vi "SubLanc.vi"(0 "Target Voltage, V":dbl=1.0 min=-4.0 max=4.0 step=0.1 format="%.4f", 2 "Sweep rate, V/min":dbl=0.1 min=0.0 max=1.0 step=0.01 format="%.4f", 3 "Custom Folder":string, 5 "optional Bias (V)":dbl=1e-08) -> ()   [LabVIEW 2015]
uses:
  <vilib>/Utility/file.llb/Write To Spreadsheet File (DBL).vi
panel:
  out "Numeric 4":i32
  in  "Commutator":bool
  in  "Commute SorceMeter":enum32{"Radio Selection 1", "Radio Selection 2"}(radio)
  out "Numeric 3":i32
  in  "Channel 2 (Vnano3b)":bool
  in  "Channel 1 (Vnano3)":bool
  out "Numeric":i32
  in  "Capacitance (C) and Loss (L)":bool
  in  "Magnetic Field (B)":bool
  in  "Current (Ik3)":bool
  in  "Voltage (Vk3)":bool
  in  "Current (Ik2)":bool
  in  "Voltage (Vk2)":bool
  in  "Channel 2 (Vnano2b)":bool
  in  "Channel 1 (Vnano2)":bool
  in  "Thermometer 1 (T1)":bool=TRUE
  in  "Channel 2 (Vnano1b)":bool
  in  "Channel 1 (Vnano1)":bool
  in  "Current (Ik1)":bool=TRUE
  in  "Voltage (Vk1)":bool
  out "Numeric Current":dbl
  out "Main Keithly2614B address":string="12"
  out "Delib Time delay":i32
  in  "points at each Vg":i32=1
  out "XY Graph":cluster{dbl[], dbl[]}(graph)={[1.0, 0.8, 0.6000000000000001, 0.4000000000000001, 0.20000000000000007, 5.551115123125783e-17, -0.19999999999999996, -0.39999999999999997, -0.6, -0.8, -1.0], [0.03352775, 0.056811, 0.03911575, 0.04330675, -0.02468015, 0.011641600000000002, 0.10151450000000001, 0.12386675000000001, 0.08288825000000001, -0.00186266, -0.038650000000000004]}
  in  "Time btw \npoints, sec":dbl=1.0 format="%.2f"
  out "Array 2":dbl[][](array[numeric])
  out "array for data":dbl[](array[numeric])
  out "Numeric 2":dbl
  out "Array":string[](array[string])
  in  "Addr 1 lock-in oop":bool
  in  "Ring":u16(ring) caption="Y-axis:" items=["Vg", "I", "R1", "R1oop", "Ik1", "T1"]
  out "String":string
  out "Data file:":path
  in  "Set compliance limit, mkA":dbl=0.05 min=0.0 max=1.0 step=0.01 format="%.3f"
  in  "error in (no error)":errorcluster
  in  "Ring 3":u16(ring)=1 items=["1 kOhm", "10 kOhm", "100 kOhm", "1 Mohm", "10 mOhm"]
  in  "Ring 2":u16(ring)=3 items=["1 kOhm", "10 kOhm", "100 kOhm", "1 Mohm", "10 mOhm"]
  in  "Fixed Current mkA":dbl=1.0
  in  "Current is:":T1(radio)
  in  "Ressitance measurements?":bool=TRUE
  in  "Addr 5 lock-in oop":bool
  in  "Addr 4 lock-in oop":bool
  in  "Addr 3 lock-in oop":bool
  in  "Addr 2 lock-in oop":bool
  in  "Addr 5 lock-in":bool
  in  "Addr 4 lock-in":bool
  in  "Addr 3 lock-in":bool=TRUE
  in  "Addr 2 lock-in":bool=TRUE
  in  "Addr 1 lock-in":bool=TRUE
  # "Keithley 2400: address 12"
  # "0"
  # "SourceMeters"
  # "Nanovoltmeters"
  # "Temperature"
  # "Main"
  # "Magnetic Field"
  # "(not recommended, too slow)"
  # "Capacitance & Loss"
  # "(not recommended, too slow)"
  # "(not recommended, too slow)"
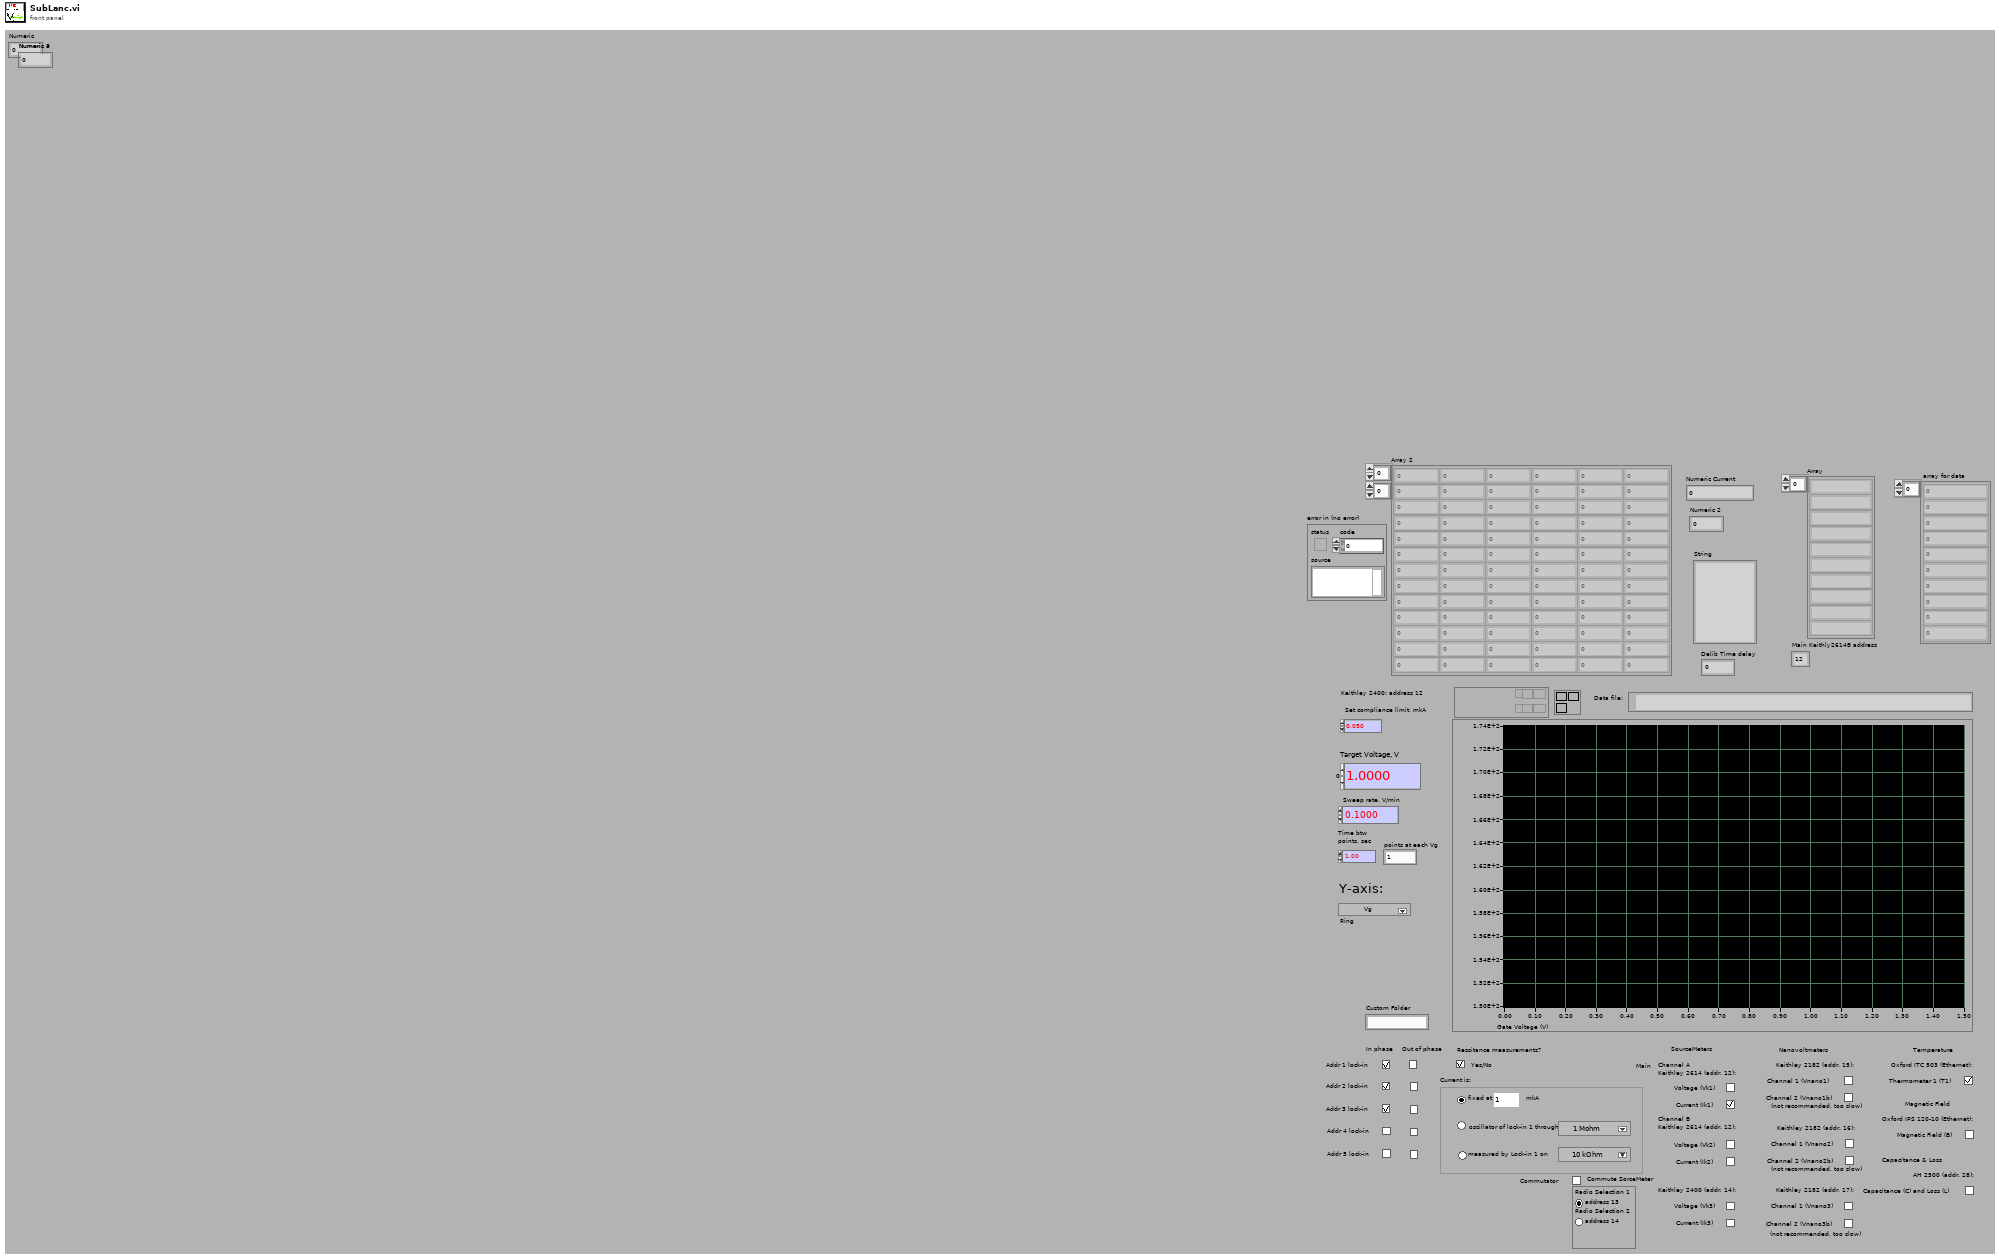
[diagram p1: front panel]
types:
  T1 = enum32{"Radio Selection 1", "Radio Selection 2", "Radio Selection 3"}
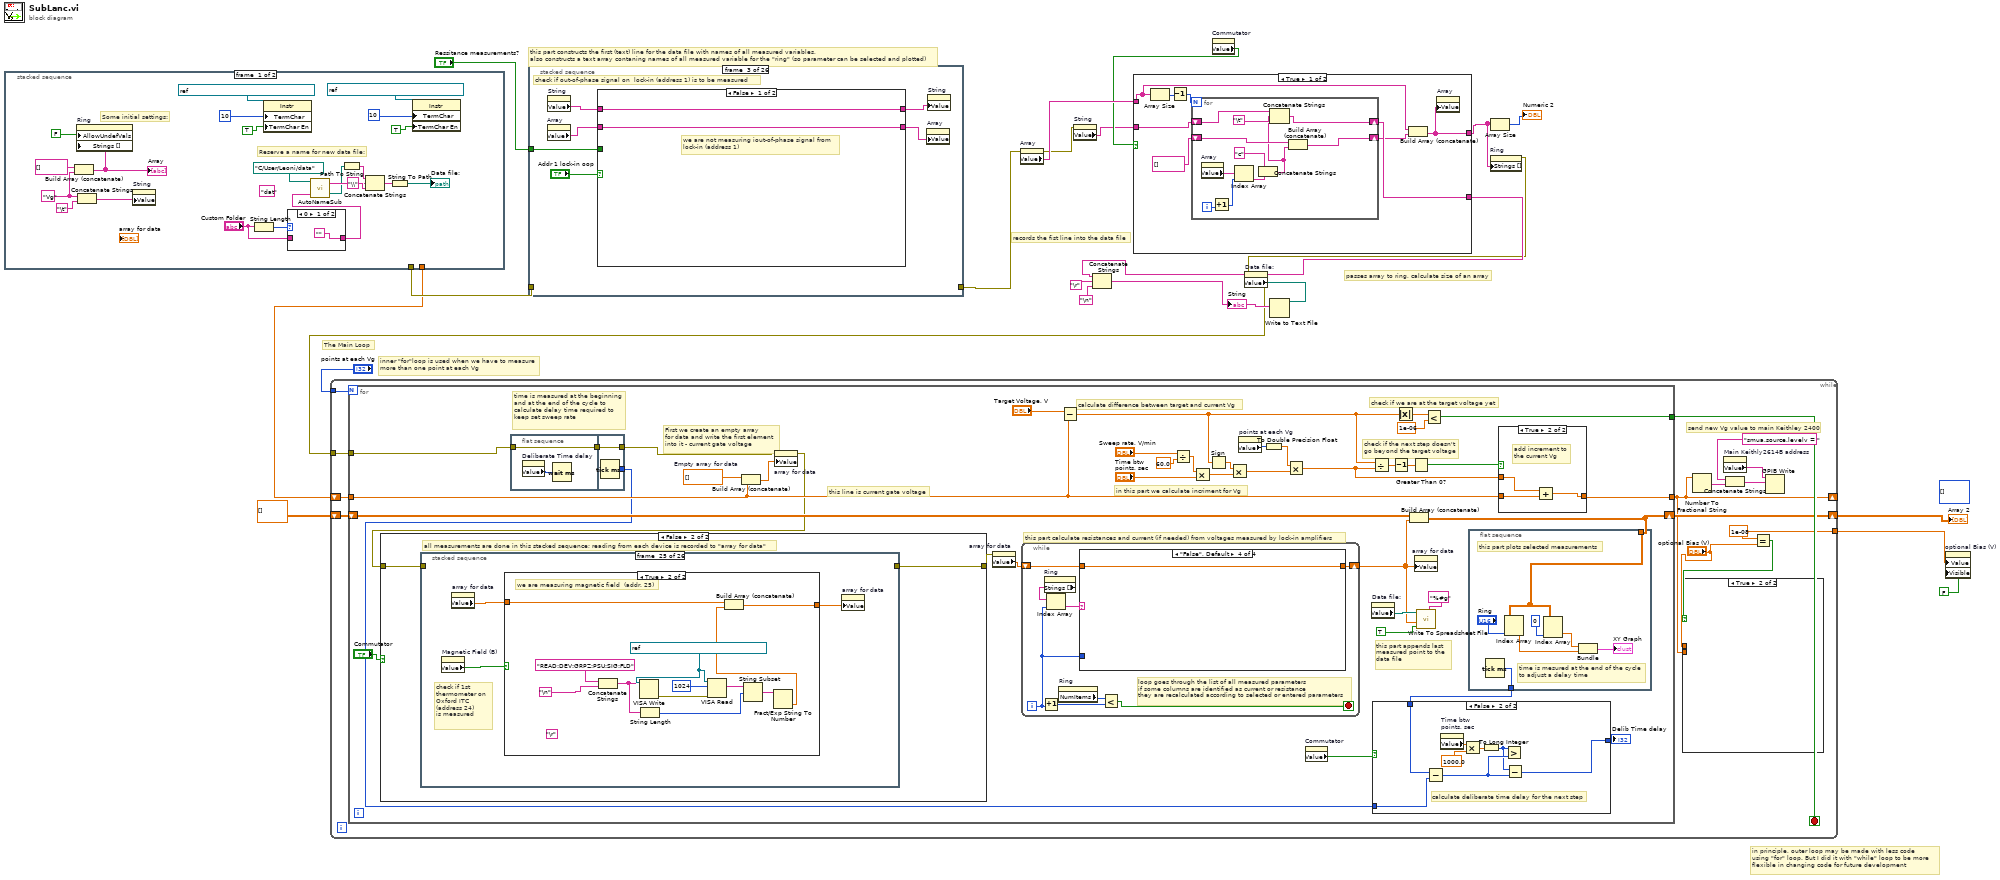
[diagram p0: block diagram]
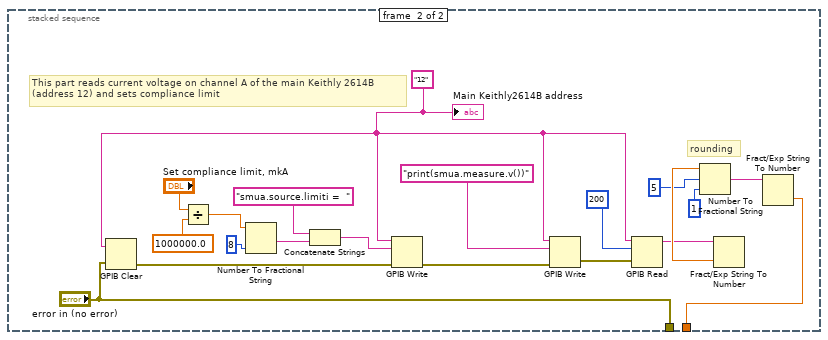
[diagram p4: hidden frame]
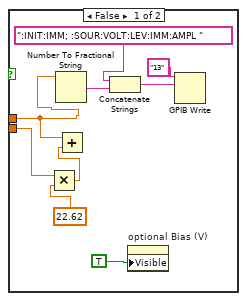
[diagram p5: hidden frame]
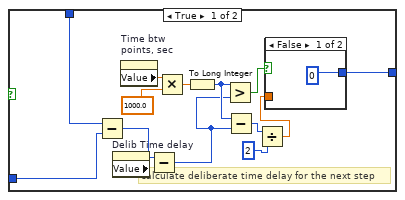
[diagram p6: hidden frame]
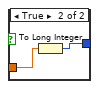
[diagram p7: hidden frame]
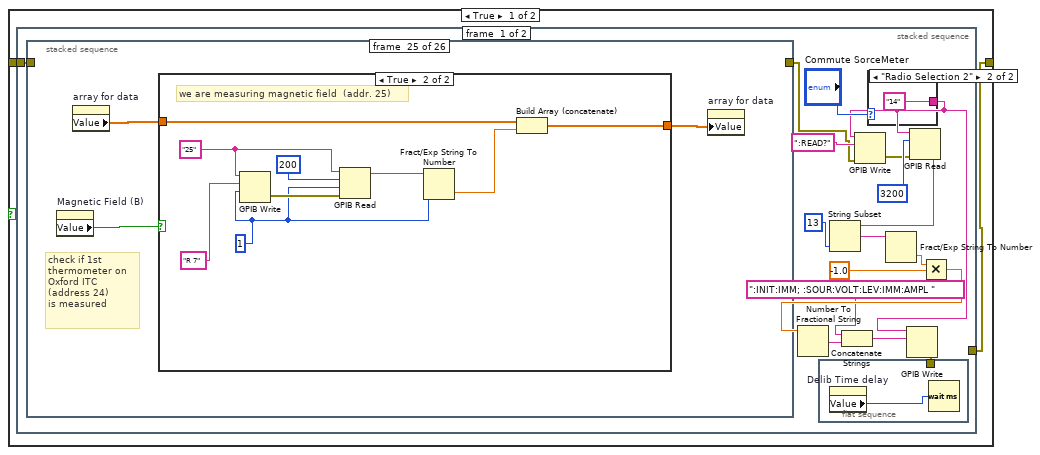
[diagram p8: hidden frame]
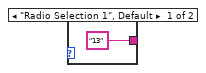
[diagram p9: hidden frame]
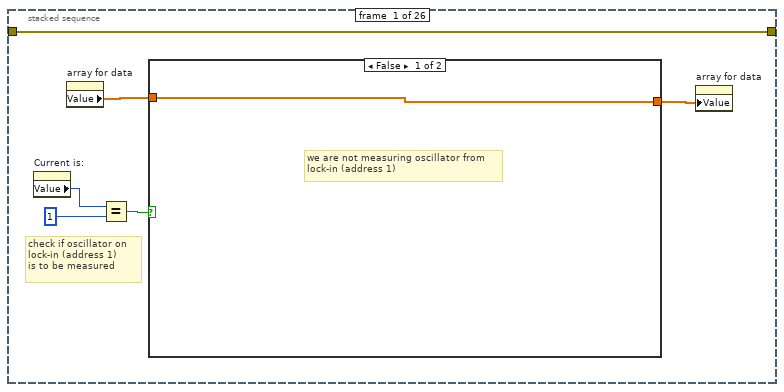
[diagram p10: hidden frame]
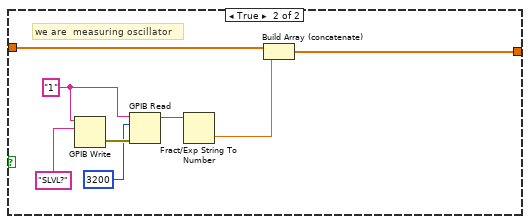
[diagram p11: hidden frame]
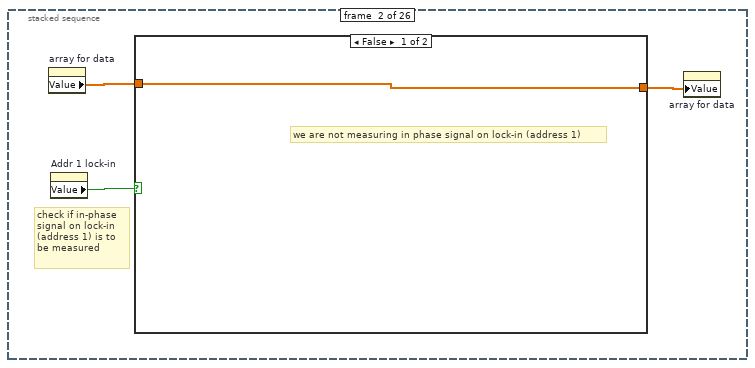
[diagram p12: hidden frame]
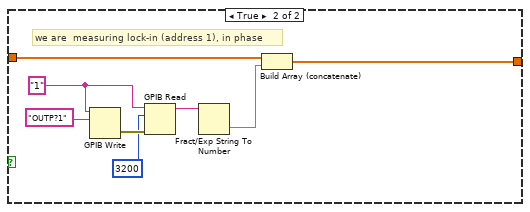
[diagram p13: hidden frame]
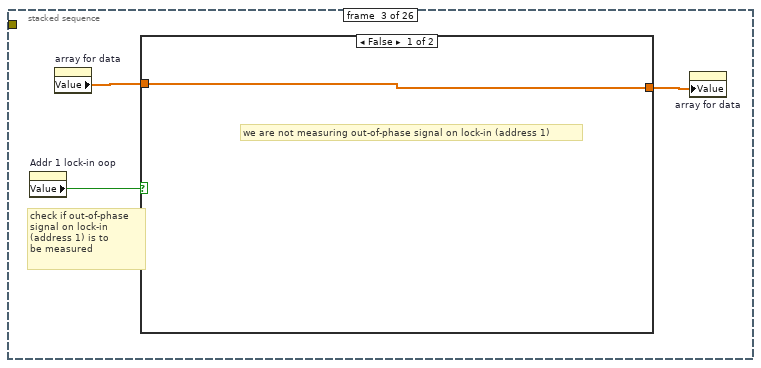
[diagram p14: hidden frame]
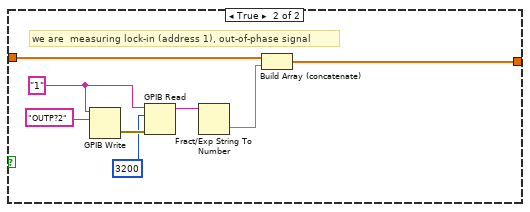
[diagram p15: hidden frame]
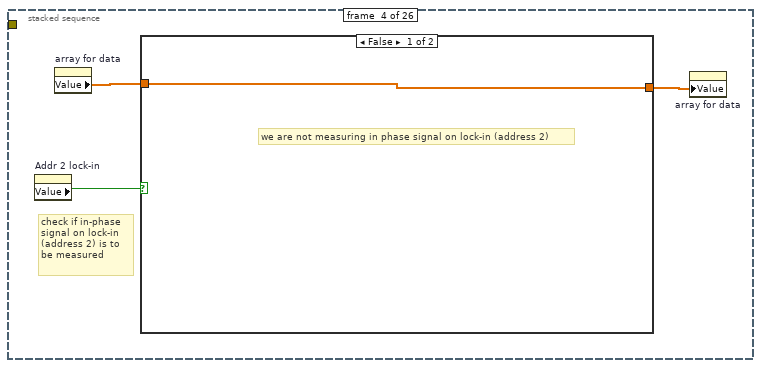
[diagram p16: hidden frame]
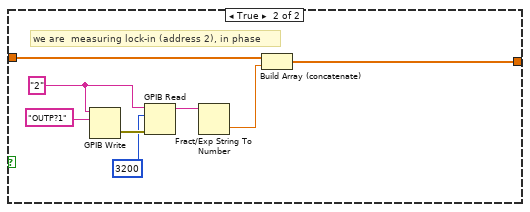
[diagram p17: hidden frame]
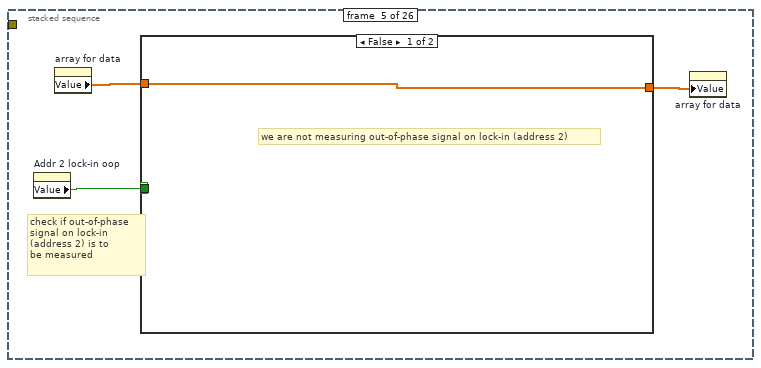
[diagram p18: hidden frame]
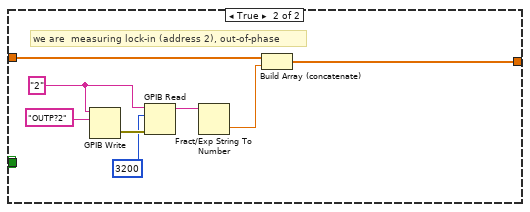
[diagram p19: hidden frame]
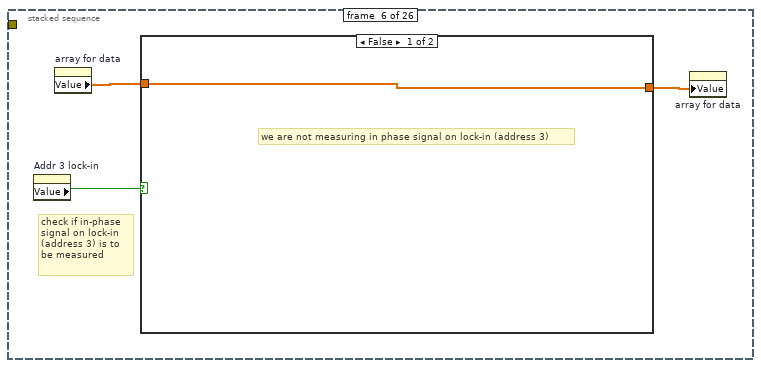
[diagram p20: hidden frame]
diagram:
  (unwired) i32[][] []
  # "passes array to ring, calculate size of an array"
  # "in principle, outer loop may be made with less code\nusing \"for\" loop. But I did it with \"while\" loop to be more \nflexible in changing code for future development"
  # "inner \"for\"loop is used when we have to measure\nmore than one point at each Vg"
  # "The Main Loop"
  # "records the fist line into the data file"
  # "this part constructs the first (text) line for the data file with names of all measured variables,\nalso constructs a text array contaning names of all measured variable for the \"ring\" (so parameter can be selected and plotted)"
  n1 = stacked-sequence {
    tunnel: [_ "error in (no error)"] -> w22
    tunnel: [_ w47] -> w9
    frame #0 {
      (unwired) "dat"
      w34 = "Vg"
      # "Some initial settings:"
      # "Reserve a name for new data file:"
      n2 = Build Array (concatenate)(string[] [], w34) -> (w36:string[])
      "Array" <- w36
      n3 = property on="Ring" class="Ring (strict)"("AllowUndefVals"=FALSE, "Strings []"=w36) -> ()  [unwired: 2 in, 2 out]
      n4 = Concatenate Strings(w34, "\t") -> (w35:string)
      n5 = property on="String" class="Str"("Value"=w35) -> ()  [unwired: 2 in, 2 out]
      n6 = String Length(string="Custom Folder") -> (length=w31:i32)
      n7 = property class="Instr"(reference=refnum<visa-resource-name> "TCPIP0::192.168.128.3::7020::SOCKET" ("VISA resource name"), "TermChar"=10, "TermChar En"=TRUE) -> ()  [unwired: 1 in, 2 out]
      n8 = case shown="0" w31 {
        tunnel: "Custom Folder" -> [_ w46]
        tunnel: ["" w46] -> w29
        frame 0 {
        }
        frame 1, Default {
        }
      }
      n9 = call "AutoNameSub.vi"("Custom Folder"=w29, "User Data Folder"=path "C:/User/Leoni/data") -> ("created path"=w43:path, "String"=w44:string)  [unwired: 1 in]
      n10 = Path To String(path=w43) -> (string=w38:string)
      n11 = Concatenate Strings(w38, "\\", w44) -> (w40:string)
      n12 = String To Path(string=w40) -> (path=→"Data file:":path)
      n13 = property class="Instr"(reference=refnum<visa-resource-name> "TCPIP0::192.168.128.2::7020::SOCKET" ("VISA resource name"), "TermChar"=10, "TermChar En"=TRUE) -> ()  [unwired: 1 in, 2 out]
    }
    frame #1 {
      w54 = "12"
      # "rounding"
      # "This part reads current voltage on channel A of the main Keithly 2614B \n(address 12) and sets compliance limit"
      n14 = GPIB Clear(2:"error in (no error)", 3:w54) -> (0:w59:errorcluster)  [unwired: 1 out]
      n15 = Divide(x="Set compliance limit, mkA", y=1000000.0) -> (x/y=w65:dbl)
      n16 = Number To Fractional String(number=w65, precision (6)=i16 8) -> (F-format string=w61:string)  [unwired: 2 in]
      n17 = Concatenate Strings("smua.source.limiti =  " ("data"), w61) -> (w60:string)
      n18 = GPIB Write(0:w54, 1:w60, 3:w59) -> (6:w55:errorcluster)  [unwired: 2 in, 1 out]
      n19 = GPIB Write(0:w54, 1:"print(smua.measure.v())" ("data"), 3:w55) -> (6:w58:errorcluster)  [unwired: 2 in, 1 out]
      n20 = GPIB Read(0:w54, 1:200 ("byte count"), 3:w58) -> (5:w48:string)  [unwired: 2 in, 2 out]
      n21 = Fract/Exp String To Number(string=w48) -> (number=w52:dbl)  [unwired: 3 in, 1 out]
      n22 = Number To Fractional String(number=w52, width (-)=5, precision (6)=1) -> (F-format string=w49:string)  [unwired: 1 in]
      n23 = Fract/Exp String To Number(string=w49) -> (number=w47:dbl)  [unwired: 3 in, 1 out]
      "Main Keithly2614B address" <- w54
    }
  }
  n24 = stacked-sequence {
    tunnel: "Ressitance measurements?" -> [w74 w89 w113 w136 w154 w172 w190 w208 w226 w244 w262 _ _ _ _ _ _ _ _ _ _ _ _ _ _ _]
    tunnel: w22 -> [_ w86 _ _ _ _ _ _ _ _ _ _ _ _ _ _ _ _ _ _ _ _ _ _ _ _]
    tunnel: [_ w86 _ _ _ _ _ _ _ _ _ _ _ _ _ _ _ _ _ _ _ _ _ _ _ _] -> w19
    frame #0 {
      # "check if oscillator of  lock-in (address 1) is to be measured"
      n25 = property on="Array" class="Arr (strict)"() -> ("Value"=w69:string[])  [unwired: 2 in, 2 out]
      n26 = property on="String" class="Str"() -> ("Value"=w73:string)  [unwired: 2 in, 2 out]
      n27 = Equal?(x="Current is:", y=1) -> (x = y?=w70:bool)
      n28 = case shown="True" w70 {
        tunnel: w74 -> [_ _]
        tunnel: [w76 w77] -> w72
        tunnel: w73 -> [w76 w80]
        tunnel: w69 -> [w75 w79]
        tunnel: [w75 w78] -> w68
        frame False {
          # "we are not measuring oscillator from\nlock-in (address 1)"
        }
        frame True {
          w81 = "I"
          # "we are  measuring oscillator"
          n29 = GPIB Clear(3:"1") -> ()  [unwired: 1 in, 2 out]
          n30 = Concatenate Strings(w80, w81, "\t") -> (w77:string)
          n31 = Build Array (concatenate)(w79, w81) -> (w78:string[])
        }
      }
      n32 = property on="Array" class="Arr (strict)"("Value"=w68) -> ()  [unwired: 2 in, 2 out]
      n33 = property on="String" class="Str"("Value"=w72) -> ()  [unwired: 2 in, 2 out]
    }
    frame #1 {
      # "check if lock-in (address 1) is to be measured"
      n34 = property on="Array" class="Arr (strict)"() -> ("Value"=w85:string[])  [unwired: 2 in, 2 out]
      n35 = property on="String" class="Str"() -> ("Value"=w88:string)  [unwired: 2 in, 2 out]
      n36 = case shown="False" "Addr 1 lock-in" {
        tunnel: w89 -> [_ w100]
        tunnel: [w92 w96] -> w87
        tunnel: w88 -> [w92 w95]
        tunnel: w85 -> [w91 w97]
        tunnel: [w91 w98] -> w84
        frame False {
          # "we are not measuring in phase signal from\nlock-in (address 1)"
        }
        frame True {
          # "are we measuring resistance?"
          n37 = GPIB Clear(3:"1") -> ()  [unwired: 1 in, 2 out]
          n38 = case shown="True" w100 {
            tunnel: ["V1" w102] -> w93
            frame False {
              # "no, we are not measuring resistanse;\nall lock-ins are measuring voltage"
            }
            frame True {
              # "are we measuring current as well?"
              n39 = property on="Current is:" class="RadioBtnsControl (strict)"() -> ("Value"=w104:T1)  [unwired: 2 in, 2 out]
              n40 = Equal?(x=w104, y=2) -> (x = y?=w105:bool)
              n41 = case shown="False" w105 {
                tunnel: ["R1" "I"] -> w102
                frame False {
                  # "no, we are not \nmeasuring current\nby lock-in \n(address 1); \nso this lock-in is \nmeasuring resistance"
                }
                frame True {
                  # "yes, we are measuring \ncurrent by lock-in \n(address 1) as \nvoltage drop on \nknown resistance"
                }
              }
            }
          }
          n42 = Concatenate Strings(w95, w93, "\t") -> (w96:string)
          n43 = Build Array (concatenate)(w97, w93) -> (w98:string[])
        }
      }
      n44 = property on="Array" class="Arr (strict)"("Value"=w84) -> ()  [unwired: 2 in, 2 out]
      n45 = property on="String" class="Str"("Value"=w87) -> ()  [unwired: 2 in, 2 out]
    }
    frame #2 {
      # "check if out-of-phase signal on  lock-in (address 1) is to be measured"
      n46 = property on="Array" class="Arr (strict)"() -> ("Value"=w110:string[])  [unwired: 2 in, 2 out]
      n47 = property on="String" class="Str"() -> ("Value"=w112:string)  [unwired: 2 in, 2 out]
      n48 = case shown="False" "Addr 1 lock-in oop" {
        tunnel: w113 -> [_ w123]
        tunnel: [w115 w119] -> w111
        tunnel: w112 -> [w115 w118]
        tunnel: w110 -> [w114 w120]
        tunnel: [w114 w121] -> w109
        frame False {
          # "we are not measuring iout-of-phase signal from\nlock-in (address 1)"
        }
        frame True {
          # "are we measuring resistance?"
          n49 = GPIB Clear(3:"1") -> ()  [unwired: 1 in, 2 out]
          n50 = case shown="True" w123 {
            tunnel: ["V1oop" w125] -> w116
            frame False {
              # "no, we are not measuring resistance;\nall lock-ins are measuring voltage"
            }
            frame True {
              # "are we measuring out-of-phase current as well?"
              n51 = property on="Current is:" class="RadioBtnsControl (strict)"() -> ("Value"=w127:T1)  [unwired: 2 in, 2 out]
              n52 = Equal?(x=w127, y=2) -> (x = y?=w128:bool)
              n53 = case shown="False" w128 {
                tunnel: ["R1oop" "Ioop"] -> w125
                frame False {
                  # "no, we are not \nmeasuring current\nby lock-in \n(address 1); so this \nlock-in is measuring\nout-of-phase resistance"
                }
                frame True {
                  # "yes, we are measuring \nout-of phase current \nby lock-in (address 1) \nas voltage drop on \nknown resistance"
                }
              }
            }
          }
          n54 = Concatenate Strings(w118, w116, "\t") -> (w119:string)
          n55 = Build Array (concatenate)(w120, w116) -> (w121:string[])
        }
      }
      n56 = property on="Array" class="Arr (strict)"("Value"=w109) -> ()  [unwired: 2 in, 2 out]
      n57 = property on="String" class="Str"("Value"=w111) -> ()  [unwired: 2 in, 2 out]
    }
    frame #3 {
      # "check if in-phase signal on  lock-in (address 2) is to be measured"
      n58 = property on="Array" class="Arr (strict)"() -> ("Value"=w133:string[])  [unwired: 2 in, 2 out]
      n59 = property on="String" class="Str"() -> ("Value"=w135:string)  [unwired: 2 in, 2 out]
      n60 = case shown="False" "Addr 2 lock-in" {
        tunnel: w136 -> [_ w146]
        tunnel: [w138 w142] -> w134
        tunnel: w135 -> [w138 w141]
        tunnel: w133 -> [w137 w143]
        tunnel: [w137 w144] -> w132
        frame False {
          # "we are not measuring in-phase signal from\nlock-in (address 2)"
        }
        frame True {
          # "are we measuring resistance?"
          n61 = GPIB Clear(3:"2") -> ()  [unwired: 1 in, 2 out]
          n62 = case shown="True" w146 {
            tunnel: ["R2" "V2"] -> w139
            frame True {
              # "we are measuring \nresistance by lock-in \n(address 2)"
            }
            frame False, Default {
              # "no, we are not measuring resistance;\nall lock-ins are measuring voltage"
            }
          }
          n63 = Concatenate Strings(w141, w139, "\t") -> (w142:string)
          n64 = Build Array (concatenate)(w143, w139) -> (w144:string[])
        }
      }
      n65 = property on="Array" class="Arr (strict)"("Value"=w132) -> ()  [unwired: 2 in, 2 out]
      n66 = property on="String" class="Str"("Value"=w134) -> ()  [unwired: 2 in, 2 out]
    }
    frame #4 {
      # "check if out-of-phase signal on  lock-in (address 2) is to be measured"
      n67 = property on="Array" class="Arr (strict)"() -> ("Value"=w151:string[])  [unwired: 2 in, 2 out]
      n68 = property on="String" class="Str"() -> ("Value"=w153:string)  [unwired: 2 in, 2 out]
      n69 = case shown="False" "Addr 2 lock-in oop" {
        tunnel: w154 -> [_ w164]
        tunnel: [w156 w160] -> w152
        tunnel: w153 -> [w156 w159]
        tunnel: w151 -> [w155 w161]
        tunnel: [w155 w162] -> w150
        frame False {
          # "we are not measuring out-of-phase signal from\nlock-in (address 2)"
        }
        frame True {
          # "are we measuring resistance?"
          n70 = GPIB Clear(3:"2") -> ()  [unwired: 1 in, 2 out]
          n71 = case shown="True" w164 {
            tunnel: ["R2oop" "V2oop"] -> w157
            frame True {
              # "we are measuring out-of-phase resistance by lock-in (address 2)\n(address 2)"
            }
            frame False, Default {
              # "no, we are not measuring resistance;\nall lock-ins are measuring voltage"
            }
          }
          n72 = Concatenate Strings(w159, w157, "\t") -> (w160:string)
          n73 = Build Array (concatenate)(w161, w157) -> (w162:string[])
        }
      }
      n74 = property on="Array" class="Arr (strict)"("Value"=w150) -> ()  [unwired: 2 in, 2 out]
      n75 = property on="String" class="Str"("Value"=w152) -> ()  [unwired: 2 in, 2 out]
    }
    frame #5 {
      # "check if in-phase signal on  lock-in (address 3) is to be measured"
      n76 = property on="Array" class="Arr (strict)"() -> ("Value"=w169:string[])  [unwired: 2 in, 2 out]
      n77 = property on="String" class="Str"() -> ("Value"=w171:string)  [unwired: 2 in, 2 out]
      n78 = case shown="False" "Addr 3 lock-in" {
        tunnel: w172 -> [_ w182]
        tunnel: [w174 w178] -> w170
        tunnel: w171 -> [w174 w177]
        tunnel: w169 -> [w173 w179]
        tunnel: [w173 w180] -> w168
        frame False {
          # "we are not measuring in-phase signal from\nlock-in (address 3)"
        }
        frame True {
          # "are we measuring resistance?"
          n79 = GPIB Clear(3:"3") -> ()  [unwired: 1 in, 2 out]
          n80 = case shown="True" w182 {
            tunnel: ["R3" "V3"] -> w175
            frame True {
              # "we are measuring \nresistance by lock-in \n(address 3)"
            }
            frame False, Default {
              # "no, we are not measuring resistance;\nall lock-ins are measuring voltage"
            }
          }
          n81 = Concatenate Strings(w177, w175, "\t") -> (w178:string)
          n82 = Build Array (concatenate)(w179, w175) -> (w180:string[])
        }
      }
      n83 = property on="Array" class="Arr (strict)"("Value"=w168) -> ()  [unwired: 2 in, 2 out]
      n84 = property on="String" class="Str"("Value"=w170) -> ()  [unwired: 2 in, 2 out]
    }
    frame #6 {
      # "check if out-of-phase signal on  lock-in (address 3) is to be measured"
      n85 = property on="Array" class="Arr (strict)"() -> ("Value"=w187:string[])  [unwired: 2 in, 2 out]
      n86 = property on="String" class="Str"() -> ("Value"=w189:string)  [unwired: 2 in, 2 out]
      n87 = case shown="False" "Addr 3 lock-in oop" {
        tunnel: w190 -> [_ w200]
        tunnel: [w192 w196] -> w188
        tunnel: w189 -> [w192 w195]
        tunnel: w187 -> [w191 w197]
        tunnel: [w191 w198] -> w186
        frame False {
          # "we are not measuring out-of-phase signal from\nlock-in (address 3)"
        }
        frame True {
          # "are we measuring resistance?"
          n88 = GPIB Clear(3:"3") -> ()  [unwired: 1 in, 2 out]
          n89 = case shown="True" w200 {
            tunnel: ["R3oop" "V3oop"] -> w193
            frame True {
              # "we are measuring out-of-phase resistance by lock-in (address 3)\n(address 2)"
            }
            frame False, Default {
              # "no, we are not measuring resistance;\nall lock-ins are measuring voltage"
            }
          }
          n90 = Concatenate Strings(w195, w193, "\t") -> (w196:string)
          n91 = Build Array (concatenate)(w197, w193) -> (w198:string[])
        }
      }
      n92 = property on="Array" class="Arr (strict)"("Value"=w186) -> ()  [unwired: 2 in, 2 out]
      n93 = property on="String" class="Str"("Value"=w188) -> ()  [unwired: 2 in, 2 out]
    }
    frame #7 {
      # "check if in-phase signal on  lock-in (address 4) is to be measured"
      n94 = property on="Array" class="Arr (strict)"() -> ("Value"=w205:string[])  [unwired: 2 in, 2 out]
      n95 = property on="String" class="Str"() -> ("Value"=w207:string)  [unwired: 2 in, 2 out]
      n96 = case shown="False" "Addr 4 lock-in" {
        tunnel: w208 -> [_ w218]
        tunnel: [w210 w214] -> w206
        tunnel: w207 -> [w210 w213]
        tunnel: w205 -> [w209 w215]
        tunnel: [w209 w216] -> w204
        frame False {
          # "we are not measuring in-phase signal from\nlock-in (address 4)"
        }
        frame True {
          # "are we measuring resistance?"
          n97 = GPIB Clear(3:"4") -> ()  [unwired: 1 in, 2 out]
          n98 = case shown="True" w218 {
            tunnel: ["R4" "V4"] -> w211
            frame True {
              # "we are measuring \nresistance by lock-in \n(address 4)"
            }
            frame False, Default {
              # "no, we are not measuring resistance;\nall lock-ins are measuring voltage"
            }
          }
          n99 = Concatenate Strings(w213, w211, "\t") -> (w214:string)
          n100 = Build Array (concatenate)(w215, w211) -> (w216:string[])
        }
      }
      n101 = property on="Array" class="Arr (strict)"("Value"=w204) -> ()  [unwired: 2 in, 2 out]
      n102 = property on="String" class="Str"("Value"=w206) -> ()  [unwired: 2 in, 2 out]
    }
    frame #8 {
      # "check if out-of-phase signal on  lock-in (address 4) is to be measured"
      n103 = property on="Array" class="Arr (strict)"() -> ("Value"=w223:string[])  [unwired: 2 in, 2 out]
      n104 = property on="String" class="Str"() -> ("Value"=w225:string)  [unwired: 2 in, 2 out]
      n105 = case shown="False" "Addr 4 lock-in oop" {
        tunnel: w226 -> [_ w236]
        tunnel: [w228 w232] -> w224
        tunnel: w225 -> [w228 w231]
        tunnel: w223 -> [w227 w233]
        tunnel: [w227 w234] -> w222
        frame False {
          # "we are not measuring out-of-phase signal from\nlock-in (address 4)"
        }
        frame True {
          # "are we measuring resistance?"
          n106 = GPIB Clear(3:"4") -> ()  [unwired: 1 in, 2 out]
          n107 = case shown="True" w236 {
            tunnel: ["R4oop" "V4oop"] -> w229
            frame True {
              # "we are measuring out-of-phase resistance by lock-in (address 4)\n(address 2)"
            }
            frame False, Default {
              # "no, we are not measuring resistance;\nall lock-ins are measuring voltage"
            }
          }
          n108 = Concatenate Strings(w231, w229, "\t") -> (w232:string)
          n109 = Build Array (concatenate)(w233, w229) -> (w234:string[])
        }
      }
      n110 = property on="Array" class="Arr (strict)"("Value"=w222) -> ()  [unwired: 2 in, 2 out]
      n111 = property on="String" class="Str"("Value"=w224) -> ()  [unwired: 2 in, 2 out]
    }
    frame #9 {
      # "check if in-phase signal on  lock-in (address 5) is to be measured"
      n112 = property on="Array" class="Arr (strict)"() -> ("Value"=w241:string[])  [unwired: 2 in, 2 out]
      n113 = property on="String" class="Str"() -> ("Value"=w243:string)  [unwired: 2 in, 2 out]
      n114 = case shown="False" "Addr 5 lock-in" {
        tunnel: w244 -> [_ w254]
        tunnel: [w246 w250] -> w242
        tunnel: w243 -> [w246 w249]
        tunnel: w241 -> [w245 w251]
        tunnel: [w245 w252] -> w240
        frame False {
          # "we are not measuring in-phase signal from\nlock-in (address 5)"
        }
        frame True {
          # "are we measuring resistance?"
          n115 = GPIB Clear(3:"5") -> ()  [unwired: 1 in, 2 out]
          n116 = case shown="True" w254 {
            tunnel: ["R5" "V5"] -> w247
            frame True {
              # "we are measuring \nresistance by lock-in \n(address 5)"
            }
            frame False, Default {
              # "no, we are not measuring resistance;\nall lock-ins are measuring voltage"
            }
          }
          n117 = Concatenate Strings(w249, w247, "\t") -> (w250:string)
          n118 = Build Array (concatenate)(w251, w247) -> (w252:string[])
        }
      }
      n119 = property on="Array" class="Arr (strict)"("Value"=w240) -> ()  [unwired: 2 in, 2 out]
      n120 = property on="String" class="Str"("Value"=w242) -> ()  [unwired: 2 in, 2 out]
    }
    frame #10 {
      # "check if out-of-phase signal on  lock-in (address 5) is to be measured"
      n121 = property on="Array" class="Arr (strict)"() -> ("Value"=w259:string[])  [unwired: 2 in, 2 out]
      n122 = property on="String" class="Str"() -> ("Value"=w261:string)  [unwired: 2 in, 2 out]
      n123 = case shown="False" "Addr 5 lock-in oop" {
        tunnel: w262 -> [_ w272]
        tunnel: [w264 w268] -> w260
        tunnel: w261 -> [w264 w267]
        tunnel: w259 -> [w263 w269]
        tunnel: [w263 w270] -> w258
        frame False {
          # "we are not measuring out-of-phase signal from\nlock-in (address 5)"
        }
        frame True {
          # "are we measuring resistance?"
          n124 = GPIB Clear(3:"5") -> ()  [unwired: 1 in, 2 out]
          n125 = case shown="True" w272 {
            tunnel: ["R5oop" "V5oop"] -> w265
            frame True {
              # "we are measuring out-of-phase resistance by lock-in (address 5)\n(address 2)"
            }
            frame False, Default {
              # "no, we are not measuring resistance;\nall lock-ins are measuring voltage"
            }
          }
          n126 = Concatenate Strings(w267, w265, "\t") -> (w268:string)
          n127 = Build Array (concatenate)(w269, w265) -> (w270:string[])
        }
      }
      n128 = property on="Array" class="Arr (strict)"("Value"=w258) -> ()  [unwired: 2 in, 2 out]
      n129 = property on="String" class="Str"("Value"=w260) -> ()  [unwired: 2 in, 2 out]
    }
    frame #11 {
      # "check if voltage on main Keithley 2400 (addr. 12) is measured"
      n130 = property on="Array" class="Arr (strict)"() -> ("Value"=w277:string[])  [unwired: 2 in, 2 out]
      n131 = property on="String" class="Str"() -> ("Value"=w279:string)  [unwired: 2 in, 2 out]
      n132 = case shown="False" "Voltage (Vk1)" {
        tunnel: [w281 w285] -> w278
        tunnel: w279 -> [w281 w284]
        tunnel: w277 -> [w280 w286]
        tunnel: [w280 w287] -> w276
        frame False {
          # "no , we aren't measuring voltage \non main Keithley 2400 (addr. 12)"
        }
        frame True {
          w282 = "Vk1"
          # "yes , we are measuring voltage \non main Keithley 2400 (addr. 12)"
          n133 = GPIB Clear(3:"12") -> ()  [unwired: 1 in, 2 out]
          n134 = Concatenate Strings(w284, w282, "\t") -> (w285:string)
          n135 = Build Array (concatenate)(w286, w282) -> (w287:string[])
        }
      }
      n136 = property on="String" class="Str"("Value"=w278) -> ()  [unwired: 2 in, 2 out]
      n137 = property on="Array" class="Arr (strict)"("Value"=w276) -> ()  [unwired: 2 in, 2 out]
    }
    frame #12 {
      # "check if current on main Keithley 2400 (addr. 12) is measured"
      n138 = property on="Array" class="Arr (strict)"() -> ("Value"=w291:string[])  [unwired: 2 in, 2 out]
      n139 = property on="String" class="Str"() -> ("Value"=w293:string)  [unwired: 2 in, 2 out]
      n140 = case shown="True" "Current (Ik1)" {
        tunnel: [w295 w299] -> w292
        tunnel: w293 -> [w295 w298]
        tunnel: w291 -> [w294 w300]
        tunnel: [w294 w301] -> w290
        frame False {
          # "no , we aren't measuring current\non main Keithley 2400 (addr. 12)"
        }
        frame True {
          w296 = "Ik1"
          # "yes , we are measuring current \non main Keithley 2400 (addr. 12)"
          n141 = GPIB Clear(3:"12") -> ()  [unwired: 1 in, 2 out]
          n142 = Concatenate Strings(w298, w296, "\t") -> (w299:string)
          n143 = Build Array (concatenate)(w300, w296) -> (w301:string[])
        }
      }
      n144 = property on="String" class="Str"("Value"=w292) -> ()  [unwired: 2 in, 2 out]
      n145 = property on="Array" class="Arr (strict)"("Value"=w290) -> ()  [unwired: 2 in, 2 out]
    }
    frame #13 {
      # "check if voltage on additional Keithley 2400 (addr. 13) is measured"
      n146 = property on="Array" class="Arr (strict)"() -> ("Value"=w305:string[])  [unwired: 2 in, 2 out]
      n147 = property on="String" class="Str"() -> ("Value"=w307:string)  [unwired: 2 in, 2 out]
      n148 = case shown="False" "Voltage (Vk2)" {
        tunnel: [w309 w313] -> w306
        tunnel: w307 -> [w309 w312]
        tunnel: w305 -> [w308 w314]
        tunnel: [w308 w315] -> w304
        frame False {
          # "no , we aren't measuring voltage \non Keithley 2400 (addr. 13)"
        }
        frame True {
          w310 = "Vk2"
          # "yes , we are measuring voltage \non Keithley 2400 (addr. 13)"
          n149 = GPIB Clear(3:"13") -> ()  [unwired: 1 in, 2 out]
          n150 = Concatenate Strings(w312, w310, "\t") -> (w313:string)
          n151 = Build Array (concatenate)(w314, w310) -> (w315:string[])
        }
      }
      n152 = property on="String" class="Str"("Value"=w306) -> ()  [unwired: 2 in, 2 out]
      n153 = property on="Array" class="Arr (strict)"("Value"=w304) -> ()  [unwired: 2 in, 2 out]
    }
    frame #14 {
      # "check if current on additional Keithley 2400 (addr. 13) is measured"
      n154 = property on="Array" class="Arr (strict)"() -> ("Value"=w319:string[])  [unwired: 2 in, 2 out]
      n155 = property on="String" class="Str"() -> ("Value"=w321:string)  [unwired: 2 in, 2 out]
      n156 = case shown="False" "Current (Ik2)" {
        tunnel: [w323 w327] -> w320
        tunnel: w321 -> [w323 w326]
        tunnel: w319 -> [w322 w328]
        tunnel: [w322 w329] -> w318
        frame False {
          # "no , we aren't measuring current\non Keithley 2400 (addr. 13)"
        }
        frame True {
          w324 = "Ik2"
          # "yes , we are measuring current \non Keithley 2400 (addr. 13)"
          n157 = GPIB Clear(3:"13") -> ()  [unwired: 1 in, 2 out]
          n158 = Concatenate Strings(w326, w324, "\t") -> (w327:string)
          n159 = Build Array (concatenate)(w328, w324) -> (w329:string[])
        }
      }
      n160 = property on="String" class="Str"("Value"=w320) -> ()  [unwired: 2 in, 2 out]
      n161 = property on="Array" class="Arr (strict)"("Value"=w318) -> ()  [unwired: 2 in, 2 out]
    }
    frame #15 {
      # "check if voltage on additional Keithley 2400 (addr. 14) is measured"
      n162 = property on="Array" class="Arr (strict)"() -> ("Value"=w333:string[])  [unwired: 2 in, 2 out]
      n163 = property on="String" class="Str"() -> ("Value"=w335:string)  [unwired: 2 in, 2 out]
      n164 = case shown="False" "Voltage (Vk3)" {
        tunnel: [w337 w341] -> w334
        tunnel: w335 -> [w337 w340]
        tunnel: w333 -> [w336 w342]
        tunnel: [w336 w343] -> w332
        frame False {
          # "no , we aren't measuring voltage \non Keithley 2400 (addr. 14)"
        }
        frame True {
          w338 = "Vk3"
          # "yes , we are measuring voltage \non Keithley 2400 (addr. 14)"
          n165 = GPIB Clear(3:"14") -> ()  [unwired: 1 in, 2 out]
          n166 = Concatenate Strings(w340, w338, "\t") -> (w341:string)
          n167 = Build Array (concatenate)(w342, w338) -> (w343:string[])
        }
      }
      n168 = property on="String" class="Str"("Value"=w334) -> ()  [unwired: 2 in, 2 out]
      n169 = property on="Array" class="Arr (strict)"("Value"=w332) -> ()  [unwired: 2 in, 2 out]
    }
    frame #16 {
      # "check if current on additional Keithley 2400 (addr. 14) is measured"
      n170 = property on="Array" class="Arr (strict)"() -> ("Value"=w347:string[])  [unwired: 2 in, 2 out]
      n171 = property on="String" class="Str"() -> ("Value"=w349:string)  [unwired: 2 in, 2 out]
      n172 = case shown="False" "Current (Ik3)" {
        tunnel: [w351 w355] -> w348
        tunnel: w349 -> [w351 w354]
        tunnel: w347 -> [w350 w356]
        tunnel: [w350 w357] -> w346
        frame False {
          # "no , we aren't measuring current\non Keithley 2400 (addr. 14)"
        }
        frame True {
          w352 = "Ik3"
          # "yes , we are measuring current \non Keithley 2400 (addr. 14)"
          n173 = GPIB Clear(3:"14") -> ()  [unwired: 1 in, 2 out]
          n174 = Concatenate Strings(w354, w352, "\t") -> (w355:string)
          n175 = Build Array (concatenate)(w356, w352) -> (w357:string[])
        }
      }
      n176 = property on="String" class="Str"("Value"=w348) -> ()  [unwired: 2 in, 2 out]
      n177 = property on="Array" class="Arr (strict)"("Value"=w346) -> ()  [unwired: 2 in, 2 out]
    }
    frame #17 {
      # "check if 1st channel of nanovoltmeter Keithley 2182 (addr. 15) is measured"
      n178 = property on="Array" class="Arr (strict)"() -> ("Value"=w361:string[])  [unwired: 2 in, 2 out]
      n179 = property on="String" class="Str"() -> ("Value"=w363:string)  [unwired: 2 in, 2 out]
      n180 = case shown="True" "Channel 1 (Vnano1)" {
        tunnel: [w365 w370] -> w362
        tunnel: w363 -> [w365 w369]
        tunnel: w361 -> [w364 w371]
        tunnel: [w364 w372] -> w360
        frame False {
          # "no , we are not measuring 1st channel\non Keithley 2182 (addr. 15)"
        }
        frame True {
          w367 = "Vnano1"
          # "yes , we are measuring 1st channel\non Keithley 2182 (addr. 15)"
          n181 = GPIB Clear(3:"15") -> ()  [unwired: 1 in, 2 out]
          n182 = Concatenate Strings(w369, w367, "\t") -> (w370:string)
          n183 = Build Array (concatenate)(w371, w367) -> (w372:string[])
        }
      }
      n184 = property on="String" class="Str"("Value"=w362) -> ()  [unwired: 2 in, 2 out]
      n185 = property on="Array" class="Arr (strict)"("Value"=w360) -> ()  [unwired: 2 in, 2 out]
    }
    frame #18 {
      # "check if 2nd channel of nanovoltmeter Keithley 2182 (addr. 15) is measured"
      n186 = property on="Array" class="Arr (strict)"() -> ("Value"=w375:string[])  [unwired: 2 in, 2 out]
      n187 = property on="String" class="Str"() -> ("Value"=w377:string)  [unwired: 2 in, 2 out]
      n188 = case shown="False" "Channel 2 (Vnano1b)" {
        tunnel: [w379 w383] -> w376
        tunnel: w377 -> [w379 w382]
        tunnel: w375 -> [w378 w384]
        tunnel: [w378 w385] -> w374
        frame False {
          # "no , we are not measuring 2nd channel\non Keithley 2182 (addr. 15)"
        }
        frame True {
          w380 = "Vnano1b"
          # "yes , we are measuring 2nd channel\non Keithley 2182 (addr. 15)"
          n189 = GPIB Clear(3:"15") -> ()  [unwired: 1 in, 2 out]
          n190 = Concatenate Strings(w382, w380, "\t") -> (w383:string)
          n191 = Build Array (concatenate)(w384, w380) -> (w385:string[])
        }
      }
      n192 = property on="String" class="Str"("Value"=w376) -> ()  [unwired: 2 in, 2 out]
      n193 = property on="Array" class="Arr (strict)"("Value"=w374) -> ()  [unwired: 2 in, 2 out]
    }
    frame #19 {
      # "check if 1st channel of nanovoltmeter Keithley 2182 (addr. 16) is measured"
      n194 = property on="Array" class="Arr (strict)"() -> ("Value"=w389:string[])  [unwired: 2 in, 2 out]
      n195 = property on="String" class="Str"() -> ("Value"=w391:string)  [unwired: 2 in, 2 out]
      n196 = case shown="True" "Channel 1 (Vnano2)" {
        tunnel: [w393 w398] -> w390
        tunnel: w391 -> [w393 w397]
        tunnel: w389 -> [w392 w399]
        tunnel: [w392 w400] -> w388
        frame False {
          # "no , we are not measuring 1st channel\non Keithley 2182 (addr. 16)"
        }
        frame True {
          w395 = "Vnano2"
          # "yes , we are measuring 1st channel\non Keithley 2182 (addr. 16)"
          n197 = GPIB Clear(3:"16") -> ()  [unwired: 1 in, 2 out]
          n198 = Concatenate Strings(w397, w395, "\t") -> (w398:string)
          n199 = Build Array (concatenate)(w399, w395) -> (w400:string[])
        }
      }
      n200 = property on="String" class="Str"("Value"=w390) -> ()  [unwired: 2 in, 2 out]
      n201 = property on="Array" class="Arr (strict)"("Value"=w388) -> ()  [unwired: 2 in, 2 out]
    }
    frame #20 {
      # "check if 2nd channel of nanovoltmeter Keithley 2182 (addr. 16) is measured"
      n202 = property on="Array" class="Arr (strict)"() -> ("Value"=w403:string[])  [unwired: 2 in, 2 out]
      n203 = property on="String" class="Str"() -> ("Value"=w405:string)  [unwired: 2 in, 2 out]
      n204 = case shown="False" "Channel 2 (Vnano2b)" {
        tunnel: [w407 w411] -> w404
        tunnel: w405 -> [w407 w410]
        tunnel: w403 -> [w406 w412]
        tunnel: [w406 w413] -> w402
        frame False {
          # "no , we are not measuring 2nd channel\non Keithley 2182 (addr. 16)"
        }
        frame True {
          w408 = "Vnano2b"
          # "yes , we are measuring 2nd channel\non Keithley 2182 (addr. 16)"
          n205 = GPIB Clear(3:"16") -> ()  [unwired: 1 in, 2 out]
          n206 = Concatenate Strings(w410, w408, "\t") -> (w411:string)
          n207 = Build Array (concatenate)(w412, w408) -> (w413:string[])
        }
      }
      n208 = property on="String" class="Str"("Value"=w404) -> ()  [unwired: 2 in, 2 out]
      n209 = property on="Array" class="Arr (strict)"("Value"=w402) -> ()  [unwired: 2 in, 2 out]
    }
    frame #21 {
      # "check if 1st channel of nanovoltmeter Keithley 2182 (addr. 17) is measured"
      n210 = property on="Array" class="Arr (strict)"() -> ("Value"=w417:string[])  [unwired: 2 in, 2 out]
      n211 = property on="String" class="Str"() -> ("Value"=w419:string)  [unwired: 2 in, 2 out]
      n212 = case shown="False" "Channel 1 (Vnano3)" {
        tunnel: [w421 w425] -> w418
        tunnel: w419 -> [w421 w424]
        tunnel: w417 -> [w420 w426]
        tunnel: [w420 w427] -> w416
        frame False {
          # "no , we are not measuring 1st channel\non Keithley 2182 (addr. 17)"
        }
        frame True {
          w422 = "Vnano3"
          # "yes , we are measuring 1st channel\non Keithley 2182 (addr. 17)"
          n213 = GPIB Clear(3:"17") -> ()  [unwired: 1 in, 2 out]
          n214 = Concatenate Strings(w424, w422, "\t") -> (w425:string)
          n215 = Build Array (concatenate)(w426, w422) -> (w427:string[])
        }
      }
      n216 = property on="String" class="Str"("Value"=w418) -> ()  [unwired: 2 in, 2 out]
      n217 = property on="Array" class="Arr (strict)"("Value"=w416) -> ()  [unwired: 2 in, 2 out]
    }
    frame #22 {
      # "check if 2nd channel of nanovoltmeter Keithley 2182 (addr. 16) is measured"
      n218 = property on="Array" class="Arr (strict)"() -> ("Value"=w431:string[])  [unwired: 2 in, 2 out]
      n219 = property on="String" class="Str"() -> ("Value"=w433:string)  [unwired: 2 in, 2 out]
      n220 = case shown="False" "Channel 2 (Vnano3b)" {
        tunnel: [w435 w439] -> w432
        tunnel: w433 -> [w435 w438]
        tunnel: w431 -> [w434 w440]
        tunnel: [w434 w441] -> w430
        frame False {
          # "no , we are not measuring 2nd channel\non Keithley 2182 (addr. 17)"
        }
        frame True {
          w436 = "Vnano3b"
          # "yes , we are measuring 2nd channel\non Keithley 2182 (addr. 17)"
          n221 = GPIB Clear(3:"17") -> ()  [unwired: 1 in, 2 out]
          n222 = Concatenate Strings(w438, w436, "\t") -> (w439:string)
          n223 = Build Array (concatenate)(w440, w436) -> (w441:string[])
        }
      }
      n224 = property on="String" class="Str"("Value"=w432) -> ()  [unwired: 2 in, 2 out]
      n225 = property on="Array" class="Arr (strict)"("Value"=w430) -> ()  [unwired: 2 in, 2 out]
    }
    frame #23 {
      # "check if 1st thermometer on Oxford ITC (address 24) is measured"
      n226 = property on="Array" class="Arr (strict)"() -> ("Value"=w445:string[])  [unwired: 2 in, 2 out]
      n227 = property on="String" class="Str"() -> ("Value"=w447:string)  [unwired: 2 in, 2 out]
      n228 = case shown="True" "Thermometer 1 (T1)" {
        tunnel: [w449 w453] -> w446
        tunnel: w447 -> [w449 w452]
        tunnel: w445 -> [w448 w454]
        tunnel: [w448 w455] -> w444
        frame False {
          # "no, we are not measuring temperature\non thermometer 1 (addr. 24)"
        }
        frame True {
          w450 = "T1"
          # "yes, we are measuring temperature,\nthermometer 1 (addr. 24)"
          n229 = GPIB Clear(3:"24") -> ()  [unwired: 1 in, 2 out]
          n230 = Concatenate Strings(w452, w450, "\t") -> (w453:string)
          n231 = Build Array (concatenate)(w454, w450) -> (w455:string[])
        }
      }
      n232 = property on="String" class="Str"("Value"=w446) -> ()  [unwired: 2 in, 2 out]
      n233 = property on="Array" class="Arr (strict)"("Value"=w444) -> ()  [unwired: 2 in, 2 out]
    }
    frame #24 {
      # "check if magnetic field from Oxford IPS 120 (address 25) is measured"
      n234 = property on="Array" class="Arr (strict)"() -> ("Value"=w459:string[])  [unwired: 2 in, 2 out]
      n235 = property on="String" class="Str"() -> ("Value"=w461:string)  [unwired: 2 in, 2 out]
      n236 = case shown="True" "Magnetic Field (B)" {
        tunnel: [w463 w467] -> w460
        tunnel: w461 -> [w463 w466]
        tunnel: w459 -> [w462 w468]
        tunnel: [w462 w469] -> w458
        frame False {
          # "no, we are not measuring magnetic field  (addr. 25)"
        }
        frame True {
          w464 = "B"
          # "yes, we are measuring magnetic field  (addr. 25)"
          n237 = GPIB Clear(3:"25") -> ()  [unwired: 1 in, 2 out]
          n238 = Concatenate Strings(w466, w464, "\t") -> (w467:string)
          n239 = Build Array (concatenate)(w468, w464) -> (w469:string[])
        }
      }
      n240 = property on="String" class="Str"("Value"=w460) -> ()  [unwired: 2 in, 2 out]
      n241 = property on="Array" class="Arr (strict)"("Value"=w458) -> ()  [unwired: 2 in, 2 out]
    }
    frame #25 {
      # "check if capacitance and loss from AH 2500 (address 28) are measured"
      n242 = property on="Array" class="Arr (strict)"() -> ("Value"=w473:string[])  [unwired: 2 in, 2 out]
      n243 = property on="String" class="Str"() -> ("Value"=w475:string)  [unwired: 2 in, 2 out]
      n244 = case shown="False" "Capacitance (C) and Loss (L)" {
        tunnel: [w477 w486] -> w474
        tunnel: w475 -> [w477 w479]
        tunnel: w473 -> [w476 w481]
        tunnel: [w476 w487] -> w472
        frame False {
          # "no, we are not measuring capacitance  (addr. 28)"
        }
        frame True {
          w482 = "C"
          w484 = "L"
          # "yes, we are measuring capacitance and loss  (addr. 28)"
          n245 = GPIB Clear(3:"28") -> ()  [unwired: 1 in, 2 out]
          n246 = Concatenate Strings(w479, w482, "\t") -> (w478:string)
          n247 = Build Array (concatenate)(w481, w482) -> (w480:string[])
          n248 = Concatenate Strings(w478, w484, "\t") -> (w486:string)
          n249 = Build Array (concatenate)(w480, w484) -> (w487:string[])
        }
      }
      n250 = property on="String" class="Str"("Value"=w474) -> ()  [unwired: 2 in, 2 out]
      n251 = property on="Array" class="Arr (strict)"("Value"=w472) -> ()  [unwired: 2 in, 2 out]
    }
  }
  n252 = property on="Array" class="Arr (strict)"(error in=w19) -> (error out=w1:errorcluster, "Value"=w8:string[])  [unwired: 1 in, 1 out]
  n253 = property on="String" class="Str"(error in=w1) -> ("Value"=w4:string)  [unwired: 1 in, 2 out]
  n254 = property on="Commutator" class="Bool (strict)"() -> ("Value"=w7:bool)  [unwired: 2 in, 2 out]
  n255 = case shown="True" w7 {
    tunnel: w8 -> [w491 w509]
    tunnel: [w489 w509] -> w5
    tunnel: w4 -> [w493 w508]
    tunnel: [w492 w508] -> w3
    frame True {
      n256 = Array Size(array=w491) -> (size(s)=w495:i32)
      n257 = Decrement(x=w495) -> (x-1=w494:i32)
      n258 = for {
        N: w494 -> [_]
        shift-right: [w506] -> w490
        shift-left: string[] [] -> [w507]
        shift-right: [w498] -> w492
        shift-left: w493 -> [w499]
        i -> [w503]
        n259 = property on="Array" class="Arr (strict)"() -> ("Value"=w501:string[])  [unwired: 2 in, 2 out]
        n260 = Increment(x=w503) -> (x+1=w502:i32)
        n261 = Index Array(array=w501, index=w502) -> (element=w505:string)
        n262 = Concatenate Strings("c", w505) -> (w497:string)
        n263 = Concatenate Strings(w499, w497, "\t") -> (w498:string)
        n264 = Build Array (concatenate)(w507, w497) -> (w506:string[])
      }
      n265 = Build Array (concatenate)(w491, w490) -> (w489:string[])
      n266 = property on="Array" class="Arr (strict)"("Value"=w489) -> ()  [unwired: 2 in, 2 out]
    }
    frame False {
    }
  }
  n267 = Concatenate Strings(w3, "\r", "\n") -> (w15:string)
  "String" <- w15
  n268 = property on="Ring" class="Ring (strict)"("Strings []"=w5) -> (error out=w2:errorcluster)  [unwired: 2 in, 1 out]
  n269 = property on="Data file:" class="Path"(error in=w2) -> (error out=w14:errorcluster, "Value"=w16:path)  [unwired: 1 in, 1 out]
  n270 = while {
    tunnel: w14 -> [w523]
    shift-right: [w520] -> w13
    shift-left: dbl[][] [] -> [w522]
    shift-right: [w512] -> _
    shift-left: w9 -> [w519]
    tunnel: "points at each Vg" -> [w514]
    tunnel: [w510] -> w11
    stop <- w521 stop-if-true
    w510 = 1e-08
    # "send new Vg value to main Keithley 2400"
    n271 = for {
      N: w514 -> [_]
      tunnel: w523 -> [w539]
      tunnel: [w557] -> w521
      shift-right: [w544] -> w520
      shift-left: w522 -> [w570]
      tunnel: w519 -> [w555]
      tunnel: [w562] -> w512
      w556 = dbl[] []  # Empty array for data
      # "this part appends last\nmeasured point to the \ndata file"
      # "this line is current gate voltage"
      # "First we create an empty array \nfor data and write the first element \ninto it - current gate voltage"
      # "time is measured at the beginning\nand at the end of the cycle to\ncalculate delay time required to\nkeep set sweep rate"
      # "this part calculate resistances and current (if needed) from voltages measured by lock-in amplifiers"
      # "check if the next step doesn't\ngo beyond the target voltage"
      # "calculate difference between target and current Vg"
      # "check if we are at the target voltage yet"
      # "in this part we calculate incriment for Vg"
      n272 = flat-sequence {
        tunnel: w539 -> [w1744]
        tunnel: [w1744] -> w537
        tunnel: [w1746] -> w538
        tunnel: w537 -> [w1746]
        tunnel: [w1745] -> w536
        frame #0 {
          n273 = property on="Deliberate Time delay" class="DigNum (strict)"() -> ("Value"=w1743:i32)  [unwired: 2 in, 2 out]
          n274 = Wait (ms)(milliseconds to wait=w1743) -> ()  [unwired: 1 out]
        }
        frame #1 {
          n275 = Tick Count (ms)() -> (millisecond timer value=w1745:u32)
        }
      }
      n276 = Build Array (concatenate)(w556, w555) -> (w554:dbl[])
      n277 = property on="array for data" class="Arr (strict)"(error in=w538, "Value"=w554) -> (error out=w553:errorcluster)  [unwired: 1 in, 1 out]
      n278 = case shown="False" "Commutator" {
        tunnel: [w597 w1377] -> w571
        tunnel: w553 -> [w598 w1376]
        frame True {
          n279 = stacked-sequence {
            tunnel: w598 -> [w615 w1004]
            tunnel: [_ w989] -> w597
            frame #0 {
              n280 = stacked-sequence {
                tunnel: w615 -> [w619 _ _ _ _ _ _ _ _ _ _ _ _ _ _ _ _ _ _ _ _ _ _ _ _ _]
                tunnel: [w619 _ _ _ _ _ _ _ _ _ _ _ _ _ _ _ _ _ _ _ _ _ _ _ _ _] -> w599
                frame #0 {
                  # "check if oscillator on \nlock-in (address 1)\nis to be measured"
                  n281 = property on="Current is:" class="RadioBtnsControl (strict)"() -> ("Value"=w622:T1)  [unwired: 2 in, 2 out]
                  n282 = property on="array for data" class="Arr (strict)"() -> ("Value"=w621:dbl[])  [unwired: 2 in, 2 out]
                  n283 = Equal?(x=w622, y=1) -> (x = y?=w623:bool)
                  n284 = case shown="False" w623 {
                    tunnel: w621 -> [w625 w633]
                    tunnel: [w625 w632] -> w620
                    frame False {
                      # "we are not measuring oscillator from\nlock-in (address 1)"
                    }
                    frame True {
                      w629 = "1"
                      # "we are  measuring oscillator"
                      n285 = GPIB Write(0:w629, 1:"SLVL?") -> (6:w630:errorcluster)  [unwired: 3 in, 1 out]
                      n286 = GPIB Read(0:w629, 1:3200, 3:w630) -> (5:w627:string)  [unwired: 2 in, 2 out]
                      n287 = Fract/Exp String To Number(string=w627) -> (number=w626:dbl)  [unwired: 3 in, 1 out]
                      n288 = Build Array (concatenate)(w633, w626) -> (w632:dbl[])
                    }
                  }
                  n289 = property on="array for data" class="Arr (strict)"("Value"=w620) -> ()  [unwired: 2 in, 2 out]
                }
                frame #1 {
                  # "check if in-phase\nsignal on lock-in \n(address 1) is to\nbe measured"
                  n290 = property on="array for data" class="Arr (strict)"() -> ("Value"=w636:dbl[])  [unwired: 2 in, 2 out]
                  n291 = property on="Addr 1 lock-in" class="Bool (strict)"() -> ("Value"=w634:bool)  [unwired: 2 in, 2 out]
                  n292 = case shown="False" w634 {
                    tunnel: w636 -> [w637 w645]
                    tunnel: [w637 w644] -> w635
                    frame False {
                      # "we are not measuring in phase signal on lock-in (address 1)"
                    }
                    frame True {
                      w642 = "1"
                      # "we are  measuring lock-in (address 1), in phase"
                      n293 = GPIB Write(0:w642, 1:"OUTP?1") -> (6:w643:errorcluster)  [unwired: 3 in, 1 out]
                      n294 = GPIB Read(0:w642, 1:3200, 3:w643) -> (5:w640:string)  [unwired: 2 in, 2 out]
                      n295 = Fract/Exp String To Number(string=w640) -> (number=w639:dbl)  [unwired: 3 in, 1 out]
                      n296 = Build Array (concatenate)(w645, w639) -> (w644:dbl[])
                    }
                  }
                  n297 = property on="array for data" class="Arr (strict)"("Value"=w635) -> ()  [unwired: 2 in, 2 out]
                }
                frame #2 {
                  # "check if out-of-phase\nsignal on lock-in \n(address 1) is to\nbe measured"
                  n298 = property on="Addr 1 lock-in oop" class="Bool (strict)"() -> ("Value"=w646:bool)  [unwired: 2 in, 2 out]
                  n299 = property on="array for data" class="Arr (strict)"() -> ("Value"=w648:dbl[])  [unwired: 2 in, 2 out]
                  n300 = case shown="False" w646 {
                    tunnel: w648 -> [w649 w657]
                    tunnel: [w649 w656] -> w647
                    frame False {
                      # "we are not measuring out-of-phase signal on lock-in (address 1)"
                    }
                    frame True {
                      w654 = "1"
                      # "we are  measuring lock-in (address 1), out-of-phase signal"
                      n301 = GPIB Write(0:w654, 1:"OUTP?2") -> (6:w655:errorcluster)  [unwired: 3 in, 1 out]
                      n302 = GPIB Read(0:w654, 1:3200, 3:w655) -> (5:w652:string)  [unwired: 2 in, 2 out]
                      n303 = Fract/Exp String To Number(string=w652) -> (number=w651:dbl)  [unwired: 3 in, 1 out]
                      n304 = Build Array (concatenate)(w657, w651) -> (w656:dbl[])
                    }
                  }
                  n305 = property on="array for data" class="Arr (strict)"("Value"=w647) -> ()  [unwired: 2 in, 2 out]
                }
                frame #3 {
                  # "check if in-phase\nsignal on lock-in \n(address 2) is to\nbe measured"
                  n306 = property on="Addr 2 lock-in" class="Bool (strict)"() -> ("Value"=w658:bool)  [unwired: 2 in, 2 out]
                  n307 = property on="array for data" class="Arr (strict)"() -> ("Value"=w660:dbl[])  [unwired: 2 in, 2 out]
                  n308 = case shown="False" w658 {
                    tunnel: w660 -> [w661 w669]
                    tunnel: [w661 w668] -> w659
                    frame False {
                      # "we are not measuring in phase signal on lock-in (address 2)"
                    }
                    frame True {
                      w666 = "2"
                      # "we are  measuring lock-in (address 2), in phase"
                      n309 = GPIB Write(0:w666, 1:"OUTP?1") -> (6:w667:errorcluster)  [unwired: 3 in, 1 out]
                      n310 = GPIB Read(0:w666, 1:3200, 3:w667) -> (5:w664:string)  [unwired: 2 in, 2 out]
                      n311 = Fract/Exp String To Number(string=w664) -> (number=w663:dbl)  [unwired: 3 in, 1 out]
                      n312 = Build Array (concatenate)(w669, w663) -> (w668:dbl[])
                    }
                  }
                  n313 = property on="array for data" class="Arr (strict)"("Value"=w659) -> ()  [unwired: 2 in, 2 out]
                }
                frame #4 {
                  # "check if out-of-phase\nsignal on lock-in \n(address 2) is to\nbe measured"
                  n314 = property on="Addr 2 lock-in oop" class="Bool (strict)"() -> ("Value"=w670:bool)  [unwired: 2 in, 2 out]
                  n315 = property on="array for data" class="Arr (strict)"() -> ("Value"=w672:dbl[])  [unwired: 2 in, 2 out]
                  n316 = case shown="False" w670 {
                    tunnel: w672 -> [w673 w681]
                    tunnel: [w673 w680] -> w671
                    tunnel: w670 -> [_ _]
                    frame False {
                      # "we are not measuring out-of-phase signal on lock-in (address 2)"
                    }
                    frame True {
                      w678 = "2"
                      # "we are  measuring lock-in (address 2), out-of-phase"
                      n317 = GPIB Write(0:w678, 1:"OUTP?2") -> (6:w679:errorcluster)  [unwired: 3 in, 1 out]
                      n318 = GPIB Read(0:w678, 1:3200, 3:w679) -> (5:w676:string)  [unwired: 2 in, 2 out]
                      n319 = Fract/Exp String To Number(string=w676) -> (number=w675:dbl)  [unwired: 3 in, 1 out]
                      n320 = Build Array (concatenate)(w681, w675) -> (w680:dbl[])
                    }
                  }
                  n321 = property on="array for data" class="Arr (strict)"("Value"=w671) -> ()  [unwired: 2 in, 2 out]
                }
                frame #5 {
                  # "check if in-phase\nsignal on lock-in \n(address 3) is to\nbe measured"
                  n322 = property on="Addr 3 lock-in" class="Bool (strict)"() -> ("Value"=w682:bool)  [unwired: 2 in, 2 out]
                  n323 = property on="array for data" class="Arr (strict)"() -> ("Value"=w684:dbl[])  [unwired: 2 in, 2 out]
                  n324 = case shown="False" w682 {
                    tunnel: w684 -> [w685 w693]
                    tunnel: [w685 w692] -> w683
                    frame False {
                      # "we are not measuring in phase signal on lock-in (address 3)"
                    }
                    frame True {
                      w690 = "3"
                      # "we are  measuring lock-in (address 3), in phase"
                      n325 = GPIB Write(0:w690, 1:"OUTP?1") -> (6:w691:errorcluster)  [unwired: 3 in, 1 out]
                      n326 = GPIB Read(0:w690, 1:3200, 3:w691) -> (5:w688:string)  [unwired: 2 in, 2 out]
                      n327 = Fract/Exp String To Number(string=w688) -> (number=w687:dbl)  [unwired: 3 in, 1 out]
                      n328 = Build Array (concatenate)(w693, w687) -> (w692:dbl[])
                    }
                  }
                  n329 = property on="array for data" class="Arr (strict)"("Value"=w683) -> ()  [unwired: 2 in, 2 out]
                }
                frame #6 {
                  # "check if out-of-phase\nsignal on lock-in \n(address 3) is to\nbe measured"
                  n330 = property on="Addr 3 lock-in oop" class="Bool (strict)"() -> ("Value"=w694:bool)  [unwired: 2 in, 2 out]
                  n331 = property on="array for data" class="Arr (strict)"() -> ("Value"=w696:dbl[])  [unwired: 2 in, 2 out]
                  n332 = case shown="False" w694 {
                    tunnel: w696 -> [w697 w705]
                    tunnel: [w697 w704] -> w695
                    frame False {
                      # "we are not measuring out-of-phase signal on lock-in (address 3)"
                    }
                    frame True {
                      w702 = "3"
                      # "we are  measuring lock-in (address 3), out-of-phase"
                      n333 = GPIB Write(0:w702, 1:"OUTP?2") -> (6:w703:errorcluster)  [unwired: 3 in, 1 out]
                      n334 = GPIB Read(0:w702, 1:3200, 3:w703) -> (5:w700:string)  [unwired: 2 in, 2 out]
                      n335 = Fract/Exp String To Number(string=w700) -> (number=w699:dbl)  [unwired: 3 in, 1 out]
                      n336 = Build Array (concatenate)(w705, w699) -> (w704:dbl[])
                    }
                  }
                  n337 = property on="array for data" class="Arr (strict)"("Value"=w695) -> ()  [unwired: 2 in, 2 out]
                }
                frame #7 {
                  # "check if in-phase\nsignal on lock-in \n(address 4) is to\nbe measured"
                  n338 = property on="Addr 4 lock-in" class="Bool (strict)"() -> ("Value"=w706:bool)  [unwired: 2 in, 2 out]
                  n339 = property on="array for data" class="Arr (strict)"() -> ("Value"=w708:dbl[])  [unwired: 2 in, 2 out]
                  n340 = case shown="False" w706 {
                    tunnel: w708 -> [w709 w717]
                    tunnel: [w709 w716] -> w707
                    frame False {
                      # "we are not measuring in phase signal on lock-in (address 4)"
                    }
                    frame True {
                      w714 = "4"
                      # "we are  measuring lock-in (address 4), in phase"
                      n341 = GPIB Write(0:w714, 1:"OUTP?1") -> (6:w715:errorcluster)  [unwired: 3 in, 1 out]
                      n342 = GPIB Read(0:w714, 1:3200, 3:w715) -> (5:w712:string)  [unwired: 2 in, 2 out]
                      n343 = Fract/Exp String To Number(string=w712) -> (number=w711:dbl)  [unwired: 3 in, 1 out]
                      n344 = Build Array (concatenate)(w717, w711) -> (w716:dbl[])
                    }
                  }
                  n345 = property on="array for data" class="Arr (strict)"("Value"=w707) -> ()  [unwired: 2 in, 2 out]
                }
                frame #8 {
                  # "check if out-of-phase\nsignal on lock-in \n(address 4) is to\nbe measured"
                  n346 = property on="Addr 4 lock-in oop" class="Bool (strict)"() -> ("Value"=w718:bool)  [unwired: 2 in, 2 out]
                  n347 = property on="array for data" class="Arr (strict)"() -> ("Value"=w720:dbl[])  [unwired: 2 in, 2 out]
                  n348 = case shown="False" w718 {
                    tunnel: w720 -> [w721 w729]
                    tunnel: [w721 w728] -> w719
                    frame False {
                      # "we are not measuring out-of-phase signal on lock-in (address 4)"
                    }
                    frame True {
                      w726 = "4"
                      # "we are  measuring lock-in (address 4), out-of-phase"
                      n349 = GPIB Write(0:w726, 1:"OUTP?2") -> (6:w727:errorcluster)  [unwired: 3 in, 1 out]
                      n350 = GPIB Read(0:w726, 1:3200, 3:w727) -> (5:w724:string)  [unwired: 2 in, 2 out]
                      n351 = Fract/Exp String To Number(string=w724) -> (number=w723:dbl)  [unwired: 3 in, 1 out]
                      n352 = Build Array (concatenate)(w729, w723) -> (w728:dbl[])
                    }
                  }
                  n353 = property on="array for data" class="Arr (strict)"("Value"=w719) -> ()  [unwired: 2 in, 2 out]
                }
                frame #9 {
                  # "check if in-phase\nsignal on lock-in \n(address 5) is to\nbe measured"
                  n354 = property on="Addr 5 lock-in" class="Bool (strict)"() -> ("Value"=w730:bool)  [unwired: 2 in, 2 out]
                  n355 = property on="array for data" class="Arr (strict)"() -> ("Value"=w732:dbl[])  [unwired: 2 in, 2 out]
                  n356 = case shown="False" w730 {
                    tunnel: w732 -> [w733 w741]
                    tunnel: [w733 w740] -> w731
                    frame False {
                      # "we are not measuring in phase signal on lock-in (address 5)"
                    }
                    frame True {
                      w738 = "5"
                      # "we are  measuring lock-in (address 5), in phase"
                      n357 = GPIB Write(0:w738, 1:"OUTP?1") -> (6:w739:errorcluster)  [unwired: 3 in, 1 out]
                      n358 = GPIB Read(0:w738, 1:3200, 3:w739) -> (5:w736:string)  [unwired: 2 in, 2 out]
                      n359 = Fract/Exp String To Number(string=w736) -> (number=w735:dbl)  [unwired: 3 in, 1 out]
                      n360 = Build Array (concatenate)(w741, w735) -> (w740:dbl[])
                    }
                  }
                  n361 = property on="array for data" class="Arr (strict)"("Value"=w731) -> ()  [unwired: 2 in, 2 out]
                }
                frame #10 {
                  # "check if out-of-phase\nsignal on lock-in \n(address 5) is to\nbe measured"
                  n362 = property on="Addr 5 lock-in oop" class="Bool (strict)"() -> ("Value"=w742:bool)  [unwired: 2 in, 2 out]
                  n363 = property on="array for data" class="Arr (strict)"() -> ("Value"=w744:dbl[])  [unwired: 2 in, 2 out]
                  n364 = case shown="False" w742 {
                    tunnel: w744 -> [w745 w753]
                    tunnel: [w745 w752] -> w743
                    frame False {
                      # "we are not measuring out-of-phase signal on lock-in (address 5)"
                    }
                    frame True {
                      w750 = "5"
                      # "we are  measuring lock-in (address 5), out-of-phase"
                      n365 = GPIB Write(0:w750, 1:"OUTP?2") -> (6:w751:errorcluster)  [unwired: 3 in, 1 out]
                      n366 = GPIB Read(0:w750, 1:3200, 3:w751) -> (5:w748:string)  [unwired: 2 in, 2 out]
                      n367 = Fract/Exp String To Number(string=w748) -> (number=w747:dbl)  [unwired: 3 in, 1 out]
                      n368 = Build Array (concatenate)(w753, w747) -> (w752:dbl[])
                    }
                  }
                  n369 = property on="array for data" class="Arr (strict)"("Value"=w743) -> ()  [unwired: 2 in, 2 out]
                }
                frame #11 {
                  # "check if voltage on \nmain Keithley 2400 \n(addr. 12) is to\nbe measured"
                  n370 = property on="Voltage (Vk1)" class="Bool (strict)"() -> ("Value"=w754:bool)  [unwired: 2 in, 2 out]
                  n371 = property on="array for data" class="Arr (strict)"() -> ("Value"=w756:dbl[])  [unwired: 2 in, 2 out]
                  n372 = case shown="False" w754 {
                    tunnel: w756 -> [w757 w767]
                    tunnel: [w757 w766] -> w755
                    frame False {
                      # "we aren't measuring voltage \non main Keithley 2400 (addr. 12)"
                    }
                    frame True {
                      w764 = "12"
                      # "we are measuring voltage \non main Keithley 2400 (addr. 12)"
                      n373 = GPIB Write(0:w764, 1:":READ?") -> (6:w765:errorcluster)  [unwired: 3 in, 1 out]
                      n374 = GPIB Read(0:w764, 1:3200, 3:w765) -> (5:w760:string)  [unwired: 2 in, 2 out]
                      n375 = String Subset(string=w760, length (rest)=13) -> (substring=w759:string)  [unwired: 1 in]
                      n376 = Fract/Exp String To Number(string=w759) -> (number=w762:dbl)  [unwired: 3 in, 1 out]
                      n377 = Build Array (concatenate)(w767, w762) -> (w766:dbl[])
                    }
                  }
                  n378 = property on="array for data" class="Arr (strict)"("Value"=w755) -> ()  [unwired: 2 in, 2 out]
                }
                frame #12 {
                  # "check if  current on \nmain Keithley 2400 \n(addr. 12) is to\nbe measured"
                  n379 = property on="Current (Ik1)" class="Bool (strict)"() -> ("Value"=w768:bool)  [unwired: 2 in, 2 out]
                  n380 = property on="array for data" class="Arr (strict)"() -> ("Value"=w770:dbl[])  [unwired: 2 in, 2 out]
                  n381 = case shown="True" w768 {
                    tunnel: w770 -> [w771 w782]
                    tunnel: [w771 w781] -> w769
                    frame False {
                      # "we aren't measuring current \non main Keithley 2400 (addr. 12)"
                    }
                    frame True {
                      w779 = "12"
                      # "we are measuring current\non main Keithley 2400 (addr. 12)"
                      n382 = GPIB Write(0:w779, 1:":READ?") -> (6:w780:errorcluster)  [unwired: 3 in, 1 out]
                      n383 = GPIB Read(0:w779, 1:3200, 3:w780) -> (5:w775:string)  [unwired: 2 in, 2 out]
                      n384 = String Subset(string=w775, offset (0)=14, length (rest)=13) -> (substring=w774:string)
                      n385 = Fract/Exp String To Number(string=w774) -> (number=w777:dbl)  [unwired: 3 in, 1 out]
                      n386 = Build Array (concatenate)(w782, w777) -> (w781:dbl[])
                    }
                  }
                  n387 = property on="array for data" class="Arr (strict)"("Value"=w769) -> ()  [unwired: 2 in, 2 out]
                }
                frame #13 {
                  # "check if voltage on \nadd. Keithley 2400 \n(addr. 13) is to\nbe measured"
                  n388 = property on="Voltage (Vk2)" class="Bool (strict)"() -> ("Value"=w783:bool)  [unwired: 2 in, 2 out]
                  n389 = property on="array for data" class="Arr (strict)"() -> ("Value"=w785:dbl[])  [unwired: 2 in, 2 out]
                  n390 = case shown="True" w783 {
                    tunnel: w785 -> [w786 w796]
                    tunnel: [w786 w795] -> w784
                    frame False {
                      # "we aren't measuring voltage \non additional Keithley 2400 (addr. 13)"
                    }
                    frame True {
                      w793 = "13"
                      # "we are measuring voltage \non additional Keithley 2400 (addr. 13)"
                      n391 = GPIB Write(0:w793, 1:":READ?") -> (6:w794:errorcluster)  [unwired: 3 in, 1 out]
                      n392 = GPIB Read(0:w793, 1:3200, 3:w794) -> (5:w789:string)  [unwired: 2 in, 2 out]
                      n393 = String Subset(string=w789, length (rest)=13) -> (substring=w788:string)  [unwired: 1 in]
                      n394 = Fract/Exp String To Number(string=w788) -> (number=w791:dbl)  [unwired: 3 in, 1 out]
                      n395 = Build Array (concatenate)(w796, w791) -> (w795:dbl[])
                    }
                  }
                  n396 = property on="array for data" class="Arr (strict)"("Value"=w784) -> ()  [unwired: 2 in, 2 out]
                }
                frame #14 {
                  # "check if  current on \nadd. Keithley 2400 \n(addr. 13) is to\nbe measured"
                  n397 = property on="Current (Ik2)" class="Bool (strict)"() -> ("Value"=w797:bool)  [unwired: 2 in, 2 out]
                  n398 = property on="array for data" class="Arr (strict)"() -> ("Value"=w799:dbl[])  [unwired: 2 in, 2 out]
                  n399 = case shown="True" w797 {
                    tunnel: w799 -> [w800 w811]
                    tunnel: [w800 w810] -> w798
                    frame False {
                      # "we aren't measuring current \non additional Keithley 2400 (addr. 13)"
                    }
                    frame True {
                      w808 = "13"
                      # "we are measuring current\non additional Keithley 2400 (addr. 13)"
                      n400 = GPIB Write(0:w808, 1:":READ?") -> (6:w809:errorcluster)  [unwired: 3 in, 1 out]
                      n401 = GPIB Read(0:w808, 1:3200, 3:w809) -> (5:w804:string)  [unwired: 2 in, 2 out]
                      n402 = String Subset(string=w804, offset (0)=14, length (rest)=13) -> (substring=w803:string)
                      n403 = Fract/Exp String To Number(string=w803) -> (number=w806:dbl)  [unwired: 3 in, 1 out]
                      n404 = Build Array (concatenate)(w811, w806) -> (w810:dbl[])
                    }
                  }
                  n405 = property on="array for data" class="Arr (strict)"("Value"=w798) -> ()  [unwired: 2 in, 2 out]
                }
                frame #15 {
                  # "check if voltage on \nadd. Keithley 2400 \n(addr. 14) is to\nbe measured"
                  n406 = property on="Voltage (Vk3)" class="Bool (strict)"() -> ("Value"=w812:bool)  [unwired: 2 in, 2 out]
                  n407 = property on="array for data" class="Arr (strict)"() -> ("Value"=w814:dbl[])  [unwired: 2 in, 2 out]
                  n408 = case shown="True" w812 {
                    tunnel: w814 -> [w815 w825]
                    tunnel: [w815 w824] -> w813
                    frame False {
                      # "we aren't measuring voltage \non additional Keithley 2400 (addr. 14)"
                    }
                    frame True {
                      w822 = "14"
                      # "we are measuring voltage \non additional Keithley 2400 (addr. 14)"
                      n409 = GPIB Write(0:w822, 1:":READ?") -> (6:w823:errorcluster)  [unwired: 3 in, 1 out]
                      n410 = GPIB Read(0:w822, 1:3200, 3:w823) -> (5:w818:string)  [unwired: 2 in, 2 out]
                      n411 = String Subset(string=w818, length (rest)=13) -> (substring=w817:string)  [unwired: 1 in]
                      n412 = Fract/Exp String To Number(string=w817) -> (number=w820:dbl)  [unwired: 3 in, 1 out]
                      n413 = Build Array (concatenate)(w825, w820) -> (w824:dbl[])
                    }
                  }
                  n414 = property on="array for data" class="Arr (strict)"("Value"=w813) -> ()  [unwired: 2 in, 2 out]
                }
                frame #16 {
                  # "check if  current on \nadd. Keithley 2400 \n(addr. 14) is to\nbe measured"
                  n415 = property on="Current (Ik3)" class="Bool (strict)"() -> ("Value"=w826:bool)  [unwired: 2 in, 2 out]
                  n416 = property on="array for data" class="Arr (strict)"() -> ("Value"=w828:dbl[])  [unwired: 2 in, 2 out]
                  n417 = case shown="True" w826 {
                    tunnel: w828 -> [w829 w840]
                    tunnel: [w829 w839] -> w827
                    frame False {
                      # "we aren't measuring current \non additional Keithley 2400 (addr. 14)"
                    }
                    frame True {
                      w837 = "14"
                      # "we are measuring current\non additional Keithley 2400 (addr. 14)"
                      n418 = GPIB Write(0:w837, 1:":READ?") -> (6:w838:errorcluster)  [unwired: 3 in, 1 out]
                      n419 = GPIB Read(0:w837, 1:3200, 3:w838) -> (5:w833:string)  [unwired: 2 in, 2 out]
                      n420 = String Subset(string=w833, offset (0)=14, length (rest)=13) -> (substring=w832:string)
                      n421 = Fract/Exp String To Number(string=w832) -> (number=w835:dbl)  [unwired: 3 in, 1 out]
                      n422 = Build Array (concatenate)(w840, w835) -> (w839:dbl[])
                    }
                  }
                  n423 = property on="array for data" class="Arr (strict)"("Value"=w827) -> ()  [unwired: 2 in, 2 out]
                }
                frame #17 {
                  # "check if 1st channel\non Keithley 2182 \n(addr. 15) is to\nbe measured"
                  n424 = property on="Channel 1 (Vnano1)" class="Bool (strict)"() -> ("Value"=w841:bool)  [unwired: 2 in, 2 out]
                  n425 = property on="array for data" class="Arr (strict)"() -> ("Value"=w843:dbl[])  [unwired: 2 in, 2 out]
                  n426 = case shown="True" w841 {
                    tunnel: w843 -> [w844 w852]
                    tunnel: [w844 w851] -> w842
                    frame False {
                      # "we are not measuring 1st channel\non Keithley 2182 (addr. 15)"
                    }
                    frame True {
                      w849 = "15"
                      # "we are measuring 1st channel\non Keithley 2182 (addr. 15)"
                      n427 = GPIB Write(0:w849, 1:":SENSe:DATA:FRES?") -> (6:w850:errorcluster)  [unwired: 3 in, 1 out]
                      n428 = GPIB Read(0:w849, 1:200, 3:w850) -> (5:w845:string)  [unwired: 2 in, 2 out]
                      n429 = Fract/Exp String To Number(string=w845) -> (number=w847:dbl)  [unwired: 3 in, 1 out]
                      n430 = Build Array (concatenate)(w852, w847) -> (w851:dbl[])
                    }
                  }
                  n431 = property on="array for data" class="Arr (strict)"("Value"=w842) -> ()  [unwired: 2 in, 2 out]
                }
                frame #18 {
                  # "check if 2nd channel\non Keithley 2182 \n(addr. 15) is to\nbe measured"
                  n432 = property on="Channel 2 (Vnano1b)" class="Bool (strict)"() -> ("Value"=w853:bool)  [unwired: 2 in, 2 out]
                  n433 = property on="array for data" class="Arr (strict)"() -> ("Value"=w855:dbl[])  [unwired: 2 in, 2 out]
                  n434 = case shown="False" w853 {
                    tunnel: w855 -> [w856 w868]
                    tunnel: [w856 w867] -> w854
                    frame False {
                      # "we are not measuring 1st channel\non Keithley 2182 (addr. 15)"
                    }
                    frame True {
                      w859 = "15"
                      # "switching to channel 2 and then\nback to channel 1"
                      # "we are measuring 2nd channel\non Keithley 2182 (addr. 15)"
                      n435 = GPIB Write(0:w859, 1:":SENSe:CHAN 2") -> (6:w860:errorcluster)  [unwired: 3 in, 1 out]
                      n436 = GPIB Write(0:w859, 1:":SENSe:DATA:FRES?", 3:w860) -> (6:w866:errorcluster)  [unwired: 2 in, 1 out]
                      n437 = GPIB Read(0:w859, 1:200, 3:w866) -> (5:w862:string, 7:w858:errorcluster)  [unwired: 2 in, 1 out]
                      n438 = GPIB Write(0:w859, 1:":SENSe:CHAN 1", 3:w858) -> ()  [unwired: 2 in, 2 out]
                      n439 = Fract/Exp String To Number(string=w862) -> (number=w864:dbl)  [unwired: 3 in, 1 out]
                      n440 = Build Array (concatenate)(w868, w864) -> (w867:dbl[])
                    }
                  }
                  n441 = property on="array for data" class="Arr (strict)"("Value"=w854) -> ()  [unwired: 2 in, 2 out]
                }
                frame #19 {
                  # "check if 1st channel\non Keithley 2182 \n(addr. 16) is to\nbe measured"
                  n442 = property on="Channel 1 (Vnano2)" class="Bool (strict)"() -> ("Value"=w869:bool)  [unwired: 2 in, 2 out]
                  n443 = property on="array for data" class="Arr (strict)"() -> ("Value"=w871:dbl[])  [unwired: 2 in, 2 out]
                  n444 = case shown="True" w869 {
                    tunnel: w871 -> [w872 w880]
                    tunnel: [w872 w879] -> w870
                    frame False {
                      # "we are not measuring 1st channel\non Keithley 2182 (addr. 16)"
                    }
                    frame True {
                      w877 = "16"
                      # "we are measuring 1st channel\non Keithley 2182 (addr. 16)"
                      n445 = GPIB Write(0:w877, 1:":SENSe:DATA:FRES?") -> (6:w878:errorcluster)  [unwired: 3 in, 1 out]
                      n446 = GPIB Read(0:w877, 1:200, 3:w878) -> (5:w873:string)  [unwired: 2 in, 2 out]
                      n447 = Fract/Exp String To Number(string=w873) -> (number=w875:dbl)  [unwired: 3 in, 1 out]
                      n448 = Build Array (concatenate)(w880, w875) -> (w879:dbl[])
                    }
                  }
                  n449 = property on="array for data" class="Arr (strict)"("Value"=w870) -> ()  [unwired: 2 in, 2 out]
                }
                frame #20 {
                  # "check if 2nd channel\non Keithley 2182 \n(addr. 16) is to\nbe measured"
                  n450 = property on="Channel 2 (Vnano2b)" class="Bool (strict)"() -> ("Value"=w881:bool)  [unwired: 2 in, 2 out]
                  n451 = property on="array for data" class="Arr (strict)"() -> ("Value"=w883:dbl[])  [unwired: 2 in, 2 out]
                  n452 = case shown="False" w881 {
                    tunnel: w883 -> [w884 w896]
                    tunnel: [w884 w895] -> w882
                    frame False {
                      # "we are not measuring 1st channel\non Keithley 2182 (addr. 16)"
                    }
                    frame True {
                      w887 = "16"
                      # "switching to channel 2 and then\nback to channel 1"
                      # "we are measuring 2nd channel\non Keithley 2182 (addr. 16)"
                      n453 = GPIB Write(0:w887, 1:":SENSe:CHAN 2") -> (6:w888:errorcluster)  [unwired: 3 in, 1 out]
                      n454 = GPIB Write(0:w887, 1:":SENSe:DATA:FRES?", 3:w888) -> (6:w894:errorcluster)  [unwired: 2 in, 1 out]
                      n455 = GPIB Read(0:w887, 1:200, 3:w894) -> (5:w890:string, 7:w886:errorcluster)  [unwired: 2 in, 1 out]
                      n456 = GPIB Write(0:w887, 1:":SENSe:CHAN 1", 3:w886) -> ()  [unwired: 2 in, 2 out]
                      n457 = Fract/Exp String To Number(string=w890) -> (number=w892:dbl)  [unwired: 3 in, 1 out]
                      n458 = Build Array (concatenate)(w896, w892) -> (w895:dbl[])
                    }
                  }
                  n459 = property on="array for data" class="Arr (strict)"("Value"=w882) -> ()  [unwired: 2 in, 2 out]
                }
                frame #21 {
                  # "check if 1st channel\non Keithley 2182 \n(addr. 17) is to\nbe measured"
                  n460 = property on="Channel 1 (Vnano3)" class="Bool (strict)"() -> ("Value"=w897:bool)  [unwired: 2 in, 2 out]
                  n461 = property on="array for data" class="Arr (strict)"() -> ("Value"=w899:dbl[])  [unwired: 2 in, 2 out]
                  n462 = case shown="True" w897 {
                    tunnel: w899 -> [w900 w908]
                    tunnel: [w900 w907] -> w898
                    frame False {
                      # "we are not measuring 1st channel\non Keithley 2182 (addr. 17)"
                    }
                    frame True {
                      w905 = "17"
                      # "we are measuring 1st channel\non Keithley 2182 (addr. 17)"
                      n463 = GPIB Write(0:w905, 1:":SENSe:DATA:FRES?") -> (6:w906:errorcluster)  [unwired: 3 in, 1 out]
                      n464 = GPIB Read(0:w905, 1:200, 3:w906) -> (5:w901:string)  [unwired: 2 in, 2 out]
                      n465 = Fract/Exp String To Number(string=w901) -> (number=w903:dbl)  [unwired: 3 in, 1 out]
                      n466 = Build Array (concatenate)(w908, w903) -> (w907:dbl[])
                    }
                  }
                  n467 = property on="array for data" class="Arr (strict)"("Value"=w898) -> ()  [unwired: 2 in, 2 out]
                }
                frame #22 {
                  # "check if 2nd channel\non Keithley 2182 \n(addr. 17) is to\nbe measured"
                  n468 = property on="Channel 2 (Vnano3b)" class="Bool (strict)"() -> ("Value"=w909:bool)  [unwired: 2 in, 2 out]
                  n469 = property on="array for data" class="Arr (strict)"() -> ("Value"=w911:dbl[])  [unwired: 2 in, 2 out]
                  n470 = case shown="False" w909 {
                    tunnel: w911 -> [w912 w924]
                    tunnel: [w912 w923] -> w910
                    frame False {
                      # "we are not measuring 1st channel\non Keithley 2182 (addr. 17)"
                    }
                    frame True {
                      w915 = "17"
                      # "switching to channel 2 and then\nback to channel 1"
                      # "we are measuring 2nd channel\non Keithley 2182 (addr. 17)"
                      n471 = GPIB Write(0:w915, 1:":SENSe:CHAN 2") -> (6:w916:errorcluster)  [unwired: 3 in, 1 out]
                      n472 = GPIB Write(0:w915, 1:":SENSe:DATA:FRES?", 3:w916) -> (6:w922:errorcluster)  [unwired: 2 in, 1 out]
                      n473 = GPIB Read(0:w915, 1:200, 3:w922) -> (5:w918:string, 7:w914:errorcluster)  [unwired: 2 in, 1 out]
                      n474 = GPIB Write(0:w915, 1:":SENSe:CHAN 1", 3:w914) -> ()  [unwired: 2 in, 2 out]
                      n475 = Fract/Exp String To Number(string=w918) -> (number=w920:dbl)  [unwired: 3 in, 1 out]
                      n476 = Build Array (concatenate)(w924, w920) -> (w923:dbl[])
                    }
                  }
                  n477 = property on="array for data" class="Arr (strict)"("Value"=w910) -> ()  [unwired: 2 in, 2 out]
                }
                frame #23 {
                  # "check if 1st \nthermometer on \nOxford ITC \n(address 24) \nis measured"
                  n478 = property on="Thermometer 1 (T1)" class="Bool (strict)"() -> ("Value"=w925:bool)  [unwired: 2 in, 2 out]
                  n479 = property on="array for data" class="Arr (strict)"() -> ("Value"=w927:dbl[])  [unwired: 2 in, 2 out]
                  n480 = case shown="True" w925 {
                    tunnel: w927 -> [w928 w937]
                    tunnel: [w928 w936] -> w926
                    frame False {
                      # "we are not measuring temperature on\nthermometer 1 (addr. 24)"
                    }
                    frame True {
                      w929 = 1
                      w934 = "24"
                      # "we are measuring temperature,\nthermometer 1 (addr. 24)"
                      n481 = GPIB Write(0:w934, 1:"R 1", 2:w929) -> (6:w935:errorcluster)  [unwired: 2 in, 1 out]
                      n482 = GPIB Read(0:w934, 1:200, 2:w929, 3:w935) -> (5:w930:string)  [unwired: 1 in, 2 out]
                      n483 = Fract/Exp String To Number(string=w930, offset=w929) -> (number=w932:dbl)  [unwired: 2 in, 1 out]
                      n484 = Build Array (concatenate)(w937, w932) -> (w936:dbl[])
                    }
                  }
                  n485 = property on="array for data" class="Arr (strict)"("Value"=w926) -> ()  [unwired: 2 in, 2 out]
                }
                frame #24 {
                  # "check if 1st \nthermometer on \nOxford ITC \n(address 24) \nis measured"
                  n486 = property on="Magnetic Field (B)" class="Bool (strict)"() -> ("Value"=w938:bool)  [unwired: 2 in, 2 out]
                  n487 = property on="array for data" class="Arr (strict)"() -> ("Value"=w940:dbl[])  [unwired: 2 in, 2 out]
                  n488 = case shown="True" w938 {
                    tunnel: w940 -> [w941 w950]
                    tunnel: [w941 w949] -> w939
                    frame False {
                      # "we are not measuringmagnetic field (addr. 25)"
                    }
                    frame True {
                      w942 = 1
                      w947 = "25"
                      # "we are measuring magnetic field  (addr. 25)"
                      n489 = GPIB Write(0:w947, 1:"R 7", 2:w942) -> (6:w948:errorcluster)  [unwired: 2 in, 1 out]
                      n490 = GPIB Read(0:w947, 1:200, 2:w942, 3:w948) -> (5:w943:string)  [unwired: 1 in, 2 out]
                      n491 = Fract/Exp String To Number(string=w943, offset=w942) -> (number=w945:dbl)  [unwired: 2 in, 1 out]
                      n492 = Build Array (concatenate)(w950, w945) -> (w949:dbl[])
                    }
                  }
                  n493 = property on="array for data" class="Arr (strict)"("Value"=w939) -> ()  [unwired: 2 in, 2 out]
                }
                frame #25 {
                  # "check if capacitance\nand loss (address 28)\nare measured"
                  n494 = property on="Capacitance (C) and Loss (L)" class="Bool (strict)"() -> ("Value"=w951:bool)  [unwired: 2 in, 2 out]
                  n495 = property on="array for data" class="Arr (strict)"() -> ("Value"=w953:dbl[])  [unwired: 2 in, 2 out]
                  n496 = case shown="False" w951 {
                    tunnel: w953 -> [w954 w960]
                    tunnel: [w954 w956] -> w952
                    frame False {
                      # "we are not measuringmagnetic capacitance (addr. 28)"
                    }
                    frame True {
                      # "we are measuring capacitance and loss  (addr. 28)"
                      n497 = stacked-sequence {
                        seq-local: [w962 _ _] -> [_ _ w985]
                        tunnel: [_ _ w979] -> w955
                        tunnel: [_ _ w980] -> w958
                        tunnel: "28" ("data") -> [w961 w965 w974]
                        frame #0 {
                          n498 = GPIB Write(0:w961, 1:"SINGLE" ("data"), 2:i16 0 ("mode (0)")) -> (6:w962:errorcluster)  [unwired: 2 in, 1 out]
                        }
                        frame #1 {
                          n499 = while {
                            tunnel: w965 -> [w966]
                            i -> [w967]
                            stop <- w969 continue-if-true
                            n500 = GPIB Serial Poll(0:w966) -> (2:w971:i16)  [unwired: 1 in, 2 out]
                            n501 = Less?(x=w971, y=i16 128) -> (x < y?=w969:bool)
                            n502 = Wait (ms)(milliseconds to wait=u32 50) -> ()  [unwired: 1 out]
                            "Numeric" <- w967
                          }
                        }
                        frame #2 {
                          w972 = i16 2 ("mode (0)")
                          n503 = GPIB Read(0:w974, 1:200 ("byte count"), 2:i16 2 ("mode (0)"), 3:w985) -> (5:w978:string)  [unwired: 1 in, 2 out]
                          n504 = Match Pattern(string=w978, regular expression="C=") -> (after substring=w977:string)  [unwired: 1 in, 3 out]
                          n505 = Match Pattern(string=w977, regular expression="PF L=") -> (after substring=w975:string)  [unwired: 1 in, 3 out]
                          n506 = Search/Split String(string=w977, search string/char (-)=" ", offset (0)=w972) -> (substring before match=w982:string)  [unwired: 2 out]
                          n507 = Search/Split String(string=w975, search string/char (-)=" ", offset (0)=w972) -> (substring before match=w981:string)  [unwired: 2 out]
                          n508 = Fract/Exp String To Number(string=w981) -> (number=w979:dbl)  [unwired: 3 in, 1 out]
                          n509 = Fract/Exp String To Number(string=w982) -> (number=w980:dbl)  [unwired: 3 in, 1 out]
                        }
                      }
                      n510 = Build Array (concatenate)(w960, w958) -> (w957:dbl[])
                      n511 = Build Array (concatenate)(w957, w955) -> (w956:dbl[])
                    }
                  }
                  n512 = property on="array for data" class="Arr (strict)"("Value"=w952) -> ()  [unwired: 2 in, 2 out]
                }
              }
              n513 = flat-sequence {
                tunnel: w600 -> [_]
                frame #0 {
                  n514 = property on="Delib Time delay" class="DigNum (strict)"() -> ("Value"=w616:i32)  [unwired: 2 in, 2 out]
                  n515 = Wait (ms)(milliseconds to wait=w616) -> ()  [unwired: 1 out]
                }
              }
              n516 = case shown="\"Radio Selection 2\"" "Commute SorceMeter" {
                tunnel: ["13" "14"] -> w601
                frame "Radio Selection 1", Default {
                }
                frame "Radio Selection 2" {
                }
              }
              n517 = GPIB Write(0:w601, 1:":READ?", 3:w599) -> (6:w602:errorcluster)  [unwired: 2 in, 1 out]
              n518 = GPIB Read(0:w601, 1:3200, 3:w602) -> (5:w605:string)  [unwired: 2 in, 2 out]
              n519 = String Subset(string=w605, length (rest)=13) -> (substring=w606:string)  [unwired: 1 in]
              n520 = Fract/Exp String To Number(string=w606) -> (number=w608:dbl)  [unwired: 3 in, 1 out]
              n521 = Multiply(x=w608, y=-1.0) -> (x*y=w613:dbl)
              n522 = Number To Fractional String(number=w613) -> (F-format string=w610:string)  [unwired: 3 in]
              n523 = Concatenate Strings(":INIT:IMM; :SOUR:VOLT:LEV:IMM:AMPL " ("data"), w610) -> (w611:string)
              n524 = GPIB Write(0:w601, 1:w611) -> (6:w600:errorcluster)  [unwired: 3 in, 1 out]
            }
            frame #1 {
              n525 = stacked-sequence {
                tunnel: w1004 -> [w1007 _ _ _ _ _ _ _ _ _ _ _ _ _ _ _ _ _ _ _ _ _ _ _ _ _]
                tunnel: [w1007 _ _ _ _ _ _ _ _ _ _ _ _ _ _ _ _ _ _ _ _ _ _ _ _ _] -> w990
                frame #0 {
                  # "check if oscillator on \nlock-in (address 1)\nis to be measured"
                  n526 = property on="Current is:" class="RadioBtnsControl (strict)"() -> ("Value"=w1010:T1)  [unwired: 2 in, 2 out]
                  n527 = property on="array for data" class="Arr (strict)"() -> ("Value"=w1009:dbl[])  [unwired: 2 in, 2 out]
                  n528 = Equal?(x=w1010, y=1) -> (x = y?=w1011:bool)
                  n529 = case shown="False" w1011 {
                    tunnel: w1009 -> [w1013 w1021]
                    tunnel: [w1013 w1020] -> w1008
                    frame False {
                      # "we are not measuring oscillator from\nlock-in (address 1)"
                    }
                    frame True {
                      w1017 = "1"
                      # "we are  measuring oscillator"
                      n530 = GPIB Write(0:w1017, 1:"SLVL?") -> (6:w1018:errorcluster)  [unwired: 3 in, 1 out]
                      n531 = GPIB Read(0:w1017, 1:3200, 3:w1018) -> (5:w1015:string)  [unwired: 2 in, 2 out]
                      n532 = Fract/Exp String To Number(string=w1015) -> (number=w1014:dbl)  [unwired: 3 in, 1 out]
                      n533 = Build Array (concatenate)(w1021, w1014) -> (w1020:dbl[])
                    }
                  }
                  n534 = property on="array for data" class="Arr (strict)"("Value"=w1008) -> ()  [unwired: 2 in, 2 out]
                }
                frame #1 {
                  # "check if in-phase\nsignal on lock-in \n(address 1) is to\nbe measured"
                  n535 = property on="array for data" class="Arr (strict)"() -> ("Value"=w1024:dbl[])  [unwired: 2 in, 2 out]
                  n536 = property on="Addr 1 lock-in" class="Bool (strict)"() -> ("Value"=w1022:bool)  [unwired: 2 in, 2 out]
                  n537 = case shown="True" w1022 {
                    tunnel: w1024 -> [w1025 w1033]
                    tunnel: [w1025 w1032] -> w1023
                    frame False {
                      # "we are not measuring in phase signal on lock-in (address 1)"
                    }
                    frame True {
                      w1030 = "1"
                      # "we are  measuring lock-in (address 1), in phase"
                      n538 = GPIB Write(0:w1030, 1:"OUTP?1") -> (6:w1031:errorcluster)  [unwired: 3 in, 1 out]
                      n539 = GPIB Read(0:w1030, 1:3200, 3:w1031) -> (5:w1028:string)  [unwired: 2 in, 2 out]
                      n540 = Fract/Exp String To Number(string=w1028) -> (number=w1027:dbl)  [unwired: 3 in, 1 out]
                      n541 = Build Array (concatenate)(w1033, w1027) -> (w1032:dbl[])
                    }
                  }
                  n542 = property on="array for data" class="Arr (strict)"("Value"=w1023) -> ()  [unwired: 2 in, 2 out]
                }
                frame #2 {
                  # "check if out-of-phase\nsignal on lock-in \n(address 1) is to\nbe measured"
                  n543 = property on="Addr 1 lock-in oop" class="Bool (strict)"() -> ("Value"=w1034:bool)  [unwired: 2 in, 2 out]
                  n544 = property on="array for data" class="Arr (strict)"() -> ("Value"=w1036:dbl[])  [unwired: 2 in, 2 out]
                  n545 = case shown="True" w1034 {
                    tunnel: w1036 -> [w1037 w1045]
                    tunnel: [w1037 w1044] -> w1035
                    frame False {
                      # "we are not measuring out-of-phase signal on lock-in (address 1)"
                    }
                    frame True {
                      w1042 = "1"
                      # "we are  measuring lock-in (address 1), out-of-phase signal"
                      n546 = GPIB Write(0:w1042, 1:"OUTP?2") -> (6:w1043:errorcluster)  [unwired: 3 in, 1 out]
                      n547 = GPIB Read(0:w1042, 1:3200, 3:w1043) -> (5:w1040:string)  [unwired: 2 in, 2 out]
                      n548 = Fract/Exp String To Number(string=w1040) -> (number=w1039:dbl)  [unwired: 3 in, 1 out]
                      n549 = Build Array (concatenate)(w1045, w1039) -> (w1044:dbl[])
                    }
                  }
                  n550 = property on="array for data" class="Arr (strict)"("Value"=w1035) -> ()  [unwired: 2 in, 2 out]
                }
                frame #3 {
                  # "check if in-phase\nsignal on lock-in \n(address 2) is to\nbe measured"
                  n551 = property on="Addr 2 lock-in" class="Bool (strict)"() -> ("Value"=w1046:bool)  [unwired: 2 in, 2 out]
                  n552 = property on="array for data" class="Arr (strict)"() -> ("Value"=w1048:dbl[])  [unwired: 2 in, 2 out]
                  n553 = case shown="False" w1046 {
                    tunnel: w1048 -> [w1049 w1057]
                    tunnel: [w1049 w1056] -> w1047
                    frame False {
                      # "we are not measuring in phase signal on lock-in (address 2)"
                    }
                    frame True {
                      w1054 = "2"
                      # "we are  measuring lock-in (address 2), in phase"
                      n554 = GPIB Write(0:w1054, 1:"OUTP?1") -> (6:w1055:errorcluster)  [unwired: 3 in, 1 out]
                      n555 = GPIB Read(0:w1054, 1:3200, 3:w1055) -> (5:w1052:string)  [unwired: 2 in, 2 out]
                      n556 = Fract/Exp String To Number(string=w1052) -> (number=w1051:dbl)  [unwired: 3 in, 1 out]
                      n557 = Build Array (concatenate)(w1057, w1051) -> (w1056:dbl[])
                    }
                  }
                  n558 = property on="array for data" class="Arr (strict)"("Value"=w1047) -> ()  [unwired: 2 in, 2 out]
                }
                frame #4 {
                  # "check if out-of-phase\nsignal on lock-in \n(address 2) is to\nbe measured"
                  n559 = property on="Addr 2 lock-in oop" class="Bool (strict)"() -> ("Value"=w1058:bool)  [unwired: 2 in, 2 out]
                  n560 = property on="array for data" class="Arr (strict)"() -> ("Value"=w1060:dbl[])  [unwired: 2 in, 2 out]
                  n561 = case shown="False" w1058 {
                    tunnel: w1060 -> [w1061 w1069]
                    tunnel: [w1061 w1068] -> w1059
                    tunnel: w1058 -> [_ _]
                    frame False {
                      # "we are not measuring out-of-phase signal on lock-in (address 2)"
                    }
                    frame True {
                      w1066 = "2"
                      # "we are  measuring lock-in (address 2), out-of-phase"
                      n562 = GPIB Write(0:w1066, 1:"OUTP?2") -> (6:w1067:errorcluster)  [unwired: 3 in, 1 out]
                      n563 = GPIB Read(0:w1066, 1:3200, 3:w1067) -> (5:w1064:string)  [unwired: 2 in, 2 out]
                      n564 = Fract/Exp String To Number(string=w1064) -> (number=w1063:dbl)  [unwired: 3 in, 1 out]
                      n565 = Build Array (concatenate)(w1069, w1063) -> (w1068:dbl[])
                    }
                  }
                  n566 = property on="array for data" class="Arr (strict)"("Value"=w1059) -> ()  [unwired: 2 in, 2 out]
                }
                frame #5 {
                  # "check if in-phase\nsignal on lock-in \n(address 3) is to\nbe measured"
                  n567 = property on="Addr 3 lock-in" class="Bool (strict)"() -> ("Value"=w1070:bool)  [unwired: 2 in, 2 out]
                  n568 = property on="array for data" class="Arr (strict)"() -> ("Value"=w1072:dbl[])  [unwired: 2 in, 2 out]
                  n569 = case shown="True" w1070 {
                    tunnel: w1072 -> [w1073 w1081]
                    tunnel: [w1073 w1080] -> w1071
                    frame False {
                      # "we are not measuring in phase signal on lock-in (address 3)"
                    }
                    frame True {
                      w1078 = "3"
                      # "we are  measuring lock-in (address 3), in phase"
                      n570 = GPIB Write(0:w1078, 1:"OUTP?1") -> (6:w1079:errorcluster)  [unwired: 3 in, 1 out]
                      n571 = GPIB Read(0:w1078, 1:3200, 3:w1079) -> (5:w1076:string)  [unwired: 2 in, 2 out]
                      n572 = Fract/Exp String To Number(string=w1076) -> (number=w1075:dbl)  [unwired: 3 in, 1 out]
                      n573 = Build Array (concatenate)(w1081, w1075) -> (w1080:dbl[])
                    }
                  }
                  n574 = property on="array for data" class="Arr (strict)"("Value"=w1071) -> ()  [unwired: 2 in, 2 out]
                }
                frame #6 {
                  # "check if out-of-phase\nsignal on lock-in \n(address 3) is to\nbe measured"
                  n575 = property on="Addr 3 lock-in oop" class="Bool (strict)"() -> ("Value"=w1082:bool)  [unwired: 2 in, 2 out]
                  n576 = property on="array for data" class="Arr (strict)"() -> ("Value"=w1084:dbl[])  [unwired: 2 in, 2 out]
                  n577 = case shown="True" w1082 {
                    tunnel: w1084 -> [w1085 w1093]
                    tunnel: [w1085 w1092] -> w1083
                    frame False {
                      # "we are not measuring out-of-phase signal on lock-in (address 3)"
                    }
                    frame True {
                      w1090 = "3"
                      # "we are  measuring lock-in (address 3), out-of-phase"
                      n578 = GPIB Write(0:w1090, 1:"OUTP?2") -> (6:w1091:errorcluster)  [unwired: 3 in, 1 out]
                      n579 = GPIB Read(0:w1090, 1:3200, 3:w1091) -> (5:w1088:string)  [unwired: 2 in, 2 out]
                      n580 = Fract/Exp String To Number(string=w1088) -> (number=w1087:dbl)  [unwired: 3 in, 1 out]
                      n581 = Build Array (concatenate)(w1093, w1087) -> (w1092:dbl[])
                    }
                  }
                  n582 = property on="array for data" class="Arr (strict)"("Value"=w1083) -> ()  [unwired: 2 in, 2 out]
                }
                frame #7 {
                  # "check if in-phase\nsignal on lock-in \n(address 4) is to\nbe measured"
                  n583 = property on="Addr 4 lock-in" class="Bool (strict)"() -> ("Value"=w1094:bool)  [unwired: 2 in, 2 out]
                  n584 = property on="array for data" class="Arr (strict)"() -> ("Value"=w1096:dbl[])  [unwired: 2 in, 2 out]
                  n585 = case shown="True" w1094 {
                    tunnel: w1096 -> [w1097 w1105]
                    tunnel: [w1097 w1104] -> w1095
                    frame False {
                      # "we are not measuring in phase signal on lock-in (address 4)"
                    }
                    frame True {
                      w1102 = "4"
                      # "we are  measuring lock-in (address 4), in phase"
                      n586 = GPIB Write(0:w1102, 1:"OUTP?1") -> (6:w1103:errorcluster)  [unwired: 3 in, 1 out]
                      n587 = GPIB Read(0:w1102, 1:3200, 3:w1103) -> (5:w1100:string)  [unwired: 2 in, 2 out]
                      n588 = Fract/Exp String To Number(string=w1100) -> (number=w1099:dbl)  [unwired: 3 in, 1 out]
                      n589 = Build Array (concatenate)(w1105, w1099) -> (w1104:dbl[])
                    }
                  }
                  n590 = property on="array for data" class="Arr (strict)"("Value"=w1095) -> ()  [unwired: 2 in, 2 out]
                }
                frame #8 {
                  # "check if out-of-phase\nsignal on lock-in \n(address 4) is to\nbe measured"
                  n591 = property on="Addr 4 lock-in oop" class="Bool (strict)"() -> ("Value"=w1106:bool)  [unwired: 2 in, 2 out]
                  n592 = property on="array for data" class="Arr (strict)"() -> ("Value"=w1108:dbl[])  [unwired: 2 in, 2 out]
                  n593 = case shown="True" w1106 {
                    tunnel: w1108 -> [w1109 w1117]
                    tunnel: [w1109 w1116] -> w1107
                    frame False {
                      # "we are not measuring out-of-phase signal on lock-in (address 4)"
                    }
                    frame True {
                      w1114 = "4"
                      # "we are  measuring lock-in (address 4), out-of-phase"
                      n594 = GPIB Write(0:w1114, 1:"OUTP?2") -> (6:w1115:errorcluster)  [unwired: 3 in, 1 out]
                      n595 = GPIB Read(0:w1114, 1:3200, 3:w1115) -> (5:w1112:string)  [unwired: 2 in, 2 out]
                      n596 = Fract/Exp String To Number(string=w1112) -> (number=w1111:dbl)  [unwired: 3 in, 1 out]
                      n597 = Build Array (concatenate)(w1117, w1111) -> (w1116:dbl[])
                    }
                  }
                  n598 = property on="array for data" class="Arr (strict)"("Value"=w1107) -> ()  [unwired: 2 in, 2 out]
                }
                frame #9 {
                  # "check if in-phase\nsignal on lock-in \n(address 5) is to\nbe measured"
                  n599 = property on="Addr 5 lock-in" class="Bool (strict)"() -> ("Value"=w1118:bool)  [unwired: 2 in, 2 out]
                  n600 = property on="array for data" class="Arr (strict)"() -> ("Value"=w1120:dbl[])  [unwired: 2 in, 2 out]
                  n601 = case shown="False" w1118 {
                    tunnel: w1120 -> [w1121 w1129]
                    tunnel: [w1121 w1128] -> w1119
                    frame False {
                      # "we are not measuring in phase signal on lock-in (address 5)"
                    }
                    frame True {
                      w1126 = "5"
                      # "we are  measuring lock-in (address 5), in phase"
                      n602 = GPIB Write(0:w1126, 1:"OUTP?1") -> (6:w1127:errorcluster)  [unwired: 3 in, 1 out]
                      n603 = GPIB Read(0:w1126, 1:3200, 3:w1127) -> (5:w1124:string)  [unwired: 2 in, 2 out]
                      n604 = Fract/Exp String To Number(string=w1124) -> (number=w1123:dbl)  [unwired: 3 in, 1 out]
                      n605 = Build Array (concatenate)(w1129, w1123) -> (w1128:dbl[])
                    }
                  }
                  n606 = property on="array for data" class="Arr (strict)"("Value"=w1119) -> ()  [unwired: 2 in, 2 out]
                }
                frame #10 {
                  # "check if out-of-phase\nsignal on lock-in \n(address 5) is to\nbe measured"
                  n607 = property on="Addr 5 lock-in oop" class="Bool (strict)"() -> ("Value"=w1130:bool)  [unwired: 2 in, 2 out]
                  n608 = property on="array for data" class="Arr (strict)"() -> ("Value"=w1132:dbl[])  [unwired: 2 in, 2 out]
                  n609 = case shown="False" w1130 {
                    tunnel: w1132 -> [w1133 w1141]
                    tunnel: [w1133 w1140] -> w1131
                    frame False {
                      # "we are not measuring out-of-phase signal on lock-in (address 5)"
                    }
                    frame True {
                      w1138 = "5"
                      # "we are  measuring lock-in (address 5), out-of-phase"
                      n610 = GPIB Write(0:w1138, 1:"OUTP?2") -> (6:w1139:errorcluster)  [unwired: 3 in, 1 out]
                      n611 = GPIB Read(0:w1138, 1:3200, 3:w1139) -> (5:w1136:string)  [unwired: 2 in, 2 out]
                      n612 = Fract/Exp String To Number(string=w1136) -> (number=w1135:dbl)  [unwired: 3 in, 1 out]
                      n613 = Build Array (concatenate)(w1141, w1135) -> (w1140:dbl[])
                    }
                  }
                  n614 = property on="array for data" class="Arr (strict)"("Value"=w1131) -> ()  [unwired: 2 in, 2 out]
                }
                frame #11 {
                  # "check if voltage on \nmain Keithley 2400 \n(addr. 12) is to\nbe measured"
                  n615 = property on="Voltage (Vk1)" class="Bool (strict)"() -> ("Value"=w1142:bool)  [unwired: 2 in, 2 out]
                  n616 = property on="array for data" class="Arr (strict)"() -> ("Value"=w1144:dbl[])  [unwired: 2 in, 2 out]
                  n617 = case shown="False" w1142 {
                    tunnel: w1144 -> [w1145 w1155]
                    tunnel: [w1145 w1154] -> w1143
                    frame False {
                      # "we aren't measuring voltage \non main Keithley 2400 (addr. 12)"
                    }
                    frame True {
                      w1152 = "12"
                      # "we are measuring voltage \non main Keithley 2400 (addr. 12)"
                      n618 = GPIB Write(0:w1152, 1:":READ?") -> (6:w1153:errorcluster)  [unwired: 3 in, 1 out]
                      n619 = GPIB Read(0:w1152, 1:3200, 3:w1153) -> (5:w1148:string)  [unwired: 2 in, 2 out]
                      n620 = String Subset(string=w1148, length (rest)=13) -> (substring=w1147:string)  [unwired: 1 in]
                      n621 = Fract/Exp String To Number(string=w1147) -> (number=w1150:dbl)  [unwired: 3 in, 1 out]
                      n622 = Build Array (concatenate)(w1155, w1150) -> (w1154:dbl[])
                    }
                  }
                  n623 = property on="array for data" class="Arr (strict)"("Value"=w1143) -> ()  [unwired: 2 in, 2 out]
                }
                frame #12 {
                  # "check if  current on \nmain Keithley 2400 \n(addr. 12) is to\nbe measured"
                  n624 = property on="Current (Ik1)" class="Bool (strict)"() -> ("Value"=w1156:bool)  [unwired: 2 in, 2 out]
                  n625 = property on="array for data" class="Arr (strict)"() -> ("Value"=w1158:dbl[])  [unwired: 2 in, 2 out]
                  n626 = case shown="True" w1156 {
                    tunnel: w1158 -> [w1159 w1170]
                    tunnel: [w1159 w1169] -> w1157
                    frame False {
                      # "we aren't measuring current \non main Keithley 2400 (addr. 12)"
                    }
                    frame True {
                      w1167 = "12"
                      # "we are measuring current\non main Keithley 2400 (addr. 12)"
                      n627 = GPIB Write(0:w1167, 1:":READ?") -> (6:w1168:errorcluster)  [unwired: 3 in, 1 out]
                      n628 = GPIB Read(0:w1167, 1:3200, 3:w1168) -> (5:w1163:string)  [unwired: 2 in, 2 out]
                      n629 = String Subset(string=w1163, offset (0)=14, length (rest)=13) -> (substring=w1162:string)
                      n630 = Fract/Exp String To Number(string=w1162) -> (number=w1165:dbl)  [unwired: 3 in, 1 out]
                      n631 = Build Array (concatenate)(w1170, w1165) -> (w1169:dbl[])
                    }
                  }
                  n632 = property on="array for data" class="Arr (strict)"("Value"=w1157) -> ()  [unwired: 2 in, 2 out]
                }
                frame #13 {
                  # "check if voltage on \nadd. Keithley 2400 \n(addr. 13) is to\nbe measured"
                  n633 = property on="Voltage (Vk2)" class="Bool (strict)"() -> ("Value"=w1171:bool)  [unwired: 2 in, 2 out]
                  n634 = property on="array for data" class="Arr (strict)"() -> ("Value"=w1173:dbl[])  [unwired: 2 in, 2 out]
                  n635 = case shown="True" w1171 {
                    tunnel: w1173 -> [w1174 w1184]
                    tunnel: [w1174 w1183] -> w1172
                    frame False {
                      # "we aren't measuring voltage \non additional Keithley 2400 (addr. 13)"
                    }
                    frame True {
                      w1181 = "13"
                      # "we are measuring voltage \non additional Keithley 2400 (addr. 13)"
                      n636 = GPIB Write(0:w1181, 1:":READ?") -> (6:w1182:errorcluster)  [unwired: 3 in, 1 out]
                      n637 = GPIB Read(0:w1181, 1:3200, 3:w1182) -> (5:w1177:string)  [unwired: 2 in, 2 out]
                      n638 = String Subset(string=w1177, length (rest)=13) -> (substring=w1176:string)  [unwired: 1 in]
                      n639 = Fract/Exp String To Number(string=w1176) -> (number=w1179:dbl)  [unwired: 3 in, 1 out]
                      n640 = Build Array (concatenate)(w1184, w1179) -> (w1183:dbl[])
                    }
                  }
                  n641 = property on="array for data" class="Arr (strict)"("Value"=w1172) -> ()  [unwired: 2 in, 2 out]
                }
                frame #14 {
                  # "check if  current on \nadd. Keithley 2400 \n(addr. 13) is to\nbe measured"
                  n642 = property on="Current (Ik2)" class="Bool (strict)"() -> ("Value"=w1185:bool)  [unwired: 2 in, 2 out]
                  n643 = property on="array for data" class="Arr (strict)"() -> ("Value"=w1187:dbl[])  [unwired: 2 in, 2 out]
                  n644 = case shown="True" w1185 {
                    tunnel: w1187 -> [w1188 w1199]
                    tunnel: [w1188 w1198] -> w1186
                    frame False {
                      # "we aren't measuring current \non additional Keithley 2400 (addr. 13)"
                    }
                    frame True {
                      w1196 = "13"
                      # "we are measuring current\non additional Keithley 2400 (addr. 13)"
                      n645 = GPIB Write(0:w1196, 1:":READ?") -> (6:w1197:errorcluster)  [unwired: 3 in, 1 out]
                      n646 = GPIB Read(0:w1196, 1:3200, 3:w1197) -> (5:w1192:string)  [unwired: 2 in, 2 out]
                      n647 = String Subset(string=w1192, offset (0)=14, length (rest)=13) -> (substring=w1191:string)
                      n648 = Fract/Exp String To Number(string=w1191) -> (number=w1194:dbl)  [unwired: 3 in, 1 out]
                      n649 = Build Array (concatenate)(w1199, w1194) -> (w1198:dbl[])
                    }
                  }
                  n650 = property on="array for data" class="Arr (strict)"("Value"=w1186) -> ()  [unwired: 2 in, 2 out]
                }
                frame #15 {
                  # "check if voltage on \nadd. Keithley 2400 \n(addr. 14) is to\nbe measured"
                  n651 = property on="Voltage (Vk3)" class="Bool (strict)"() -> ("Value"=w1200:bool)  [unwired: 2 in, 2 out]
                  n652 = property on="array for data" class="Arr (strict)"() -> ("Value"=w1202:dbl[])  [unwired: 2 in, 2 out]
                  n653 = case shown="False" w1200 {
                    tunnel: w1202 -> [w1203 w1213]
                    tunnel: [w1203 w1212] -> w1201
                    frame False {
                      # "we aren't measuring voltage \non additional Keithley 2400 (addr. 14)"
                    }
                    frame True {
                      w1210 = "14"
                      # "we are measuring voltage \non additional Keithley 2400 (addr. 14)"
                      n654 = GPIB Write(0:w1210, 1:":READ?") -> (6:w1211:errorcluster)  [unwired: 3 in, 1 out]
                      n655 = GPIB Read(0:w1210, 1:3200, 3:w1211) -> (5:w1206:string)  [unwired: 2 in, 2 out]
                      n656 = String Subset(string=w1206, length (rest)=13) -> (substring=w1205:string)  [unwired: 1 in]
                      n657 = Fract/Exp String To Number(string=w1205) -> (number=w1208:dbl)  [unwired: 3 in, 1 out]
                      n658 = Build Array (concatenate)(w1213, w1208) -> (w1212:dbl[])
                    }
                  }
                  n659 = property on="array for data" class="Arr (strict)"("Value"=w1201) -> ()  [unwired: 2 in, 2 out]
                }
                frame #16 {
                  # "check if  current on \nadd. Keithley 2400 \n(addr. 14) is to\nbe measured"
                  n660 = property on="Current (Ik3)" class="Bool (strict)"() -> ("Value"=w1214:bool)  [unwired: 2 in, 2 out]
                  n661 = property on="array for data" class="Arr (strict)"() -> ("Value"=w1216:dbl[])  [unwired: 2 in, 2 out]
                  n662 = case shown="True" w1214 {
                    tunnel: w1216 -> [w1217 w1228]
                    tunnel: [w1217 w1227] -> w1215
                    frame False {
                      # "we aren't measuring current \non additional Keithley 2400 (addr. 14)"
                    }
                    frame True {
                      w1225 = "14"
                      # "we are measuring current\non additional Keithley 2400 (addr. 14)"
                      n663 = GPIB Write(0:w1225, 1:":READ?") -> (6:w1226:errorcluster)  [unwired: 3 in, 1 out]
                      n664 = GPIB Read(0:w1225, 1:3200, 3:w1226) -> (5:w1221:string)  [unwired: 2 in, 2 out]
                      n665 = String Subset(string=w1221, offset (0)=14, length (rest)=13) -> (substring=w1220:string)
                      n666 = Fract/Exp String To Number(string=w1220) -> (number=w1223:dbl)  [unwired: 3 in, 1 out]
                      n667 = Build Array (concatenate)(w1228, w1223) -> (w1227:dbl[])
                    }
                  }
                  n668 = property on="array for data" class="Arr (strict)"("Value"=w1215) -> ()  [unwired: 2 in, 2 out]
                }
                frame #17 {
                  # "check if 1st channel\non Keithley 2182 \n(addr. 15) is to\nbe measured"
                  n669 = property on="Channel 1 (Vnano1)" class="Bool (strict)"() -> ("Value"=w1229:bool)  [unwired: 2 in, 2 out]
                  n670 = property on="array for data" class="Arr (strict)"() -> ("Value"=w1231:dbl[])  [unwired: 2 in, 2 out]
                  n671 = case shown="True" w1229 {
                    tunnel: w1231 -> [w1232 w1240]
                    tunnel: [w1232 w1239] -> w1230
                    frame False {
                      # "we are not measuring 1st channel\non Keithley 2182 (addr. 15)"
                    }
                    frame True {
                      w1237 = "15"
                      # "we are measuring 1st channel\non Keithley 2182 (addr. 15)"
                      n672 = GPIB Write(0:w1237, 1:":SENSe:DATA:FRES?") -> (6:w1238:errorcluster)  [unwired: 3 in, 1 out]
                      n673 = GPIB Read(0:w1237, 1:200, 3:w1238) -> (5:w1233:string)  [unwired: 2 in, 2 out]
                      n674 = Fract/Exp String To Number(string=w1233) -> (number=w1235:dbl)  [unwired: 3 in, 1 out]
                      n675 = Build Array (concatenate)(w1240, w1235) -> (w1239:dbl[])
                    }
                  }
                  n676 = property on="array for data" class="Arr (strict)"("Value"=w1230) -> ()  [unwired: 2 in, 2 out]
                }
                frame #18 {
                  # "check if 2nd channel\non Keithley 2182 \n(addr. 15) is to\nbe measured"
                  n677 = property on="Channel 2 (Vnano1b)" class="Bool (strict)"() -> ("Value"=w1241:bool)  [unwired: 2 in, 2 out]
                  n678 = property on="array for data" class="Arr (strict)"() -> ("Value"=w1243:dbl[])  [unwired: 2 in, 2 out]
                  n679 = case shown="False" w1241 {
                    tunnel: w1243 -> [w1244 w1256]
                    tunnel: [w1244 w1255] -> w1242
                    frame False {
                      # "we are not measuring 1st channel\non Keithley 2182 (addr. 15)"
                    }
                    frame True {
                      w1247 = "15"
                      # "switching to channel 2 and then\nback to channel 1"
                      # "we are measuring 2nd channel\non Keithley 2182 (addr. 15)"
                      n680 = GPIB Write(0:w1247, 1:":SENSe:CHAN 2") -> (6:w1248:errorcluster)  [unwired: 3 in, 1 out]
                      n681 = GPIB Write(0:w1247, 1:":SENSe:DATA:FRES?", 3:w1248) -> (6:w1254:errorcluster)  [unwired: 2 in, 1 out]
                      n682 = GPIB Read(0:w1247, 1:200, 3:w1254) -> (5:w1250:string, 7:w1246:errorcluster)  [unwired: 2 in, 1 out]
                      n683 = GPIB Write(0:w1247, 1:":SENSe:CHAN 1", 3:w1246) -> ()  [unwired: 2 in, 2 out]
                      n684 = Fract/Exp String To Number(string=w1250) -> (number=w1252:dbl)  [unwired: 3 in, 1 out]
                      n685 = Build Array (concatenate)(w1256, w1252) -> (w1255:dbl[])
                    }
                  }
                  n686 = property on="array for data" class="Arr (strict)"("Value"=w1242) -> ()  [unwired: 2 in, 2 out]
                }
                frame #19 {
                  # "check if 1st channel\non Keithley 2182 \n(addr. 16) is to\nbe measured"
                  n687 = property on="Channel 1 (Vnano2)" class="Bool (strict)"() -> ("Value"=w1257:bool)  [unwired: 2 in, 2 out]
                  n688 = property on="array for data" class="Arr (strict)"() -> ("Value"=w1259:dbl[])  [unwired: 2 in, 2 out]
                  n689 = case shown="True" w1257 {
                    tunnel: w1259 -> [w1260 w1268]
                    tunnel: [w1260 w1267] -> w1258
                    frame False {
                      # "we are not measuring 1st channel\non Keithley 2182 (addr. 16)"
                    }
                    frame True {
                      w1265 = "16"
                      # "we are measuring 1st channel\non Keithley 2182 (addr. 16)"
                      n690 = GPIB Write(0:w1265, 1:":SENSe:DATA:FRES?") -> (6:w1266:errorcluster)  [unwired: 3 in, 1 out]
                      n691 = GPIB Read(0:w1265, 1:200, 3:w1266) -> (5:w1261:string)  [unwired: 2 in, 2 out]
                      n692 = Fract/Exp String To Number(string=w1261) -> (number=w1263:dbl)  [unwired: 3 in, 1 out]
                      n693 = Build Array (concatenate)(w1268, w1263) -> (w1267:dbl[])
                    }
                  }
                  n694 = property on="array for data" class="Arr (strict)"("Value"=w1258) -> ()  [unwired: 2 in, 2 out]
                }
                frame #20 {
                  # "check if 2nd channel\non Keithley 2182 \n(addr. 16) is to\nbe measured"
                  n695 = property on="Channel 2 (Vnano2b)" class="Bool (strict)"() -> ("Value"=w1269:bool)  [unwired: 2 in, 2 out]
                  n696 = property on="array for data" class="Arr (strict)"() -> ("Value"=w1271:dbl[])  [unwired: 2 in, 2 out]
                  n697 = case shown="True" w1269 {
                    tunnel: w1271 -> [w1272 w1284]
                    tunnel: [w1272 w1283] -> w1270
                    frame False {
                      # "we are not measuring 1st channel\non Keithley 2182 (addr. 16)"
                    }
                    frame True {
                      w1275 = "16"
                      # "switching to channel 2 and then\nback to channel 1"
                      # "we are measuring 2nd channel\non Keithley 2182 (addr. 16)"
                      n698 = GPIB Write(0:w1275, 1:":SENSe:CHAN 2") -> (6:w1276:errorcluster)  [unwired: 3 in, 1 out]
                      n699 = GPIB Write(0:w1275, 1:":SENSe:DATA:FRES?", 3:w1276) -> (6:w1282:errorcluster)  [unwired: 2 in, 1 out]
                      n700 = GPIB Read(0:w1275, 1:200, 3:w1282) -> (5:w1278:string, 7:w1274:errorcluster)  [unwired: 2 in, 1 out]
                      n701 = GPIB Write(0:w1275, 1:":SENSe:CHAN 1", 3:w1274) -> ()  [unwired: 2 in, 2 out]
                      n702 = Fract/Exp String To Number(string=w1278) -> (number=w1280:dbl)  [unwired: 3 in, 1 out]
                      n703 = Build Array (concatenate)(w1284, w1280) -> (w1283:dbl[])
                    }
                  }
                  n704 = property on="array for data" class="Arr (strict)"("Value"=w1270) -> ()  [unwired: 2 in, 2 out]
                }
                frame #21 {
                  # "check if 1st channel\non Keithley 2182 \n(addr. 17) is to\nbe measured"
                  n705 = property on="Channel 1 (Vnano3)" class="Bool (strict)"() -> ("Value"=w1285:bool)  [unwired: 2 in, 2 out]
                  n706 = property on="array for data" class="Arr (strict)"() -> ("Value"=w1287:dbl[])  [unwired: 2 in, 2 out]
                  n707 = case shown="True" w1285 {
                    tunnel: w1287 -> [w1288 w1296]
                    tunnel: [w1288 w1295] -> w1286
                    frame False {
                      # "we are not measuring 1st channel\non Keithley 2182 (addr. 17)"
                    }
                    frame True {
                      w1293 = "17"
                      # "we are measuring 1st channel\non Keithley 2182 (addr. 17)"
                      n708 = GPIB Write(0:w1293, 1:":SENSe:DATA:FRES?") -> (6:w1294:errorcluster)  [unwired: 3 in, 1 out]
                      n709 = GPIB Read(0:w1293, 1:200, 3:w1294) -> (5:w1289:string)  [unwired: 2 in, 2 out]
                      n710 = Fract/Exp String To Number(string=w1289) -> (number=w1291:dbl)  [unwired: 3 in, 1 out]
                      n711 = Build Array (concatenate)(w1296, w1291) -> (w1295:dbl[])
                    }
                  }
                  n712 = property on="array for data" class="Arr (strict)"("Value"=w1286) -> ()  [unwired: 2 in, 2 out]
                }
                frame #22 {
                  # "check if 2nd channel\non Keithley 2182 \n(addr. 17) is to\nbe measured"
                  n713 = property on="Channel 2 (Vnano3b)" class="Bool (strict)"() -> ("Value"=w1297:bool)  [unwired: 2 in, 2 out]
                  n714 = property on="array for data" class="Arr (strict)"() -> ("Value"=w1299:dbl[])  [unwired: 2 in, 2 out]
                  n715 = case shown="True" w1297 {
                    tunnel: w1299 -> [w1300 w1312]
                    tunnel: [w1300 w1311] -> w1298
                    frame False {
                      # "we are not measuring 1st channel\non Keithley 2182 (addr. 17)"
                    }
                    frame True {
                      w1303 = "17"
                      # "switching to channel 2 and then\nback to channel 1"
                      # "we are measuring 2nd channel\non Keithley 2182 (addr. 17)"
                      n716 = GPIB Write(0:w1303, 1:":SENSe:CHAN 2") -> (6:w1304:errorcluster)  [unwired: 3 in, 1 out]
                      n717 = GPIB Write(0:w1303, 1:":SENSe:DATA:FRES?", 3:w1304) -> (6:w1310:errorcluster)  [unwired: 2 in, 1 out]
                      n718 = GPIB Read(0:w1303, 1:200, 3:w1310) -> (5:w1306:string, 7:w1302:errorcluster)  [unwired: 2 in, 1 out]
                      n719 = GPIB Write(0:w1303, 1:":SENSe:CHAN 1", 3:w1302) -> ()  [unwired: 2 in, 2 out]
                      n720 = Fract/Exp String To Number(string=w1306) -> (number=w1308:dbl)  [unwired: 3 in, 1 out]
                      n721 = Build Array (concatenate)(w1312, w1308) -> (w1311:dbl[])
                    }
                  }
                  n722 = property on="array for data" class="Arr (strict)"("Value"=w1298) -> ()  [unwired: 2 in, 2 out]
                }
                frame #23 {
                  # "check if 1st \nthermometer on \nOxford ITC \n(address 24) \nis measured"
                  n723 = property on="Thermometer 1 (T1)" class="Bool (strict)"() -> ("Value"=w1313:bool)  [unwired: 2 in, 2 out]
                  n724 = property on="array for data" class="Arr (strict)"() -> ("Value"=w1315:dbl[])  [unwired: 2 in, 2 out]
                  n725 = case shown="True" w1313 {
                    tunnel: w1315 -> [w1316 w1325]
                    tunnel: [w1316 w1324] -> w1314
                    frame False {
                      # "we are not measuring temperature on\nthermometer 1 (addr. 24)"
                    }
                    frame True {
                      w1317 = 1
                      w1322 = "24"
                      # "we are measuring temperature,\nthermometer 1 (addr. 24)"
                      n726 = GPIB Write(0:w1322, 1:"R 1", 2:w1317) -> (6:w1323:errorcluster)  [unwired: 2 in, 1 out]
                      n727 = GPIB Read(0:w1322, 1:200, 2:w1317, 3:w1323) -> (5:w1318:string)  [unwired: 1 in, 2 out]
                      n728 = Fract/Exp String To Number(string=w1318, offset=w1317) -> (number=w1320:dbl)  [unwired: 2 in, 1 out]
                      n729 = Build Array (concatenate)(w1325, w1320) -> (w1324:dbl[])
                    }
                  }
                  n730 = property on="array for data" class="Arr (strict)"("Value"=w1314) -> ()  [unwired: 2 in, 2 out]
                }
                frame #24 {
                  # "check if 1st \nthermometer on \nOxford ITC \n(address 24) \nis measured"
                  n731 = property on="Magnetic Field (B)" class="Bool (strict)"() -> ("Value"=w1326:bool)  [unwired: 2 in, 2 out]
                  n732 = property on="array for data" class="Arr (strict)"() -> ("Value"=w1328:dbl[])  [unwired: 2 in, 2 out]
                  n733 = case shown="True" w1326 {
                    tunnel: w1328 -> [w1329 w1338]
                    tunnel: [w1329 w1337] -> w1327
                    frame False {
                      # "we are not measuringmagnetic field (addr. 25)"
                    }
                    frame True {
                      w1330 = 1
                      w1335 = "25"
                      # "we are measuring magnetic field  (addr. 25)"
                      n734 = GPIB Write(0:w1335, 1:"R 8", 2:w1330) -> (6:w1336:errorcluster)  [unwired: 2 in, 1 out]
                      n735 = GPIB Read(0:w1335, 1:200, 2:w1330, 3:w1336) -> (5:w1331:string)  [unwired: 1 in, 2 out]
                      n736 = Fract/Exp String To Number(string=w1331, offset=w1330) -> (number=w1333:dbl)  [unwired: 2 in, 1 out]
                      n737 = Build Array (concatenate)(w1338, w1333) -> (w1337:dbl[])
                    }
                  }
                  n738 = property on="array for data" class="Arr (strict)"("Value"=w1327) -> ()  [unwired: 2 in, 2 out]
                }
                frame #25 {
                  # "check if capacitance\nand loss (address 28)\nare measured"
                  n739 = property on="Capacitance (C) and Loss (L)" class="Bool (strict)"() -> ("Value"=w1339:bool)  [unwired: 2 in, 2 out]
                  n740 = property on="array for data" class="Arr (strict)"() -> ("Value"=w1341:dbl[])  [unwired: 2 in, 2 out]
                  n741 = case shown="True" w1339 {
                    tunnel: w1341 -> [w1342 w1348]
                    tunnel: [w1342 w1344] -> w1340
                    frame False {
                      # "we are not measuringmagnetic capacitance (addr. 28)"
                    }
                    frame True {
                      # "we are measuring capacitance and loss  (addr. 28)"
                      n742 = stacked-sequence {
                        seq-local: [w1350 _ _] -> [_ _ w1373]
                        tunnel: [_ _ w1367] -> w1343
                        tunnel: [_ _ w1368] -> w1346
                        tunnel: "28" ("data") -> [w1349 w1353 w1362]
                        frame #0 {
                          n743 = GPIB Write(0:w1349, 1:"SINGLE" ("data"), 2:i16 0 ("mode (0)")) -> (6:w1350:errorcluster)  [unwired: 2 in, 1 out]
                        }
                        frame #1 {
                          n744 = while {
                            tunnel: w1353 -> [w1354]
                            i -> [w1355]
                            stop <- w1357 continue-if-true
                            n745 = GPIB Serial Poll(0:w1354) -> (2:w1359:i16)  [unwired: 1 in, 2 out]
                            n746 = Less?(x=w1359, y=i16 128) -> (x < y?=w1357:bool)
                            n747 = Wait (ms)(milliseconds to wait=u32 50) -> ()  [unwired: 1 out]
                            "Numeric 4" <- w1355
                          }
                        }
                        frame #2 {
                          w1360 = i16 2 ("mode (0)")
                          n748 = GPIB Read(0:w1362, 1:200 ("byte count"), 2:i16 2 ("mode (0)"), 3:w1373) -> (5:w1366:string)  [unwired: 1 in, 2 out]
                          n749 = Match Pattern(string=w1366, regular expression="C=") -> (after substring=w1365:string)  [unwired: 1 in, 3 out]
                          n750 = Match Pattern(string=w1365, regular expression="PF L=") -> (after substring=w1363:string)  [unwired: 1 in, 3 out]
                          n751 = Search/Split String(string=w1365, search string/char (-)=" ", offset (0)=w1360) -> (substring before match=w1370:string)  [unwired: 2 out]
                          n752 = Search/Split String(string=w1363, search string/char (-)=" ", offset (0)=w1360) -> (substring before match=w1369:string)  [unwired: 2 out]
                          n753 = Fract/Exp String To Number(string=w1369) -> (number=w1367:dbl)  [unwired: 3 in, 1 out]
                          n754 = Fract/Exp String To Number(string=w1370) -> (number=w1368:dbl)  [unwired: 3 in, 1 out]
                        }
                      }
                      n755 = Build Array (concatenate)(w1348, w1346) -> (w1345:dbl[])
                      n756 = Build Array (concatenate)(w1345, w1343) -> (w1344:dbl[])
                    }
                  }
                  n757 = property on="array for data" class="Arr (strict)"("Value"=w1340) -> ()  [unwired: 2 in, 2 out]
                }
              }
              n758 = property on="Commute SorceMeter" class="RadioBtnsControl (strict)"() -> ("Value"=w988:enum32{"Radio Selection 1", "Radio Selection 2"})  [unwired: 2 in, 2 out]
              n759 = case shown="\"Radio Selection 1\", Default" w988 {
                tunnel: ["13" "14"] -> w991
                frame "Radio Selection 1", Default {
                }
                frame "Radio Selection 2" {
                }
              }
              n760 = GPIB Write(0:w991, 1:":READ?", 3:w990) -> (6:w992:errorcluster)  [unwired: 2 in, 1 out]
              n761 = GPIB Read(0:w991, 1:3200, 3:w992) -> (5:w995:string)  [unwired: 2 in, 2 out]
              n762 = String Subset(string=w995, length (rest)=13) -> (substring=w996:string)  [unwired: 1 in]
              n763 = Fract/Exp String To Number(string=w996) -> (number=w998:dbl)  [unwired: 3 in, 1 out]
              n764 = Multiply(x=w998, y=-1.0) -> (x*y=w1003:dbl)
              n765 = Number To Fractional String(number=w1003) -> (F-format string=w1000:string)  [unwired: 3 in]
              n766 = Concatenate Strings(":INIT:IMM; :SOUR:VOLT:LEV:IMM:AMPL " ("data"), w1000) -> (w1001:string)
              n767 = GPIB Write(0:w991, 1:w1001) -> (6:w989:errorcluster)  [unwired: 3 in, 1 out]
            }
          }
        }
        frame False {
          # "all measurements are done in this stacked sequence; reading from each device is recorded to \"array for data\""
          n768 = stacked-sequence {
            tunnel: w1376 -> [w1378 _ _ _ _ _ _ _ _ _ _ _ _ _ _ _ _ _ _ _ _ _ _ _ _ _]
            tunnel: [w1378 _ _ _ _ _ _ _ _ _ _ _ _ _ _ _ _ _ _ _ _ _ _ _ _ _] -> w1377
            frame #0 {
              # "check if oscillator on \nlock-in (address 1)\nis to be measured"
              n769 = property on="Current is:" class="RadioBtnsControl (strict)"() -> ("Value"=w1381:T1)  [unwired: 2 in, 2 out]
              n770 = property on="array for data" class="Arr (strict)"() -> ("Value"=w1380:dbl[])  [unwired: 2 in, 2 out]
              n771 = Equal?(x=w1381, y=1) -> (x = y?=w1382:bool)
              n772 = case shown="True" w1382 {
                tunnel: w1380 -> [w1384 w1392]
                tunnel: [w1384 w1391] -> w1379
                frame False {
                  # "we are not measuring oscillator from\nlock-in (address 1)"
                }
                frame True {
                  w1388 = "1"
                  # "we are  measuring oscillator"
                  n773 = GPIB Write(0:w1388, 1:"SLVL?") -> (6:w1389:errorcluster)  [unwired: 3 in, 1 out]
                  n774 = GPIB Read(0:w1388, 1:3200, 3:w1389) -> (5:w1386:string)  [unwired: 2 in, 2 out]
                  n775 = Fract/Exp String To Number(string=w1386) -> (number=w1385:dbl)  [unwired: 3 in, 1 out]
                  n776 = Build Array (concatenate)(w1392, w1385) -> (w1391:dbl[])
                }
              }
              n777 = property on="array for data" class="Arr (strict)"("Value"=w1379) -> ()  [unwired: 2 in, 2 out]
            }
            frame #1 {
              # "check if in-phase\nsignal on lock-in \n(address 1) is to\nbe measured"
              n778 = property on="array for data" class="Arr (strict)"() -> ("Value"=w1395:dbl[])  [unwired: 2 in, 2 out]
              n779 = property on="Addr 1 lock-in" class="Bool (strict)"() -> ("Value"=w1393:bool)  [unwired: 2 in, 2 out]
              n780 = case shown="True" w1393 {
                tunnel: w1395 -> [w1396 w1404]
                tunnel: [w1396 w1403] -> w1394
                frame False {
                  # "we are not measuring in phase signal on lock-in (address 1)"
                }
                frame True {
                  w1401 = "1"
                  # "we are  measuring lock-in (address 1), in phase"
                  n781 = GPIB Write(0:w1401, 1:"OUTP?1") -> (6:w1402:errorcluster)  [unwired: 3 in, 1 out]
                  n782 = GPIB Read(0:w1401, 1:3200, 3:w1402) -> (5:w1399:string)  [unwired: 2 in, 2 out]
                  n783 = Fract/Exp String To Number(string=w1399) -> (number=w1398:dbl)  [unwired: 3 in, 1 out]
                  n784 = Build Array (concatenate)(w1404, w1398) -> (w1403:dbl[])
                }
              }
              n785 = property on="array for data" class="Arr (strict)"("Value"=w1394) -> ()  [unwired: 2 in, 2 out]
            }
            frame #2 {
              # "check if out-of-phase\nsignal on lock-in \n(address 1) is to\nbe measured"
              n786 = property on="Addr 1 lock-in oop" class="Bool (strict)"() -> ("Value"=w1405:bool)  [unwired: 2 in, 2 out]
              n787 = property on="array for data" class="Arr (strict)"() -> ("Value"=w1407:dbl[])  [unwired: 2 in, 2 out]
              n788 = case shown="False" w1405 {
                tunnel: w1407 -> [w1408 w1416]
                tunnel: [w1408 w1415] -> w1406
                frame False {
                  # "we are not measuring out-of-phase signal on lock-in (address 1)"
                }
                frame True {
                  w1413 = "1"
                  # "we are  measuring lock-in (address 1), out-of-phase signal"
                  n789 = GPIB Write(0:w1413, 1:"OUTP?2") -> (6:w1414:errorcluster)  [unwired: 3 in, 1 out]
                  n790 = GPIB Read(0:w1413, 1:3200, 3:w1414) -> (5:w1411:string)  [unwired: 2 in, 2 out]
                  n791 = Fract/Exp String To Number(string=w1411) -> (number=w1410:dbl)  [unwired: 3 in, 1 out]
                  n792 = Build Array (concatenate)(w1416, w1410) -> (w1415:dbl[])
                }
              }
              n793 = property on="array for data" class="Arr (strict)"("Value"=w1406) -> ()  [unwired: 2 in, 2 out]
            }
            frame #3 {
              # "check if in-phase\nsignal on lock-in \n(address 2) is to\nbe measured"
              n794 = property on="Addr 2 lock-in" class="Bool (strict)"() -> ("Value"=w1417:bool)  [unwired: 2 in, 2 out]
              n795 = property on="array for data" class="Arr (strict)"() -> ("Value"=w1419:dbl[])  [unwired: 2 in, 2 out]
              n796 = case shown="False" w1417 {
                tunnel: w1419 -> [w1420 w1428]
                tunnel: [w1420 w1427] -> w1418
                frame False {
                  # "we are not measuring in phase signal on lock-in (address 2)"
                }
                frame True {
                  w1425 = "2"
                  # "we are  measuring lock-in (address 2), in phase"
                  n797 = GPIB Write(0:w1425, 1:"OUTP?1") -> (6:w1426:errorcluster)  [unwired: 3 in, 1 out]
                  n798 = GPIB Read(0:w1425, 1:3200, 3:w1426) -> (5:w1423:string)  [unwired: 2 in, 2 out]
                  n799 = Fract/Exp String To Number(string=w1423) -> (number=w1422:dbl)  [unwired: 3 in, 1 out]
                  n800 = Build Array (concatenate)(w1428, w1422) -> (w1427:dbl[])
                }
              }
              n801 = property on="array for data" class="Arr (strict)"("Value"=w1418) -> ()  [unwired: 2 in, 2 out]
            }
            frame #4 {
              # "check if out-of-phase\nsignal on lock-in \n(address 2) is to\nbe measured"
              n802 = property on="Addr 2 lock-in oop" class="Bool (strict)"() -> ("Value"=w1429:bool)  [unwired: 2 in, 2 out]
              n803 = property on="array for data" class="Arr (strict)"() -> ("Value"=w1431:dbl[])  [unwired: 2 in, 2 out]
              n804 = case shown="False" w1429 {
                tunnel: w1431 -> [w1432 w1440]
                tunnel: [w1432 w1439] -> w1430
                tunnel: w1429 -> [_ _]
                frame False {
                  # "we are not measuring out-of-phase signal on lock-in (address 2)"
                }
                frame True {
                  w1437 = "2"
                  # "we are  measuring lock-in (address 2), out-of-phase"
                  n805 = GPIB Write(0:w1437, 1:"OUTP?2") -> (6:w1438:errorcluster)  [unwired: 3 in, 1 out]
                  n806 = GPIB Read(0:w1437, 1:3200, 3:w1438) -> (5:w1435:string)  [unwired: 2 in, 2 out]
                  n807 = Fract/Exp String To Number(string=w1435) -> (number=w1434:dbl)  [unwired: 3 in, 1 out]
                  n808 = Build Array (concatenate)(w1440, w1434) -> (w1439:dbl[])
                }
              }
              n809 = property on="array for data" class="Arr (strict)"("Value"=w1430) -> ()  [unwired: 2 in, 2 out]
            }
            frame #5 {
              # "check if in-phase\nsignal on lock-in \n(address 3) is to\nbe measured"
              n810 = property on="Addr 3 lock-in" class="Bool (strict)"() -> ("Value"=w1441:bool)  [unwired: 2 in, 2 out]
              n811 = property on="array for data" class="Arr (strict)"() -> ("Value"=w1443:dbl[])  [unwired: 2 in, 2 out]
              n812 = case shown="False" w1441 {
                tunnel: w1443 -> [w1444 w1452]
                tunnel: [w1444 w1451] -> w1442
                frame False {
                  # "we are not measuring in phase signal on lock-in (address 3)"
                }
                frame True {
                  w1449 = "3"
                  # "we are  measuring lock-in (address 3), in phase"
                  n813 = GPIB Write(0:w1449, 1:"OUTP?1") -> (6:w1450:errorcluster)  [unwired: 3 in, 1 out]
                  n814 = GPIB Read(0:w1449, 1:3200, 3:w1450) -> (5:w1447:string)  [unwired: 2 in, 2 out]
                  n815 = Fract/Exp String To Number(string=w1447) -> (number=w1446:dbl)  [unwired: 3 in, 1 out]
                  n816 = Build Array (concatenate)(w1452, w1446) -> (w1451:dbl[])
                }
              }
              n817 = property on="array for data" class="Arr (strict)"("Value"=w1442) -> ()  [unwired: 2 in, 2 out]
            }
            frame #6 {
              # "check if out-of-phase\nsignal on lock-in \n(address 3) is to\nbe measured"
              n818 = property on="Addr 3 lock-in oop" class="Bool (strict)"() -> ("Value"=w1453:bool)  [unwired: 2 in, 2 out]
              n819 = property on="array for data" class="Arr (strict)"() -> ("Value"=w1455:dbl[])  [unwired: 2 in, 2 out]
              n820 = case shown="False" w1453 {
                tunnel: w1455 -> [w1456 w1464]
                tunnel: [w1456 w1463] -> w1454
                frame False {
                  # "we are not measuring out-of-phase signal on lock-in (address 3)"
                }
                frame True {
                  w1461 = "3"
                  # "we are  measuring lock-in (address 3), out-of-phase"
                  n821 = GPIB Write(0:w1461, 1:"OUTP?2") -> (6:w1462:errorcluster)  [unwired: 3 in, 1 out]
                  n822 = GPIB Read(0:w1461, 1:3200, 3:w1462) -> (5:w1459:string)  [unwired: 2 in, 2 out]
                  n823 = Fract/Exp String To Number(string=w1459) -> (number=w1458:dbl)  [unwired: 3 in, 1 out]
                  n824 = Build Array (concatenate)(w1464, w1458) -> (w1463:dbl[])
                }
              }
              n825 = property on="array for data" class="Arr (strict)"("Value"=w1454) -> ()  [unwired: 2 in, 2 out]
            }
            frame #7 {
              # "check if in-phase\nsignal on lock-in \n(address 4) is to\nbe measured"
              n826 = property on="Addr 4 lock-in" class="Bool (strict)"() -> ("Value"=w1465:bool)  [unwired: 2 in, 2 out]
              n827 = property on="array for data" class="Arr (strict)"() -> ("Value"=w1467:dbl[])  [unwired: 2 in, 2 out]
              n828 = case shown="False" w1465 {
                tunnel: w1467 -> [w1468 w1476]
                tunnel: [w1468 w1475] -> w1466
                frame False {
                  # "we are not measuring in phase signal on lock-in (address 4)"
                }
                frame True {
                  w1473 = "4"
                  # "we are  measuring lock-in (address 4), in phase"
                  n829 = GPIB Write(0:w1473, 1:"OUTP?1") -> (6:w1474:errorcluster)  [unwired: 3 in, 1 out]
                  n830 = GPIB Read(0:w1473, 1:3200, 3:w1474) -> (5:w1471:string)  [unwired: 2 in, 2 out]
                  n831 = Fract/Exp String To Number(string=w1471) -> (number=w1470:dbl)  [unwired: 3 in, 1 out]
                  n832 = Build Array (concatenate)(w1476, w1470) -> (w1475:dbl[])
                }
              }
              n833 = property on="array for data" class="Arr (strict)"("Value"=w1466) -> ()  [unwired: 2 in, 2 out]
            }
            frame #8 {
              # "check if out-of-phase\nsignal on lock-in \n(address 4) is to\nbe measured"
              n834 = property on="Addr 4 lock-in oop" class="Bool (strict)"() -> ("Value"=w1477:bool)  [unwired: 2 in, 2 out]
              n835 = property on="array for data" class="Arr (strict)"() -> ("Value"=w1479:dbl[])  [unwired: 2 in, 2 out]
              n836 = case shown="False" w1477 {
                tunnel: w1479 -> [w1480 w1488]
                tunnel: [w1480 w1487] -> w1478
                frame False {
                  # "we are not measuring out-of-phase signal on lock-in (address 4)"
                }
                frame True {
                  w1485 = "4"
                  # "we are  measuring lock-in (address 4), out-of-phase"
                  n837 = GPIB Write(0:w1485, 1:"OUTP?2") -> (6:w1486:errorcluster)  [unwired: 3 in, 1 out]
                  n838 = GPIB Read(0:w1485, 1:3200, 3:w1486) -> (5:w1483:string)  [unwired: 2 in, 2 out]
                  n839 = Fract/Exp String To Number(string=w1483) -> (number=w1482:dbl)  [unwired: 3 in, 1 out]
                  n840 = Build Array (concatenate)(w1488, w1482) -> (w1487:dbl[])
                }
              }
              n841 = property on="array for data" class="Arr (strict)"("Value"=w1478) -> ()  [unwired: 2 in, 2 out]
            }
            frame #9 {
              # "check if in-phase\nsignal on lock-in \n(address 5) is to\nbe measured"
              n842 = property on="Addr 5 lock-in" class="Bool (strict)"() -> ("Value"=w1489:bool)  [unwired: 2 in, 2 out]
              n843 = property on="array for data" class="Arr (strict)"() -> ("Value"=w1491:dbl[])  [unwired: 2 in, 2 out]
              n844 = case shown="False" w1489 {
                tunnel: w1491 -> [w1492 w1500]
                tunnel: [w1492 w1499] -> w1490
                frame False {
                  # "we are not measuring in phase signal on lock-in (address 5)"
                }
                frame True {
                  w1497 = "5"
                  # "we are  measuring lock-in (address 5), in phase"
                  n845 = GPIB Write(0:w1497, 1:"OUTP?1") -> (6:w1498:errorcluster)  [unwired: 3 in, 1 out]
                  n846 = GPIB Read(0:w1497, 1:3200, 3:w1498) -> (5:w1495:string)  [unwired: 2 in, 2 out]
                  n847 = Fract/Exp String To Number(string=w1495) -> (number=w1494:dbl)  [unwired: 3 in, 1 out]
                  n848 = Build Array (concatenate)(w1500, w1494) -> (w1499:dbl[])
                }
              }
              n849 = property on="array for data" class="Arr (strict)"("Value"=w1490) -> ()  [unwired: 2 in, 2 out]
            }
            frame #10 {
              # "check if out-of-phase\nsignal on lock-in \n(address 5) is to\nbe measured"
              n850 = property on="Addr 5 lock-in oop" class="Bool (strict)"() -> ("Value"=w1501:bool)  [unwired: 2 in, 2 out]
              n851 = property on="array for data" class="Arr (strict)"() -> ("Value"=w1503:dbl[])  [unwired: 2 in, 2 out]
              n852 = case shown="False" w1501 {
                tunnel: w1503 -> [w1504 w1512]
                tunnel: [w1504 w1511] -> w1502
                frame False {
                  # "we are not measuring out-of-phase signal on lock-in (address 5)"
                }
                frame True {
                  w1509 = "5"
                  # "we are  measuring lock-in (address 5), out-of-phase"
                  n853 = GPIB Write(0:w1509, 1:"OUTP?2") -> (6:w1510:errorcluster)  [unwired: 3 in, 1 out]
                  n854 = GPIB Read(0:w1509, 1:3200, 3:w1510) -> (5:w1507:string)  [unwired: 2 in, 2 out]
                  n855 = Fract/Exp String To Number(string=w1507) -> (number=w1506:dbl)  [unwired: 3 in, 1 out]
                  n856 = Build Array (concatenate)(w1512, w1506) -> (w1511:dbl[])
                }
              }
              n857 = property on="array for data" class="Arr (strict)"("Value"=w1502) -> ()  [unwired: 2 in, 2 out]
            }
            frame #11 {
              # "check if voltage on \nChannel A of main\nKeithley 2614B \n(addr. 12) is to\nbe measured"
              n858 = property on="Voltage (Vk1)" class="Bool (strict)"() -> ("Value"=w1513:bool)  [unwired: 2 in, 2 out]
              n859 = property on="array for data" class="Arr (strict)"() -> ("Value"=w1515:dbl[])  [unwired: 2 in, 2 out]
              n860 = case shown="False" w1513 {
                tunnel: w1515 -> [w1516 w1524]
                tunnel: [w1516 w1523] -> w1514
                frame False {
                  # "we aren't measuring voltage \non main Keithley 2614B Channel A (addr. 12)"
                }
                frame True {
                  (unwired) 13
                  w1521 = "12"
                  # "we are measuring voltage of Channel A \non the main Keithley 2614B (addr. 12)"
                  n861 = GPIB Write(0:w1521, 1:"print(smua.measure.v())") -> (6:w1522:errorcluster)  [unwired: 3 in, 1 out]
                  n862 = GPIB Read(0:w1521, 1:3200, 3:w1522) -> (5:w1517:string)  [unwired: 2 in, 2 out]
                  n863 = Fract/Exp String To Number(string=w1517) -> (number=w1519:dbl)  [unwired: 3 in, 1 out]
                  n864 = Build Array (concatenate)(w1524, w1519) -> (w1523:dbl[])
                }
              }
              n865 = property on="array for data" class="Arr (strict)"("Value"=w1514) -> ()  [unwired: 2 in, 2 out]
            }
            frame #12 {
              # "check if current on \nChannel A of main\nKeithley 2614B \n(addr. 12) is to\nbe measured"
              n866 = property on="Current (Ik1)" class="Bool (strict)"() -> ("Value"=w1525:bool)  [unwired: 2 in, 2 out]
              n867 = property on="array for data" class="Arr (strict)"() -> ("Value"=w1527:dbl[])  [unwired: 2 in, 2 out]
              n868 = case shown="True" w1525 {
                tunnel: w1527 -> [w1528 w1530]
                tunnel: [w1528 w1529] -> w1526
                frame False {
                  # "we aren't measuring current \non main Keithley 2400 (addr. 12)"
                }
                frame True {
                  w1535 = "12"
                  # "we are measuring current of Channel A \non the main Keithley 2614B (addr. 12)"
                  n869 = GPIB Write(0:w1535, 1:"print(smua.measure.i())") -> (6:w1536:errorcluster)  [unwired: 3 in, 1 out]
                  n870 = GPIB Read(0:w1535, 1:3200, 3:w1536) -> (5:w1531:string)  [unwired: 2 in, 2 out]
                  n871 = Fract/Exp String To Number(string=w1531) -> (number=w1533:dbl)  [unwired: 3 in, 1 out]
                  n872 = Build Array (concatenate)(w1530, w1533) -> (w1529:dbl[])
                }
              }
              n873 = property on="array for data" class="Arr (strict)"("Value"=w1526) -> ()  [unwired: 2 in, 2 out]
            }
            frame #13 {
              # "check if voltage on \nChannel B of main\nKeithley 2614B \n(addr. 12) is to\nbe measured"
              n874 = property on="Voltage (Vk2)" class="Bool (strict)"() -> ("Value"=w1537:bool)  [unwired: 2 in, 2 out]
              n875 = property on="array for data" class="Arr (strict)"() -> ("Value"=w1539:dbl[])  [unwired: 2 in, 2 out]
              n876 = case shown="False" w1537 {
                tunnel: w1539 -> [w1540 w1542]
                tunnel: [w1540 w1541] -> w1538
                frame False {
                  # "we aren't measuring voltage \non additional Keithley 2400 (addr. 13)"
                }
                frame True {
                  w1547 = "12"
                  # "we are measuring voltage of Channel B \non the main Keithley 2614B (addr. 12)"
                  n877 = GPIB Write(0:w1547, 1:"print(smub.measure.v())") -> (6:w1548:errorcluster)  [unwired: 3 in, 1 out]
                  n878 = GPIB Read(0:w1547, 1:3200, 3:w1548) -> (5:w1543:string)  [unwired: 2 in, 2 out]
                  n879 = Fract/Exp String To Number(string=w1543) -> (number=w1545:dbl)  [unwired: 3 in, 1 out]
                  n880 = Build Array (concatenate)(w1542, w1545) -> (w1541:dbl[])
                }
              }
              n881 = property on="array for data" class="Arr (strict)"("Value"=w1538) -> ()  [unwired: 2 in, 2 out]
            }
            frame #14 {
              # "check if current on \nChannel B of main\nKeithley 2614B \n(addr. 12) is to\nbe measured"
              n882 = property on="Current (Ik2)" class="Bool (strict)"() -> ("Value"=w1549:bool)  [unwired: 2 in, 2 out]
              n883 = property on="array for data" class="Arr (strict)"() -> ("Value"=w1551:dbl[])  [unwired: 2 in, 2 out]
              n884 = case shown="False" w1549 {
                tunnel: w1551 -> [w1552 w1554]
                tunnel: [w1552 w1553] -> w1550
                frame False {
                  # "we aren't measuring current \non additional Keithley 2400 (addr. 13)"
                }
                frame True {
                  w1559 = "12"
                  # "we are measuring current of Channel B \non the main Keithley 2614B (addr. 12)"
                  n885 = GPIB Write(0:w1559, 1:"print(smub.measure.i())") -> (6:w1560:errorcluster)  [unwired: 3 in, 1 out]
                  n886 = GPIB Read(0:w1559, 1:3200, 3:w1560) -> (5:w1555:string)  [unwired: 2 in, 2 out]
                  n887 = Fract/Exp String To Number(string=w1555) -> (number=w1557:dbl)  [unwired: 3 in, 1 out]
                  n888 = Build Array (concatenate)(w1554, w1557) -> (w1553:dbl[])
                }
              }
              n889 = property on="array for data" class="Arr (strict)"("Value"=w1550) -> ()  [unwired: 2 in, 2 out]
            }
            frame #15 {
              # "check if voltage on \nadd. Keithley 2400 \n(addr. 14) is to\nbe measured"
              n890 = property on="Voltage (Vk3)" class="Bool (strict)"() -> ("Value"=w1561:bool)  [unwired: 2 in, 2 out]
              n891 = property on="array for data" class="Arr (strict)"() -> ("Value"=w1563:dbl[])  [unwired: 2 in, 2 out]
              n892 = case shown="False" w1561 {
                tunnel: w1563 -> [w1564 w1574]
                tunnel: [w1564 w1573] -> w1562
                frame False {
                  # "we aren't measuring voltage \non additional Keithley 2400 (addr. 14)"
                }
                frame True {
                  w1571 = "14"
                  # "we are measuring voltage \non additional Keithley 2400 (addr. 14)"
                  n893 = GPIB Write(0:w1571, 1:":READ?") -> (6:w1572:errorcluster)  [unwired: 3 in, 1 out]
                  n894 = GPIB Read(0:w1571, 1:3200, 3:w1572) -> (5:w1567:string)  [unwired: 2 in, 2 out]
                  n895 = String Subset(string=w1567, length (rest)=13) -> (substring=w1566:string)  [unwired: 1 in]
                  n896 = Fract/Exp String To Number(string=w1566) -> (number=w1569:dbl)  [unwired: 3 in, 1 out]
                  n897 = Build Array (concatenate)(w1574, w1569) -> (w1573:dbl[])
                }
              }
              n898 = property on="array for data" class="Arr (strict)"("Value"=w1562) -> ()  [unwired: 2 in, 2 out]
            }
            frame #16 {
              # "check if  current on \nadd. Keithley 2400 \n(addr. 14) is to\nbe measured"
              n899 = property on="Current (Ik3)" class="Bool (strict)"() -> ("Value"=w1575:bool)  [unwired: 2 in, 2 out]
              n900 = property on="array for data" class="Arr (strict)"() -> ("Value"=w1577:dbl[])  [unwired: 2 in, 2 out]
              n901 = case shown="False" w1575 {
                tunnel: w1577 -> [w1578 w1589]
                tunnel: [w1578 w1588] -> w1576
                frame False {
                  # "we aren't measuring current \non additional Keithley 2400 (addr. 14)"
                }
                frame True {
                  w1586 = "14"
                  # "we are measuring current\non additional Keithley 2400 (addr. 14)"
                  n902 = GPIB Write(0:w1586, 1:":READ?") -> (6:w1587:errorcluster)  [unwired: 3 in, 1 out]
                  n903 = GPIB Read(0:w1586, 1:3200, 3:w1587) -> (5:w1582:string)  [unwired: 2 in, 2 out]
                  n904 = String Subset(string=w1582, offset (0)=14, length (rest)=13) -> (substring=w1581:string)
                  n905 = Fract/Exp String To Number(string=w1581) -> (number=w1584:dbl)  [unwired: 3 in, 1 out]
                  n906 = Build Array (concatenate)(w1589, w1584) -> (w1588:dbl[])
                }
              }
              n907 = property on="array for data" class="Arr (strict)"("Value"=w1576) -> ()  [unwired: 2 in, 2 out]
            }
            frame #17 {
              # "check if 1st channel\non Keithley 2182 \n(addr. 15) is to\nbe measured"
              n908 = property on="Channel 1 (Vnano1)" class="Bool (strict)"() -> ("Value"=w1590:bool)  [unwired: 2 in, 2 out]
              n909 = property on="array for data" class="Arr (strict)"() -> ("Value"=w1592:dbl[])  [unwired: 2 in, 2 out]
              n910 = case shown="True" w1590 {
                tunnel: w1592 -> [w1593 w1601]
                tunnel: [w1593 w1600] -> w1591
                frame False {
                  # "we are not measuring 1st channel\non Keithley 2182 (addr. 15)"
                }
                frame True {
                  w1598 = "15"
                  # "we are measuring 1st channel\non Keithley 2182 (addr. 15)"
                  n911 = GPIB Write(0:w1598, 1:":SENSe:DATA:FRES?") -> (6:w1599:errorcluster)  [unwired: 3 in, 1 out]
                  n912 = GPIB Read(0:w1598, 1:200, 3:w1599) -> (5:w1594:string)  [unwired: 2 in, 2 out]
                  n913 = Fract/Exp String To Number(string=w1594) -> (number=w1596:dbl)  [unwired: 3 in, 1 out]
                  n914 = Build Array (concatenate)(w1601, w1596) -> (w1600:dbl[])
                }
              }
              n915 = property on="array for data" class="Arr (strict)"("Value"=w1591) -> ()  [unwired: 2 in, 2 out]
            }
            frame #18 {
              # "check if 2nd channel\non Keithley 2182 \n(addr. 15) is to\nbe measured"
              n916 = property on="Channel 2 (Vnano1b)" class="Bool (strict)"() -> ("Value"=w1602:bool)  [unwired: 2 in, 2 out]
              n917 = property on="array for data" class="Arr (strict)"() -> ("Value"=w1604:dbl[])  [unwired: 2 in, 2 out]
              n918 = case shown="False" w1602 {
                tunnel: w1604 -> [w1605 w1617]
                tunnel: [w1605 w1616] -> w1603
                frame False {
                  # "we are not measuring 1st channel\non Keithley 2182 (addr. 15)"
                }
                frame True {
                  w1608 = "15"
                  # "switching to channel 2 and then\nback to channel 1"
                  # "we are measuring 2nd channel\non Keithley 2182 (addr. 15)"
                  n919 = GPIB Write(0:w1608, 1:":SENSe:CHAN 2") -> (6:w1609:errorcluster)  [unwired: 3 in, 1 out]
                  n920 = GPIB Write(0:w1608, 1:":SENSe:DATA:FRES?", 3:w1609) -> (6:w1615:errorcluster)  [unwired: 2 in, 1 out]
                  n921 = GPIB Read(0:w1608, 1:200, 3:w1615) -> (5:w1611:string, 7:w1607:errorcluster)  [unwired: 2 in, 1 out]
                  n922 = GPIB Write(0:w1608, 1:":SENSe:CHAN 1", 3:w1607) -> ()  [unwired: 2 in, 2 out]
                  n923 = Fract/Exp String To Number(string=w1611) -> (number=w1613:dbl)  [unwired: 3 in, 1 out]
                  n924 = Build Array (concatenate)(w1617, w1613) -> (w1616:dbl[])
                }
              }
              n925 = property on="array for data" class="Arr (strict)"("Value"=w1603) -> ()  [unwired: 2 in, 2 out]
            }
            frame #19 {
              # "check if 1st channel\non Keithley 2182 \n(addr. 16) is to\nbe measured"
              n926 = property on="Channel 1 (Vnano2)" class="Bool (strict)"() -> ("Value"=w1618:bool)  [unwired: 2 in, 2 out]
              n927 = property on="array for data" class="Arr (strict)"() -> ("Value"=w1620:dbl[])  [unwired: 2 in, 2 out]
              n928 = case shown="True" w1618 {
                tunnel: w1620 -> [w1621 w1629]
                tunnel: [w1621 w1628] -> w1619
                frame False {
                  # "we are not measuring 1st channel\non Keithley 2182 (addr. 16)"
                }
                frame True {
                  w1626 = "16"
                  # "we are measuring 1st channel\non Keithley 2182 (addr. 16)"
                  n929 = GPIB Write(0:w1626, 1:":SENSe:DATA:FRES?") -> (6:w1627:errorcluster)  [unwired: 3 in, 1 out]
                  n930 = GPIB Read(0:w1626, 1:200, 3:w1627) -> (5:w1622:string)  [unwired: 2 in, 2 out]
                  n931 = Fract/Exp String To Number(string=w1622) -> (number=w1624:dbl)  [unwired: 3 in, 1 out]
                  n932 = Build Array (concatenate)(w1629, w1624) -> (w1628:dbl[])
                }
              }
              n933 = property on="array for data" class="Arr (strict)"("Value"=w1619) -> ()  [unwired: 2 in, 2 out]
            }
            frame #20 {
              # "check if 2nd channel\non Keithley 2182 \n(addr. 16) is to\nbe measured"
              n934 = property on="Channel 2 (Vnano2b)" class="Bool (strict)"() -> ("Value"=w1630:bool)  [unwired: 2 in, 2 out]
              n935 = property on="array for data" class="Arr (strict)"() -> ("Value"=w1632:dbl[])  [unwired: 2 in, 2 out]
              n936 = case shown="False" w1630 {
                tunnel: w1632 -> [w1633 w1645]
                tunnel: [w1633 w1644] -> w1631
                frame False {
                  # "we are not measuring 1st channel\non Keithley 2182 (addr. 16)"
                }
                frame True {
                  w1636 = "16"
                  # "switching to channel 2 and then\nback to channel 1"
                  # "we are measuring 2nd channel\non Keithley 2182 (addr. 16)"
                  n937 = GPIB Write(0:w1636, 1:":SENSe:CHAN 2") -> (6:w1637:errorcluster)  [unwired: 3 in, 1 out]
                  n938 = GPIB Write(0:w1636, 1:":SENSe:DATA:FRES?", 3:w1637) -> (6:w1643:errorcluster)  [unwired: 2 in, 1 out]
                  n939 = GPIB Read(0:w1636, 1:200, 3:w1643) -> (5:w1639:string, 7:w1635:errorcluster)  [unwired: 2 in, 1 out]
                  n940 = GPIB Write(0:w1636, 1:":SENSe:CHAN 1", 3:w1635) -> ()  [unwired: 2 in, 2 out]
                  n941 = Fract/Exp String To Number(string=w1639) -> (number=w1641:dbl)  [unwired: 3 in, 1 out]
                  n942 = Build Array (concatenate)(w1645, w1641) -> (w1644:dbl[])
                }
              }
              n943 = property on="array for data" class="Arr (strict)"("Value"=w1631) -> ()  [unwired: 2 in, 2 out]
            }
            frame #21 {
              # "check if 1st channel\non Keithley 2182 \n(addr. 17) is to\nbe measured"
              n944 = property on="Channel 1 (Vnano3)" class="Bool (strict)"() -> ("Value"=w1646:bool)  [unwired: 2 in, 2 out]
              n945 = property on="array for data" class="Arr (strict)"() -> ("Value"=w1648:dbl[])  [unwired: 2 in, 2 out]
              n946 = case shown="False" w1646 {
                tunnel: w1648 -> [w1649 w1657]
                tunnel: [w1649 w1656] -> w1647
                frame False {
                  # "we are not measuring 1st channel\non Keithley 2182 (addr. 17)"
                }
                frame True {
                  w1654 = "17"
                  # "we are measuring 1st channel\non Keithley 2182 (addr. 17)"
                  n947 = GPIB Write(0:w1654, 1:":SENSe:DATA:FRES?") -> (6:w1655:errorcluster)  [unwired: 3 in, 1 out]
                  n948 = GPIB Read(0:w1654, 1:200, 3:w1655) -> (5:w1650:string)  [unwired: 2 in, 2 out]
                  n949 = Fract/Exp String To Number(string=w1650) -> (number=w1652:dbl)  [unwired: 3 in, 1 out]
                  n950 = Build Array (concatenate)(w1657, w1652) -> (w1656:dbl[])
                }
              }
              n951 = property on="array for data" class="Arr (strict)"("Value"=w1647) -> ()  [unwired: 2 in, 2 out]
            }
            frame #22 {
              # "check if 2nd channel\non Keithley 2182 \n(addr. 17) is to\nbe measured"
              n952 = property on="Channel 2 (Vnano3b)" class="Bool (strict)"() -> ("Value"=w1658:bool)  [unwired: 2 in, 2 out]
              n953 = property on="array for data" class="Arr (strict)"() -> ("Value"=w1660:dbl[])  [unwired: 2 in, 2 out]
              n954 = case shown="False" w1658 {
                tunnel: w1660 -> [w1661 w1673]
                tunnel: [w1661 w1672] -> w1659
                frame False {
                  # "we are not measuring 1st channel\non Keithley 2182 (addr. 17)"
                }
                frame True {
                  w1664 = "17"
                  # "switching to channel 2 and then\nback to channel 1"
                  # "we are measuring 2nd channel\non Keithley 2182 (addr. 17)"
                  n955 = GPIB Write(0:w1664, 1:":SENSe:CHAN 2") -> (6:w1665:errorcluster)  [unwired: 3 in, 1 out]
                  n956 = GPIB Write(0:w1664, 1:":SENSe:DATA:FRES?", 3:w1665) -> (6:w1671:errorcluster)  [unwired: 2 in, 1 out]
                  n957 = GPIB Read(0:w1664, 1:200, 3:w1671) -> (5:w1667:string, 7:w1663:errorcluster)  [unwired: 2 in, 1 out]
                  n958 = GPIB Write(0:w1664, 1:":SENSe:CHAN 1", 3:w1663) -> ()  [unwired: 2 in, 2 out]
                  n959 = Fract/Exp String To Number(string=w1667) -> (number=w1669:dbl)  [unwired: 3 in, 1 out]
                  n960 = Build Array (concatenate)(w1673, w1669) -> (w1672:dbl[])
                }
              }
              n961 = property on="array for data" class="Arr (strict)"("Value"=w1659) -> ()  [unwired: 2 in, 2 out]
            }
            frame #23 {
              # "check if 1st \nthermometer on \nOxford ITC \n(address 24) \nis measured"
              n962 = property on="Thermometer 1 (T1)" class="Bool (strict)"() -> ("Value"=w1674:bool)  [unwired: 2 in, 2 out]
              n963 = property on="array for data" class="Arr (strict)"() -> ("Value"=w1676:dbl[])  [unwired: 2 in, 2 out]
              n964 = case shown="True" w1674 {
                tunnel: w1676 -> [w1677 w1689]
                tunnel: [w1677 w1688] -> w1675
                frame False {
                  # "we are not measuring temperature on\nthermometer 1 (addr. 24)"
                }
                frame True {
                  (unwired) "\r"
                  w1682 = refnum<visa-resource-name> "TCPIP0::192.168.128.2::7020::SOCKET" ("VISA resource name")
                  # "we are measuring temperature,\nthermometer 1 (addr. 24)"
                  n965 = Concatenate Strings("READ:DEV:MB1.T1:TEMP:SIG:TEMP" ("string"), "\n") -> (w1681:string)
                  n966 = VISA Write(VISA resource name=w1682, write buffer=w1681) -> (error out=w1687:errorcluster)  [unwired: 1 in, 2 out]
                  n967 = String Length(string=w1681) -> (length=w1678:i32)
                  n968 = VISA Read(VISA resource name=w1682, byte count=1024, error in (no error)=w1687) -> (read buffer=w1685:string)  [unwired: 3 out]
                  n969 = String Subset(string=w1685, offset (0)=w1678) -> (substring=w1684:string)  [unwired: 1 in]
                  n970 = Fract/Exp String To Number(string=w1684) -> (number=w1680:dbl)  [unwired: 3 in, 1 out]
                  n971 = Build Array (concatenate)(w1689, w1680) -> (w1688:dbl[])
                }
              }
              n972 = property on="array for data" class="Arr (strict)"("Value"=w1675) -> ()  [unwired: 2 in, 2 out]
            }
            frame #24 {
              # "check if 1st \nthermometer on \nOxford ITC \n(address 24) \nis measured"
              n973 = property on="Magnetic Field (B)" class="Bool (strict)"() -> ("Value"=w1690:bool)  [unwired: 2 in, 2 out]
              n974 = property on="array for data" class="Arr (strict)"() -> ("Value"=w1692:dbl[])  [unwired: 2 in, 2 out]
              n975 = case shown="True" w1690 {
                tunnel: w1692 -> [w1693 w1705]
                tunnel: [w1693 w1704] -> w1691
                frame False {
                  # "we are not measuringmagnetic field (addr. 25)"
                }
                frame True {
                  (unwired) "\r"
                  w1698 = refnum<visa-resource-name> "TCPIP0::192.168.128.3::7020::SOCKET" ("VISA resource name")
                  # "we are measuring magnetic field  (addr. 25)"
                  n976 = Concatenate Strings("READ:DEV:GRPZ:PSU:SIG:FLD" ("string"), "\n") -> (w1697:string)
                  n977 = VISA Write(VISA resource name=w1698, write buffer=w1697) -> (error out=w1703:errorcluster)  [unwired: 1 in, 2 out]
                  n978 = String Length(string=w1697) -> (length=w1694:i32)
                  n979 = VISA Read(VISA resource name=w1698, byte count=1024, error in (no error)=w1703) -> (read buffer=w1701:string)  [unwired: 3 out]
                  n980 = String Subset(string=w1701, offset (0)=w1694) -> (substring=w1700:string)  [unwired: 1 in]
                  n981 = Fract/Exp String To Number(string=w1700) -> (number=w1696:dbl)  [unwired: 3 in, 1 out]
                  n982 = Build Array (concatenate)(w1705, w1696) -> (w1704:dbl[])
                }
              }
              n983 = property on="array for data" class="Arr (strict)"("Value"=w1691) -> ()  [unwired: 2 in, 2 out]
            }
            frame #25 {
              # "check if capacitance\nand loss (address 28)\nare measured"
              n984 = property on="Capacitance (C) and Loss (L)" class="Bool (strict)"() -> ("Value"=w1706:bool)  [unwired: 2 in, 2 out]
              n985 = property on="array for data" class="Arr (strict)"() -> ("Value"=w1708:dbl[])  [unwired: 2 in, 2 out]
              n986 = case shown="False" w1706 {
                tunnel: w1708 -> [w1709 w1715]
                tunnel: [w1709 w1711] -> w1707
                frame False {
                  # "we are not measuringmagnetic capacitance (addr. 28)"
                }
                frame True {
                  # "we are measuring capacitance and loss  (addr. 28)"
                  n987 = stacked-sequence {
                    seq-local: [w1717 _ _] -> [_ _ w1740]
                    tunnel: [_ _ w1734] -> w1710
                    tunnel: [_ _ w1735] -> w1713
                    tunnel: "28" ("data") -> [w1716 w1720 w1729]
                    frame #0 {
                      n988 = GPIB Write(0:w1716, 1:"SINGLE" ("data"), 2:i16 0 ("mode (0)")) -> (6:w1717:errorcluster)  [unwired: 2 in, 1 out]
                    }
                    frame #1 {
                      n989 = while {
                        tunnel: w1720 -> [w1721]
                        i -> [w1722]
                        stop <- w1724 continue-if-true
                        n990 = GPIB Serial Poll(0:w1721) -> (2:w1726:i16)  [unwired: 1 in, 2 out]
                        n991 = Less?(x=w1726, y=i16 128) -> (x < y?=w1724:bool)
                        n992 = Wait (ms)(milliseconds to wait=u32 50) -> ()  [unwired: 1 out]
                        "Numeric 3" <- w1722
                      }
                    }
                    frame #2 {
                      w1727 = i16 2 ("mode (0)")
                      n993 = GPIB Read(0:w1729, 1:200 ("byte count"), 2:i16 2 ("mode (0)"), 3:w1740) -> (5:w1733:string)  [unwired: 1 in, 2 out]
                      n994 = Match Pattern(string=w1733, regular expression="C=") -> (after substring=w1732:string)  [unwired: 1 in, 3 out]
                      n995 = Match Pattern(string=w1732, regular expression="PF L=") -> (after substring=w1730:string)  [unwired: 1 in, 3 out]
                      n996 = Search/Split String(string=w1732, search string/char (-)=" ", offset (0)=w1727) -> (substring before match=w1737:string)  [unwired: 2 out]
                      n997 = Search/Split String(string=w1730, search string/char (-)=" ", offset (0)=w1727) -> (substring before match=w1736:string)  [unwired: 2 out]
                      n998 = Fract/Exp String To Number(string=w1736) -> (number=w1734:dbl)  [unwired: 3 in, 1 out]
                      n999 = Fract/Exp String To Number(string=w1737) -> (number=w1735:dbl)  [unwired: 3 in, 1 out]
                    }
                  }
                  n1000 = Build Array (concatenate)(w1715, w1713) -> (w1712:dbl[])
                  n1001 = Build Array (concatenate)(w1712, w1710) -> (w1711:dbl[])
                }
              }
              n1002 = property on="array for data" class="Arr (strict)"("Value"=w1707) -> ()  [unwired: 2 in, 2 out]
            }
          }
        }
      }
      n1003 = property on="array for data" class="Arr (strict)"(error in=w571) -> ("Value"=w549:dbl[])  [unwired: 1 in, 2 out]
      n1004 = while {
        shift-right: [w1754] -> w545
        shift-left: w549 -> [w1756]
        i -> [w1755]
        stop <- w1759 stop-if-true
        # "loop goes through the list of all measured parameters\nif some columns are identified as current or resistance\nthey are recalculated according to selected or entered parameters"
        n1005 = Increment(x=w1755) -> (x+1=w1760:i32)
        n1006 = property on="Ring" class="Ring (strict)"() -> ("Strings []"=w1758:string[])  [unwired: 2 in, 2 out]
        n1007 = Index Array(array=w1758, index=w1755) -> (element=w1757:string)
        n1008 = property on="Ring" class="Ring (strict)"() -> ("NumItems"=w1761:u32)  [unwired: 2 in, 2 out]
        n1009 = case shown="\"False\", Default" w1757 {
          tunnel: w1756 -> [w1767 w1777 w1787 w1794]
          tunnel: w1755 -> [w1765 w1774 w1785 _]
          tunnel: [w1766 w1775 w1786 w1794] -> w1754
          frame "I" {
            n1010 = property on="Current is:" class="RadioBtnsControl (strict)"() -> ("Value"=w1763:T1)  [unwired: 2 in, 2 out]
            n1011 = case shown="\"Radio Selection 2\"" w1763 {
              tunnel: ["Ring 3" "Ring 2"] -> w1762
              frame "Radio Selection 3", Default {
              }
              frame "Radio Selection 2" {
              }
            }
            n1012 = Index Array(array=w1767, index=w1765) -> (element=w1768:dbl)
            n1013 = Power Of 10(x=w1762) -> (10^x=w1771:dbl)
            n1014 = Multiply(x=1000.0, y=w1771) -> (x*y=w1769:dbl)
            n1015 = Divide(x=w1768, y=w1769) -> (x/y=w1764:dbl)
            "Numeric Current" <- w1764
            n1016 = Replace Array Subset(array=w1767, new element=w1764, index=w1765) -> (w1766:dbl[])
          }
          frame "Ioop" {
            n1017 = property on="Ring 3" class="Ring (strict)"() -> ("Value"=w1776:u16)  [unwired: 2 in, 2 out]
            n1018 = Index Array(array=w1777, index=w1774) -> (element=w1779:dbl)
            n1019 = Power Of 10(x=w1776) -> (10^x=w1782:dbl)
            n1020 = Multiply(x=1000.0, y=w1782) -> (x*y=w1780:dbl)
            n1021 = Divide(x=w1779, y=w1780) -> (x/y=w1778:dbl)
            n1022 = Replace Array Subset(array=w1777, new element=w1778, index=w1774) -> (w1775:dbl[])
          }
          frame "R1", "R1oop", "R2", "R2oop", "R3", "R3oop", "R4", "R4oop", "R5", "R5oop" {
            n1023 = property on="Current is:" class="RadioBtnsControl (strict)"() -> ("Value"=w1784:T1)  [unwired: 2 in, 2 out]
            n1024 = case shown="\"Radio Selection 2\", Default" w1784 {
              tunnel: [w1790 w1793] -> w1783
              frame "Radio Selection 1" {
                n1025 = Divide(x="Fixed Current mkA", y=1000000.0) -> (x/y=w1790:dbl)
              }
              frame "Radio Selection 2", Default {
                n1026 = property on="Numeric Current" class="DigNum (strict)"() -> ("Value"=w1793:dbl)  [unwired: 2 in, 2 out]
              }
            }
            n1027 = Index Array(array=w1787, index=w1785) -> (element=w1789:dbl)
            n1028 = Divide(x=w1789, y=w1783) -> (x/y=w1788:dbl)
            n1029 = Replace Array Subset(array=w1787, new element=w1788, index=w1785) -> (w1786:dbl[])
          }
          frame "False", Default {
          }
        }
        n1030 = Less?(x=w1761, y=w1760) -> (x < y?=w1759:bool)
      }
      n1031 = Subtract(x="Target Voltage, V", y=w555) -> (x-y=w558:dbl)
      n1032 = Divide(x="Sweep rate, V/min", y=60.0) -> (x/y=w567:dbl)
      n1033 = Multiply(x=w567, y="Time btw \npoints, sec") -> (x*y=w550:dbl)
      n1034 = Sign(1:w558) -> (0:w551:dbl)
      n1035 = Multiply(x=w551, y=w550) -> (x*y=w543:dbl)
      n1036 = property on="points at each Vg" class="DigNum (strict)"() -> ("Value"=w542:i32)  [unwired: 2 in, 2 out]
      n1037 = To Double Precision Float(number=w542) -> (double precision float=w541:dbl)
      n1038 = Multiply(x=w541, y=w543) -> (x*y=w540:dbl)
      n1039 = property on="Commutator" class="Bool (strict)"() -> ("Value"=w534:bool)  [unwired: 2 in, 2 out]
      n1040 = property on="Data file:" class="Path"() -> ("Value"=w547:path)  [unwired: 2 in, 2 out]
      n1041 = Divide(x=w558, y=w540) -> (x/y=w565:dbl)
      n1042 = case shown="False" w534 {
        tunnel: w552 -> [w585 w596]
        tunnel: w536 -> [w580 w590]
        tunnel: [w572 w589] -> w533
        frame True {
          # "calculate deliberate time delay for the next step"
          n1043 = Subtract(x=w585, y=w580) -> (x-y=w578:u32)
          n1044 = property on="Delib Time delay" class="DigNum (strict)"() -> ("Value"=w579:i32)  [unwired: 2 in, 2 out]
          n1045 = property on="Time btw \npoints, sec" class="DigNum (strict)"() -> ("Value"=w584:dbl)  [unwired: 2 in, 2 out]
          n1046 = Subtract(x=w578, y=w579) -> (x-y=w577:u32)
          n1047 = Multiply(x=w584, y=1000.0) -> (x*y=w582:dbl)
          n1048 = To Long Integer(number=w582) -> (32bit integer=w581:i32)
          n1049 = Greater?(x=w581, y=w577) -> (0:w574:bool)
          n1050 = Subtract(x=w581, y=w577) -> (x-y=w576:u32)
          n1051 = Divide(x=w576, y=2) -> (x/y=w573:dbl)
          n1052 = case shown="False" w574 {
            tunnel: w573 -> [_ w588]
            tunnel: [0 w587] -> w572
            frame False {
            }
            frame True {
              n1053 = To Long Integer(number=w588) -> (32bit integer=w587:i32)
            }
          }
        }
        frame False {
          # "calculate deliberate time delay for the next step"
          n1054 = Subtract(x=w596, y=w590) -> (x-y=w593:u32)
          n1055 = property on="Time btw \npoints, sec" class="DigNum (strict)"() -> ("Value"=w595:dbl)  [unwired: 2 in, 2 out]
          n1056 = Multiply(x=w595, y=1000.0) -> (x*y=w592:dbl)
          n1057 = To Long Integer(number=w592) -> (32bit integer=w591:i32)
          n1058 = Greater?(x=w591, y=w593) -> ()  [unwired: 1 out]
          n1059 = Subtract(x=w591, y=w593) -> (x-y=w589:u32)
        }
      }
      "Delib Time delay" <- w533
      n1060 = Decrement(x=w565) -> (x-1=w564:dbl)
      n1061 = Absolute Value(x=w558) -> (abs(x)=w560:dbl)
      n1062 = Build Array (concatenate)(w570, w545) -> (w544:dbl[][])
      n1063 = Greater Than 0?(x=w564) -> (x > 0?=w563:bool)
      n1064 = property on="array for data" class="Arr (strict)"("Value"=w545) -> ()  [unwired: 2 in, 2 out]
      n1065 = call-poly <vilib>:"Write To Spreadsheet File.vi"("format (%.3f)"="%#g", "append to file? (new file:F)"=TRUE, "1D data"=w545, "file path (dialog if empty)"=w547) -> ()  [unwired: 4 in, 1 out]
      n1066 = Less?(x=w560, y=1e-06) -> (x < y?=w557:bool)
      n1067 = flat-sequence {
        tunnel: [w1753] -> w552
        tunnel: w544 -> [w1747]
        frame #0 {
          # "time is mesured at the end of the cycle\nto adjust a delay time"
          # "this part plots selected measurements"
          n1068 = Tick Count (ms)() -> (millisecond timer value=w1753:u32)
          n1069 = Index Array(array=w1747, index (col)="Ring") -> (element=w1752:dbl[])  [unwired: 1 in]
          n1070 = Index Array(array=w1747, index (col)=0) -> (element=w1750:dbl[])  [unwired: 1 in]
          n1071 = Bundle(w1750, w1752) -> (→"XY Graph":cluster{dbl[], dbl[]})  [unwired: 1 in]
        }
      }
      n1072 = case shown="True" w563 {
        tunnel: w555 -> [_ w1798]
        tunnel: w540 -> [_ w1797]
        tunnel: [w1795 w1796] -> w562
        frame False {
          # "if next step is too long\nuse target voltage"
          n1073 = property on="Target Voltage, V" class="DigNum (strict)"() -> ("Value"=w1795:dbl)  [unwired: 2 in, 2 out]
        }
        frame True {
          # "add increment to\nthe current Vg"
          n1074 = Add(x=w1797, y=w1798) -> (x+y=w1796:dbl)
        }
      }
    }
    n1075 = Number To Fractional String(number=w512) -> (F-format string=w517:string)  [unwired: 3 in]
    n1076 = property on="Main Keithly2614B address" class="Str"() -> ("Value"=w515:string)  [unwired: 2 in, 2 out]
    n1077 = Concatenate Strings("smua.source.levelv = " ("data"), w517) -> (w516:string)
    n1078 = Equal?(x=w510, y="optional Bias (V)") -> (x = y?=w513:bool)
    n1079 = case shown="True" w513 {
      tunnel: "optional Bias (V)" -> [w524 _]
      tunnel: w512 -> [w525 _]
      frame False {
        n1080 = Multiply(x=w525, y=22.62) -> (x*y=w526:dbl)
        n1081 = Number To Fractional String(number=w524) -> (F-format string=w532:string)  [unwired: 3 in]
        n1082 = Add(x=w524, y=w526) -> ()  [unwired: 1 out]
        n1083 = Concatenate Strings(":INIT:IMM; :SOUR:VOLT:LEV:IMM:AMPL " ("data"), w532) -> (w531:string)
        n1084 = property on="optional Bias (V)" class="DigNum (strict)"("Visible"=TRUE) -> ()  [unwired: 2 in, 2 out]
        n1085 = GPIB Write(0:"13", 1:w531) -> ()  [unwired: 3 in, 2 out]
      }
      frame True {
      }
    }
    n1086 = GPIB Write(0:w515, 1:w516) -> ()  [unwired: 3 in, 2 out]
  }
  "Array 2" <- w13
  n1087 = Write to Text File(file (use dialog)=w16, text=w15) -> ()  [unwired: 2 in, 3 out]
  n1088 = Array Size(array=w5) -> (size(s)=→"Numeric 2":i32)
  n1089 = property on="optional Bias (V)" class="DigNum (strict)"("Value"=w11, "Visible"=FALSE) -> ()  [unwired: 2 in, 2 out]
